vi "BIMS_Collector (BRZ).vi"() -> ()   [LabVIEW 2015]
doc: "This program is currently beta software. It is designed to address the data requirements defined primarily by the DHB Ballistic Test Report.\n\nThe general operation of this program is based on the Ballistics Version 2005 application developed internally by DuPont as a research tool for the Spruance Plant Ballistics Lab in Richmond, VA.\n\nPlease note that the original trigger control logic was modified and no longer depends on a safety interlock system to enable operation of a ballistic test.\n\nDuPont makes no warranties and assumes no liabilities in connection with any use of this program."
uses:
  <vilib>/addons/database/NI_Database_API.lvlib
  <vilib>/addons/database/Connection.llb/Conn Execute.vi
  <vilib>/addons/database/Recordset.llb/Rec Destroy - Connection.vi
  <vilib>/Utility/config.llb/NI_LVConfig.lvlib
  <vilib>/Utility/config.llb/Write Key (I32).vi
  Shot Record.ctl
  BIMS_Collector Globals.vi
  Collector State.ctl
  DataSource.ctl
  <vilib>/registry/registry.llb/Registry RtKey.ctl
  <vilib>/Utility/config.llb/Write Key (String).vi
  <vilib>/addons/database/Connection.llb/DB Tools Open Connec (Path).vi
panel:
  out "Loading":u16(ring)
  in  "runtimeMenusVisible":bool=TRUE
  in  "diagPageVisible":bool
  in  "RESET All":bool
  out "ConfigName":string
  out "TimeNow":string
  in  "EXIT":bool
  in  "mainTabCntrl":enum32{"Setup", "Measure", "History", "System"}(tab)=enum."System"
  in  "SampleEntryTabCntrl":enum32{"Environment", "Sample"}(tab)
  in  "ThreatDetails":u16(ring) caption="Detail" items=["2gr 223 cal.   FSP", "4gr 223 cal.   FSP", "16gr 223 cal."]
  in  "ThreatGroups":u16(ring) caption="Group" items=["", "RCC", "FSP", "44 Magnum", "0.22 Caliber", "0.380 Caliber", "0.38 Caliber", "9mm Luger", "40 S&W", "0.357 MAG", "0.44 Rem Mag"]
  in  "PowderTypes":u16(ring) caption="Type" items=["", "CBC 236", "CBC 210", "CBC 220", "CBC 216", "CBC 207", "CBC PCL 504"]
  in  "Ballisticians":u16(ring) caption="Laboratorists" items=["", "Gustavo M Rubio", "Manoel Machado", "Lucas Loureiro", "Outros (others)"]
  in  "Recorders":u16(ring) caption="Recorder"
  in  "Shooters":u16(ring) caption="Shooter" items=["", "Manoel C. Machado                                 ", "Gustavo M Rubio                                   ", "Assef Maluf                                       "]
  in  "Methods":u16(ring) caption="Method" items=["", "V50", "NIJ 0101.04", "NIJ 0101.06", "NIJ 0108.01", "Helmets", "Others"]
  in  "RoomT":sgl caption="Temperature (° C)" format="%.1f"
  in  "RoomHum":sgl caption="Humidity (%)" min=0 max=100 format="%.1f"
  in  "SampleBackings":u16(ring)=3 caption="Type" items=["", "Clay", "Roma Clay", "Corfix Clay", "Dim Clay"]
  in  "clayCalArray":i16[](array[numeric])=[0, 0, 0, 0, 0] caption="Calibration (mm)" min=0 max=99 format="%02.0f"
  out "clayAverage":sgl caption="Clay Average (mm)" format="%#.1f"
  in  "clayTemp":sgl caption="Clay Temp (° F)" format="%.1f"
  out "threatDetails":T1 caption="Description"
  in  "SampleClamping":u16(ring) caption="Clamping" items=["", "elástic with Velcro", "screws", "rubber tube", "anti spall ", "box against fragments"]
  in  "Sample SubTabCntrl":T2(tab)
  in  "SampleID":string caption="Sample ID"
  in  "SampleDimensions":u16(ring) caption="Dimensions" items=["", "40 x 40", "50 x 50", "P", "M", "G", "GG", "Car Part", "Indefinite"]
  in  "ModelMfrs":u16(ring) caption="Manufacturer" items=["DuPont Experimental"]
  in  "SampleTypes":u16(ring) caption="Sample Type" items=["", "Aramid", "Glass", "Steel", "Ceramic", "Panel", "Body Armor", "Car Parts", "Quality Control", "Helmets", "Shield", "Other"]
  in  "Submitters":u16(ring) caption="Submitter" items=["", "Ana P Viegas", "Julio Tabegna", "Priscila Akiti", "Ariana Bottura", "Carlos Magno", "Rodrigo Gomez", "Angela C Vargas", "Manoel Machado", "Others"]
  in  "ProjectID":string caption="Project ID"
  in  "BackLayers":i32 caption="# of Layers" min=0 max=99 step=5
  in  "FrontLayers":i32 caption="# of Layers" min=0 max=99 step=5
  in  "BackLayer":u16(ring) caption="Back Layer" items=["", "PC", "Steel", "PE Foam", "Ghost", "ceramic plate", "Others"]
  in  "FrontLayer":u16(ring) caption="Front Layer" items=["", "PC", "Steel", "PE Foam", "Ghost", "ceramic plate", "Others"]
  out "totalNumLayers":i32 caption="Total # of Layers" min=0 max=100 step=5
  out "totalBAW":sgl caption="Total BAW (psf)" format="%.2f"
  in  "LayerTabControl":enum32{"1", "2", "3", "4", "5", "6"}(tab) caption="Inner Layers"
  out "fab1_totalWt":sgl caption="Fab1 Wt" min=0 max=99 step=5 format="%.2f"
  out "SampleAttribs_1":T3 caption="fabricAttribs_1"
  in  "Layer_1":T4 caption="Fabric #1" {"plyNum" min=0 max=99 step=5}
  in  "SampleStyle_1":u16(ring) items=["", "S363 GR", "S363 WR", "S436 GR", "S436 WR", "S704 GR", "S704 WR", "S708 GR", "S708 WR", "S720", "S720 GR", "S720 WR", "S724 GR", "S729 GR", "S729 WR", "S731 GR", "S731 WR", "S745 GR", "S745 WR", "S745GR", "S745GR-1", "S778 GR", "S778 WR", "XF", "XP1000"]
  in  "Mfr_1":u16(ring) caption="vendor" items=["", "Assef Maluf", "DuPont", "DuPont Cooper River", "TEADIT", "TestBob1"]
  in  "layerStitch_1":u16(ring) caption="Stitch" items=["", "Diamante (diamond)", "Cantos vertices (corners vertices)", "Cantos centrais (corners centrals)", "Borda e Centro (all around and center)", "Borda (all around)", "Borda e diamante (all around and diamond)", "Dupla em X (double and X centered)", "Outras (others)"]
  out "fab2_totalWt":sgl caption="Fab2 Wt" min=0 max=99 step=5 format="%.2f"
  out "SampleAttribs_2":T3 caption="fabricAttribs_2"
  in  "Layer_2":T4 caption="Fabric #2" {"plyNum" min=0 max=99 step=5}
  in  "SampleStyle_2":u16(ring)
  in  "Mfr_2":u16(ring) caption="vendor" items=["", "Assef Maluf", "DuPont", "DuPont Cooper River", "TEADIT", "TestBob1"]
  in  "layerStitch_2":u16(ring) caption="Stitch" items=["", "Diamante (diamond)", "Cantos vertices (corners vertices)", "Cantos centrais (corners centrals)", "Borda e Centro (all around and center)", "Borda (all around)", "Borda e diamante (all around and diamond)", "Dupla em X (double and X centered)", "Outras (others)"]
  out "fab3_totalWt":sgl caption="Fab3 Wt" min=0 max=99 step=5 format="%.2f"
  out "SampleAttribs_3":T3 caption="fabricAttribs_3"
  in  "Layer_3":T4 caption="Fabric #3" {"plyNum" min=0 max=99 step=5}
  in  "SampleStyle_3":u16(ring)
  in  "Mfr_3":u16(ring) caption="vendor" items=["", "Assef Maluf", "DuPont", "DuPont Cooper River", "TEADIT", "TestBob1"]
  in  "layerStitch_3":u16(ring) caption="Stitch" items=["", "Diamante (diamond)", "Cantos vertices (corners vertices)", "Cantos centrais (corners centrals)", "Borda e Centro (all around and center)", "Borda (all around)", "Borda e diamante (all around and diamond)", "Dupla em X (double and X centered)", "Outras (others)"]
  out "fab4_totalWt":sgl caption="Fab4 Wt" min=0 max=99 step=5 format="%.2f"
  out "SampleAttribs_4":T3 caption="fabricAttribs_4"
  in  "Layer_4":T4 caption="Fabric #4" {"plyNum" min=0 max=99 step=5}
  in  "SampleStyle_4":u16(ring)
  in  "Mfr_4":u16(ring) caption="vendor" items=["", "Assef Maluf", "DuPont", "DuPont Cooper River", "TEADIT", "TestBob1"]
  in  "layerStitch_4":u16(ring) caption="Stitch" items=["", "Diamante (diamond)", "Cantos vertices (corners vertices)", "Cantos centrais (corners centrals)", "Borda e Centro (all around and center)", "Borda (all around)", "Borda e diamante (all around and diamond)", "Dupla em X (double and X centered)", "Outras (others)"]
  out "fab5_totalWt":sgl caption="Fab5 Wt" min=0 max=99 step=5 format="%.2f"
  out "SampleAttribs_5":T3 caption="fabricAttribs_5"
  in  "Layer_5":T4 caption="Fabric #5" {"plyNum" min=0 max=99 step=5}
  in  "SampleStyle_5":u16(ring)
  in  "Mfr_5":u16(ring) caption="vendor" items=["", "Assef Maluf", "DuPont", "DuPont Cooper River", "TEADIT", "TestBob1"]
  in  "layerStitch_5":u16(ring) caption="Stitch" items=["", "Diamante (diamond)", "Cantos vertices (corners vertices)", "Cantos centrais (corners centrals)", "Borda e Centro (all around and center)", "Borda (all around)", "Borda e diamante (all around and diamond)", "Dupla em X (double and X centered)", "Outras (others)"]
  out "fab6_totalWt":sgl caption="Fab6 Wt" min=0 max=99 step=5 format="%.2f"
  out "SampleAttribs_6":T3 caption="fabricAttribs_6"
  in  "Layer_6":T4 caption="Fabric #6" {"plyNum" min=0 max=99 step=5}
  in  "SampleStyle_6":u16(ring)
  in  "Mfr_6":u16(ring) caption="vendor" items=["", "Assef Maluf", "DuPont", "DuPont Cooper River", "TEADIT", "TestBob1"]
  in  "layerStitch_6":u16(ring) caption="Stitch" items=["", "Diamante (diamond)", "Cantos vertices (corners vertices)", "Cantos centrais (corners centrals)", "Borda e Centro (all around and center)", "Borda (all around)", "Borda e diamante (all around and diamond)", "Dupla em X (double and X centered)", "Outras (others)"]
  in  "SampleCoverings":u16(ring) caption="Sample Covering" items=["None", "RipStop", "Plastic bag", "Other"]
  in  "Assemblers":u16(ring) caption="Technician" items=["", "Gustavo M Rubio", "Lucas Loureiro", "Manoel Machado", "Assef Maluf", "Client", "Tecidos Especiales", "Others"]
  in  "Thickness":dbl caption="Thickness (in)" format="%.3f"
  in  "totalSampleWt":sgl caption="Total Weight (lbs)" format="%.3f"
  in  "Comments":string caption="Remarks (optional):"
  in  "TestConditions":u16(ring) caption="Sample Condition" items=["", "Dry", "Wet", "T & H Controlled", "After Tumbling", "Heated", "Cooled"]
  in  "shotsTabCntrl":T5(tab)
  in  "2ndScreen":bool=TRUE caption="Enabled"
  in  "Frag Rod":sgl format="%.1f"
  in  "MeasSrc":T6=enum."Screens" caption="Source"
  in  "Drag Corrected":bool=TRUE
  in  "ARM":bool
  in  "readyClock":bool caption="Clock"
  out "Impact/speed":sgl caption="Chronograph 1" min=0 max=10000 step=0.1 format="%.1f"
  out "SHOT STATUS":u16(ring) caption="Penetration" items=["Partial", "Complete"]
  out "residual/speed":sgl caption="Residual" min=0 max=10000 step=0.1 format="%.1f"
  out "SUBMIT DATE/TIME":string
  out "BACKFACE DEPTH":sgl caption="Backface\nDepth" min=0 max=200 step=5
  in  "MeasVelScrnSet1":sgl caption="Set #1" min=0 max=10000 step=0.1 format="%.1f"
  in  "Current/sthotstatus":u16(ring) caption="Penetration" items=["Partial", "Complete"]
  in  "Current/residual/speed":sgl caption="Residual Set" min=0 max=10000 step=0.1 format="%.1f"
  in  "currentDateTime":string caption="Date/Time"
  in  "MeasVelScrnSet2":sgl caption="Set #2" min=0 max=1000000 step=0.1 format="%.1f"
  out "%_Difference":sgl caption="% Vel Diff" format="%.3f"
  in  "backdepth":sgl caption="BF Depth"
  out "Redundant/speed":sgl caption="Chronograph 2" min=0 max=10000 step=0.1 format="%.1f"
  out "Current/avg/speed":sgl caption="Average" min=0 max=1000000 step=0.1 format="%.1f"
  out "Avg/speed":sgl caption="Average" min=0 max=10000 step=0.1 format="%.1f"
  out "SafetyInterlock":cluster{"ARMED":bool}
  out "DC_ factor":sgl=1.0 caption="DC Factor" format="%.4f"
  in  "Barrel Temp":sgl format="%.1f"
  in  "Shot Description":string caption="Description (optional)"
  in  "Powder Loading":sgl caption="Powder Load" min=0 max=100 step=0.1 format="%.3f"
  in  "Shot Angle":u16 max=90 step=1
  out "Projectile Mass":sgl caption="Projectile Mass (grains)" min=0 step=1
  in  "N.I.J":u16(ring) items=["n/a", "PASS", "FAIL"]
  out "Device S/N":string
  in  "addShot":bool caption="RANGE SETUP must be selected before shots can be added."
  in  "loadingUnits":enum32{"grams", "grains"}(radio)
  out "instruct_addShot":string="RANGE SETUP and THREAT must be selected before shots can be added."
  out "Set#1 Separation":sgl=1.0 caption="Outer" format="%.2f"
  out "Set#2 Separation":sgl=1.0 caption="Inner" format="%.2f"
  out "velSTDEV":sgl caption="Standard Deviation" min=0 max=10000 step=1 format="%.1f"
  out "saveReq":string="Number of layers in sample ply specification and number of shots in shots table must be greater than 0 to enable saving."
  in  "VsVr Report":bool caption="Report"
  out "Table of Shots":string[][](table) caption="Shot Table"
  in  "MC Listbox of Shots":i32(listbox)
  in  "saveShots":bool
  in  "clearShots":bool
  out "highPartial":i32 caption="High Partial" min=0 max=10000 step=1
  out "lowComplete":i32 caption="Low Complete" min=0 max=10000 step=1
  out "rangeOfResults":i32 caption="Range of Results" min=0 max=10000 step=1
  out "zmr 2":sgl caption="Low C minus High P" format="%.1f"
  out "computed_V50":sgl caption="V50  (m/s)" format="%.1f"
  out "Pairs":i16 min=0 max=100 step=1
  in  "reportV50":bool caption="Report"
  in  "maxDev":sgl=10.0 caption="Max Deviation (m/s)" min=0 max=100 format="%.1f"
  in  "undoLastShot":bool
  in  "deleteShot":bool
  in  "nextShot":bool
  in  "SHOTS":T7[](array[typedef]) {"Frag Rod" format="%.1f"; "UncorrectedAvgVel_PB" format="%.1f"; "UncorrectedRed_PB" format="%.1f"; "strikeVel_PB" format="%.1f"; "velLoss_PB" format="%.1f"; "avgVel_PB" format="%.1f"; "Redundant_Velocity" format="%.1f"; "Energy Loss (J)" format="%.3e"; "Projectile Mass" min=0 step=1 format="%.4f"; "Corrected residual" format="%.2f"; "Uncorrected Residual" format="%.1f"; "Corrected Impact" format="%.2f"; "Uncorrected Impact" format="%.1f"; "Shot Angle" max=90 step=1; "SHOT STATUS" items=["Partial", "Complete"]; "IMPACT VELOCITY" min=0 max=10000 step=0.1 format="%.1f"; "Barrel Temperature" format="%.1f"; "Powder Loading" format="%.4f"; "RESIDUAL  VELOCITY" min=0 max=10000 step=0.1 format="%.1f"}
  out "velProfile":cluster{dbl, dbl}[](graph) caption="Shot Velocity Measurement Profile"
  out "velCompProf":cluster{"vStrike":dbl, "vA":dbl} caption="Velocity in fps\n(computed)"
  out "velMeasProf":T8 caption="Velocity in fps\n(measured)"
  out "relativeTime":cluster{"ts2":dbl, "ts3":dbl, "ts1":dbl} caption="Relative time\n(microsec)"
  out "displacement":T9={"ds_v2"=6.75, "ds2"=5.0833, "ds_vB"=4.9167, "ds3"=4.75, "ds_vAvg"=6.9167, "ds_v1"=7.0833, "ds1"=8.75, "ds_vA"=8.9167, "ds0"=9.0833} caption="Distance from\ntarget (ft)" {"ds0" format="%_4g"; "ds_vA" format="%_4g"; "ds1" format="%_4g"; "ds_v1" format="%_4g"; "ds_vAvg" format="%_4g"; "ds3" format="%_4g"; "ds_vB" format="%#_4g"; "ds2" format="%#_4g"; "ds_v2" format="%_4g"}
  out "arrIDC":dbl[](array[numeric]) caption="Instantaneous Drag Coefficient"
  in  "rangeSetup":u16(ring)=1 caption="Range Dimensions" items=["Short (small frag)", "Standard (handgun)", "Long (rifle)"]
  out "mid_to_targ_dist":sgl=5.0 caption="Mid To Target (ft)"
  in  "historyTabCntrl":enum32{"Powder Loading", "Panel Search"}(tab)=enum."Panel Search"
  in  "Threat.freeTxt":string caption="Threat"
  in  "Powder.freeTxt":string caption="Powder"
  in  "QueryLoad":bool
  in  "lkupEndDate":timestamp caption="End Date" format="%<%x>T"
  in  "lkupStartDate":timestamp caption="Begin Date" format="%<%x>T"
  out "Vel.vs.Loading":cluster{dbl[], dbl[]}(graph)
  out "v50_table":string[][](table)
  in  "maxRecs":u16=1001 caption="Max # of SHOT Records" min=1 max=10000 step=100
  out "ActualNumRecs":i32=1001 caption="Actual # Returned"
  in  "ThreatSize_0":u16(ring) caption="Threat Size" items=["", "2", "4", "16", "17", "33", "40", "44", "85", "95", "124", "125", "158", "180", "240"]
  in  "panelSearch":bool
  in  "Mfr_0":u16(ring) caption="Manufacturer" items=["", "Assef Maluf", "DuPont", "DuPont Cooper River", "TEADIT", "TestBob1"]
  in  "SampleStyle_0":u16(ring) caption="Sample Style"
  in  "srchParams":T10={"maxPanels"=1001, "lkupPanelStartDate"=timestamp(0 s since 1904-01-01), "lkupPanelEndDate"=timestamp(3376658114.0909824 s since 1904-01-01)} {"lkupPanelEndDate" format="%<%x>T"; "lkupPanelStartDate" format="%<%x>T"; "maxPanels" min=1 max=10000 step=100}
  out "actualNumPanels":i32 caption="Actual # Returned"
  out "pastPanels":string[][](table)
  in  "Record #":i32=1 min=0 max=48
  in  "reportV50_History":bool
  out "SampleAttribs_0":T11 caption="fabricAttribs_1"
  in  "Requestors_0":u16(ring) caption="Submitter" items=["", "Ana P Viegas", "Angela C Vargas", "Ariana Bottura", "Carlos Magno", "Julio Tabegna", "Manoel Machado", "Others", "Priscila Akiti", "Rodrigo Gomez"]
  in  "aboutTabCntrl":T12(tab)
  in  "RefreshMetadata":bool
  out "LastShot":i32 caption="Shot"
  out "LastSample":i32 caption="Sample"
  in  "PublishNewRecords":bool
  in  "Folder":string="esvrs11" caption="Publish Folder"
  in  "clearErrors":bool
  in  "useBMC":bool caption="Use Message Center?"
  in  "Server":string="esvrs11"
  in  "Site":string="ICE1"
  in  "TestStandards":u16(ring)=2 caption="Standard" items=["n/a", "NIJ 0101.04", "MIL-STD-662F"]
  in  "WeaponTypes":u16(ring) caption="Weapon" items=["", "Universal Receiver", "Other"]
  in  "processShots":bool
  out "DIO":u32=21 format="%.0b"
  in  "line direction map":i32=1792 format="%.0b"
  out "Corrected Average":sgl=1527.9313 format="%.2f"
  out "CorrectedVelScrnSet2":sgl=1551.8816 caption="Corrected Redundant" format="%.2f"
  out "conversion factor":sgl=0.3048037 format="%.5f"
  out "#_completes":i32
  out "#_partials":i32
  in  "percent warning":sgl=1.0 format="%.2f"
  in  "SoftwareVersion":dbl caption="Version" format="%.2f"
  out "impact/ID":u32=83886081 format="%.0x"
  out "residual/ID":u32=83951617 format="%.0x"
  out "Red/ID":u32=84017153 format="%.0x"
  out "correction coefficient":sgl format="%.8f"
  out "Corrected Residual":sgl=751.9905 format="%.2f"
  out "CorrectedVelScrnSet1":sgl=1503.981 format="%.2f"
  out "Barrel to Screen":sgl=7.8333 format="%.2f"
  in  "Set#1_to_Target":sgl=7.083333 format="%.2f"
  out "Residual/Separation":sgl=4.0 format="%.2f"
  in  "Residual/Target Dist":sgl=7.083333 format="%.2f"
  out "Z.M.R.":sgl min=0 step=0.1 format="%.1f"
  in  "old threat":u16
  out "Complete":sgl[](array[numeric]) format="%.2f"
  out "factor array":sgl[](array[numeric]) format="%.4f"
  out "Partial":sgl[](array[numeric]) format="%.2f"
  in  "DAQ Card":i16=1
  in  "Impact Timer":i16 min=0 max=3 step=1
  in  "Redundant Timer":i16=1 min=0 max=3 step=1
  in  "Residual  Timer":i16=2 min=0 max=3 step=1
  out "Impact factor":sgl=1.0 caption="Impact" min=0 max=1 format="%.5f"
  out "Residual factor":sgl=1.0 caption="Residual" min=0 max=1 format="%.5f"
  in  "Areal Density":dbl format="%.2f"
  in  "Areal density text":string
  in  "Fabric Description":string caption="Fabric Desc"
  in  "clayCalib":string="##-##-##-##-##" caption="Calibration"
  in  "lookupRec":bool caption="lookup"
  out "STOP (Shots MC LB)":bool=TRUE
  out "configPath":path=path "P:/Private/My Projects/AFS/BIMS/2008/BIMS_Collector.ini" caption="Configuration Path (INI)"
  in  "minV50":i32=450 caption="Minimum V50"
  in  "Type of work":string="QC"
  in  "Threat":u16(ring) caption="Threat (long description)"
  out "massUnits":string="GRAMS" caption="Weight Units"
  out "lengthUnits":string="FOOT" caption="Distance Units"
  in  "SampleDescrip":u16(ring) caption="Misc. Sample Description (legacy)"
  in  "serialNum":string caption="Serial #"
  in  "Models":u16(ring) caption="Model #" items=["n/a"]
  in  "InterlockExists":bool=TRUE caption="Safety Interlock Hardware Exist?"
  in  "ScreenSetAvgg":bool caption="Average Screen Sets?"
  in  "Sort by AVG":bool=TRUE caption="Sort shots by average velocity"
  in  "useBallisitican":bool=TRUE caption="Use Ballistician field in Setup?"
  in  "useRecorder":bool caption="Use Recorder field in Setup?"
  in  "useShooter":bool caption="Use Shooter field in Setup?"
  out "SMErr":errorcluster
  out "U/I EvErr":errorcluster
  out "booleanDump":bool
  out "GrainSize":u16 caption="Grain"
  in  "LayerStitchTypes":u16(ring) caption="Stitch" items=["", "Corners"]
  # "Effectively restarts the application from scratch, as if the user pressed the EXIT button and then restarted the application."
  # "Configured for"
  # "Threat"
  # "*"
  # "*"
  # "Test"
  # "Powder"
  # "*"
  # "Personnel"
  # "Room"
  # "*"
  # "Backing"
  # "*"
  # "*"
  # "*"
  # "Body Side"
  # "Strike Face"
  # "Layer"
  # "Mfr"
  # "Style"
  # "# of Plies"
  # "Lot"
  # "Roll"
  # "Stitch"
  # "Internal ID"
  # "Fiber"
  # "Denier"
  # "Construction"
  # "Weave"
  # "Finish"
  # "Basis weight (oz/yd²)"
  # "Yarn Merge"
  # "Total Weight"
  # "*"
  # "*"
  # "*"
  # "1"
  # "2"
  # "3"
  # "4"
  # "5"
  # "6"
  # "Required"
  # "*"
  # "Timing System"
  # "Shot Parameters"
  # "cm"
  # "deg"
  # "° C"
  # "Velocity Measurements"
  # "Observations"
  # "Screens\nSeparation"
  # "meters"
  # "Table Functions"
  # "Summary"
  # "Reports"
  # "Test Record"
  # "Edit Shot Records"
  # "Corrected"
  # "Shot #"
  # "t0"
  # "0"
  # "S Strike"
  # "0"
  # "Internal ID#"
  # "Fiber"
  # "Denier"
  # "Pick"
  # "Weave"
  # "Finish"
  # "oz/yd²"
  # "Asset"
  # "DuPont Ballistics Information Management System\n\nBIMS\nEnterprise Edition\n\n\nSample Performance\nData Collector\n\nApril 2012"
  # "DuET Measurement System Technologies\nDUCOM 8 695-2330 for technical support\n\nDuPont Company"
  # "Last Assigned\nRecord Numbers"
  # "Deployment Configuration"
  # "Data items support Point Blank requirements:"
  # "Correction Factors"
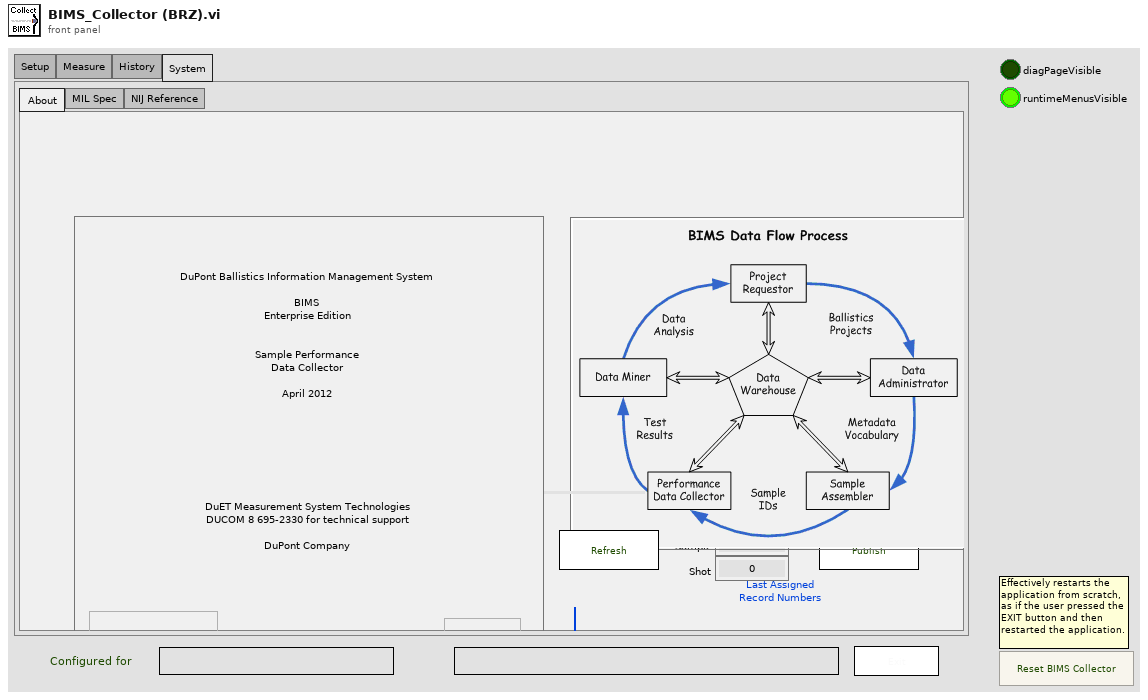
[diagram p1: front panel]
types:
  T1 = cluster{"barrelLength":string, "dragCorrection":string, "detailDescription":string, "barrelCaliber":string, "grainSize":string, "Make":string, "Model":string}
  T2 = enum32{"General Specification", "Ply Specification", "Preparation"}
  T3 = cluster{"Fabric.fiber":string, "Fabric.denier":string, "pick":string, "weave":string, "finish":string, "ozPerYd2":string, "fabricID_DHB":string, "yarnMerge":string}
  T4 = cluster{"plyNum":i32, "LotNum":string, "RollNum":string}
  T5 = enum32{"Ready-Aim-Fire", "Shots Table", "Edit", "Instantaneous DC"}
  T6 = typedef "DataSource.ctl" = enum16{"Simulated", "Radar", "Screens"}
  T7 = typedef "Shot Record.ctl" = cluster{"Uncorrected Impact":sgl, "Uncorrected Residual":sgl, "avgVel_PB":sgl, "IMPACT VELOCITY":sgl, "RESIDUAL  VELOCITY ":sgl, "Shot Description":string, "Powder Loading ":sgl, "Barrel Temperature":sgl, "TIME / DATE":string, "shot order":i32, "SHOT STATUS":u16, "Shot Angle":u16, "Corrected Impact":sgl, "Corrected residual":sgl, "Projectile Mass":sgl, "usedv50":bool, "Energy Loss (J)":sgl, "BackFace\nDepth":sgl, "BackFace\nDiameter":sgl, "Redundant_Velocity":sgl, "velLoss_PB":sgl, "strikeVel_PB":sgl, "UncorrectedRed_PB":sgl, "CorrectedRed_PB":sgl, "UncorrectedAvgVel_PB":sgl, "V50userExcl":bool, "Frag Rod":sgl}
  T8 = cluster{"v2":dbl, "vB":dbl, "vOuter":dbl, "v1":dbl, "vA":dbl, "vInner":dbl}
  T9 = cluster{"ds_v2":dbl, "ds2":dbl, "ds_vB":dbl, "ds3":dbl, "ds_vAvg":dbl, "ds_v1":dbl, "ds1":dbl, "ds_vA":dbl, "ds0":dbl}
  T10 = cluster{"maxPanels":u16, "lkupPanelStartDate":timestamp, "lkupPanelEndDate":timestamp}
  T11 = cluster{"Fabric.fiber":string, "Fabric.denier":string, "pick":string, "weave":string, "finish":string, "ozPerYd2":string, "fabricID_DHB":string, "asset":string}
  T12 = enum32{"About ", "MIL Spec", "NIJ Reference", "Internal Use"}
  T13 = typedef "Collector State.ctl" = enum16{"POLL", "INITIALIZE", "V50 Report or GET Record", "VsVr Report", "SAVE SHOTS", "ADD SHOT", "CLEAR SHOTS", "NEXT SHOT", "DELETE SHOT", "READY CLOCK", "PROC SHOTS", "CHECK DAQ"}
  T14 = typedef "Collector State.ctl" = enum16{"POLL", "INITIALIZE", "V50 Report or GET Record", "VsVr Report", "SAVE SHOTS", "ADD SHOT", "CLEAR SHOTS", "NEXT SHOT", "DELETE SHOT", "PROCESS SHOTS", "READY CLOCK", "CHECK DAQ"}
  T15 = enum8{"Enabled", "Disabled", "Disabled and Grayed Out"}
  T16 = enum32{"Page Enabled", "Page Disabled", "Page Disabled & Grayed"}
  T17 = typedef "Registry RtKey.ctl" = enum32{"HKEY_CLASSES_ROOT", "HKEY_CURRENT_USER", "HKEY_LOCAL_MACHINE", "HKEY_USERS", "HKEY_PERFORMANCE_DATA", "HKEY_CURRENT_CONFIG", "HKEY_DYN_DATA"}
  T18 = cluster{"[0]":string, "[1]":string, "[2]":string, "[3]":string, "[4]":string, "[5]":string, "[6]":string, "[7]":string, "[8]":string, "[9]":string}[]
  T19 = cluster{"[0]":string, "[1]":string, "[2]":string, "[3]":string, "[4]":string, "[5]":string, "[6]":string, "[7]":string, "[8]":string}[]
  T20 = cluster{"Fabric.fiber":string, "Fabric.denier":string, "pick":string, "weave":string, "finish":string, "ozPerYd2":string, "fabricID_DHB":string, "yarnMerge":string}[]
  T21 = cluster{"Uncorrected Impact":bool, "Uncorrected Residual":bool, "avgVel_PB":bool, "IMPACT VELOCITY":bool, "RESIDUAL  VELOCITY ":bool, "Shot Description":bool, "Powder Loading ":bool, "Barrel Temperature":bool, "TIME / DATE":bool, "shot order":bool, "SHOT STATUS":bool, "Shot Angle":bool, "Corrected Impact":bool, "Corrected residual":bool, "Projectile Mass":bool, "usedv50":bool, "Energy Loss (J)":bool, "BackFace\nDepth":bool, "BackFace\nDiameter":bool, "Redundant_Velocity":bool, "velLoss_PB":bool, "strikeVel_PB":bool, "UncorrectedRed_PB":bool, "CorrectedRed_PB":bool, "UncorrectedAvgVel_PB":bool, "V50userExcl":bool, "Frag Rod":bool}
  T22 = cluster{"SampleTypes":refnum<vi>, "SampleDescrip":refnum<vi>}
  T23 = cluster{"max dev":sgl, "residual separation":sgl, "Set#1 Separation":sgl, "Set#2 Separation ":sgl, "impact target dist":sgl, "resid target dist":sgl, "barrel screen dist":sgl, "midpt_to_target_dist":sgl}
  T24 = cluster{"fiber":string, "denier":string, "pick":string, "weave":string, "finish":string, "ozPerYd2":string, "internal_ID":string, "asset":string}[]
  T25 = cluster{"numOfPlies":i32, "LotNum":string, "RollNum":string}[]
  T26 = cluster{string, string, string, string, string, string, string, string, "clayCalib":string, string}
  T27 = cluster{string, string, string, string, string, string, string}
  T28 = cluster{"SampleID":string, "element":string, "Type of work":string, "serialNum":string, "element":string, string, string, string, "element":string, string}
  T29 = cluster{"SampleID":string, "element":string, string, string, string, "element":string}
  T30 = cluster{"[0]":string, "[1]":string, "[2]":string, "[3]":string, "[4]":string, "[5]":string, "[6]":string, "[7]":string, "[8]":string, "[9]":string}
  T31 = cluster{"[0]":string, "[1]":string, "[2]":string, "[3]":string, "[4]":string, "[5]":string, "[6]":string, "[7]":string, "[8]":string}
  T32 = cluster{"element":string, "element":string, "grainSize":string, "element":string, "barrelLength":string, string, "element":string, "element":string, "element":string}
  T33 = cluster{"element":string, "grainSize":string, "element":string, "barrelLength":string, string, "element":string}
  T34 = typedef "NI_Database_API.lvlib/Conn ObjectReference.ctl" = refnum<k1>
  T35 = typedef "NI_Database_API.lvlib/Rec ObjectReference.ctl" = refnum<k1>
  T36 = typedef "NI_LVConfig.lvlib/Config Data RefNum.ctl" = refnum<k1>
  T37 = cluster{"task ID out":u32, "task ID out":u32, "task ID out":u32}
  T38 = enum32{"invalid app kind", "Development System", "Run Time System", "Student Edition", "Embedded LabVIEW", "Evaluation", "Custom"}
  T39 = typedef "LVRowAndColumnTypeDef.ctl" = cluster{"Row":i32, "Column":i32}
  T40 = cluster{"barrelLength":string, "dragCoefficient":string, "detailDescription":string, "barrelCaliber":string, "grainSize":string, "Make":string, "Model":string}
  T41 = cluster{"fiber":string, "denier":string, "construction":string, "weave":string, "finish":string, "ozPerYd2":string, "fabricStyle_DHB":string, "yarnMerge":string}
  T42 = cluster{"plyNum":i32, "LotNum":string, "RollNum":string}[]
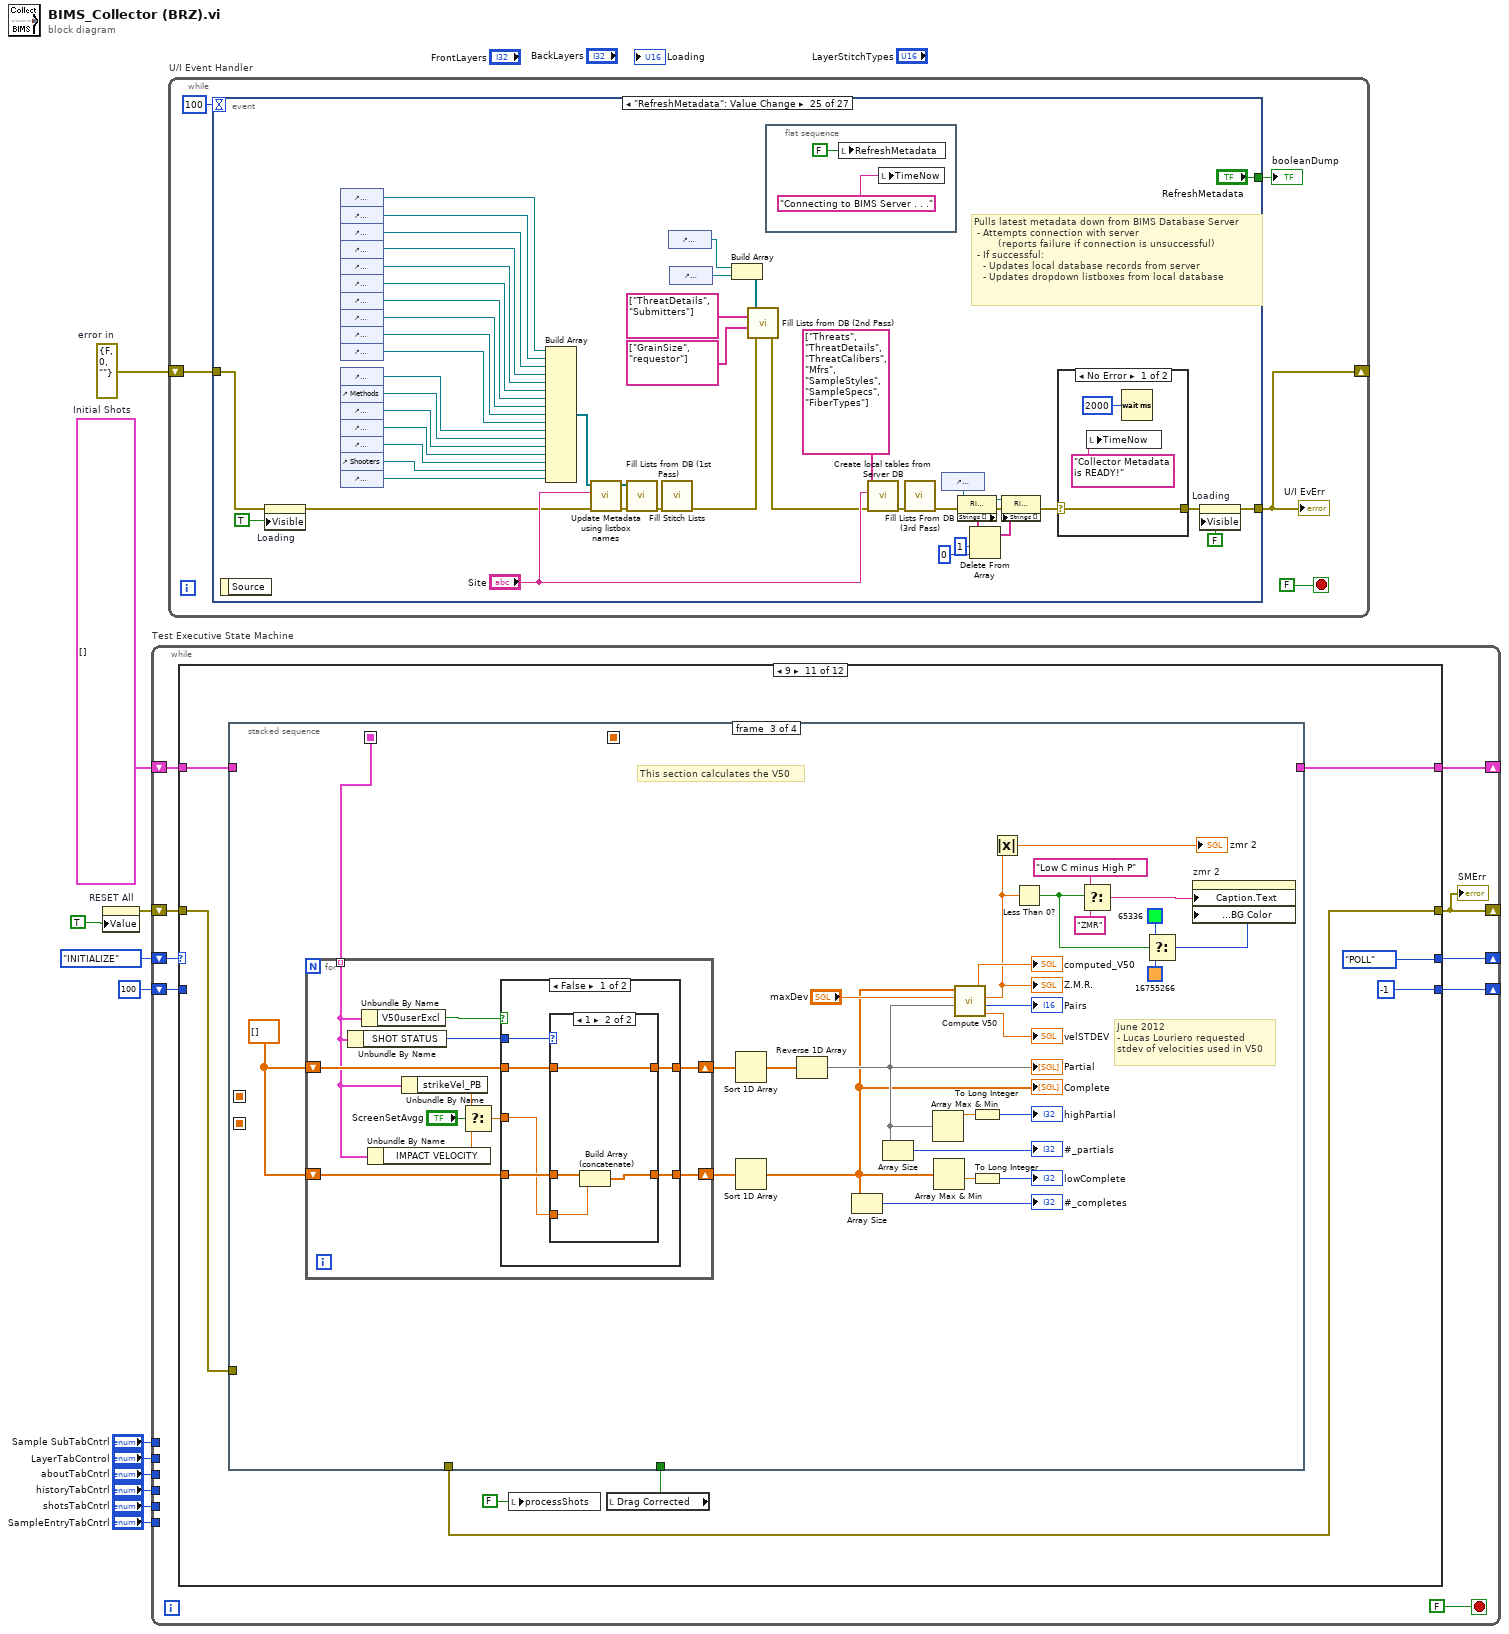
[diagram p0: block diagram]
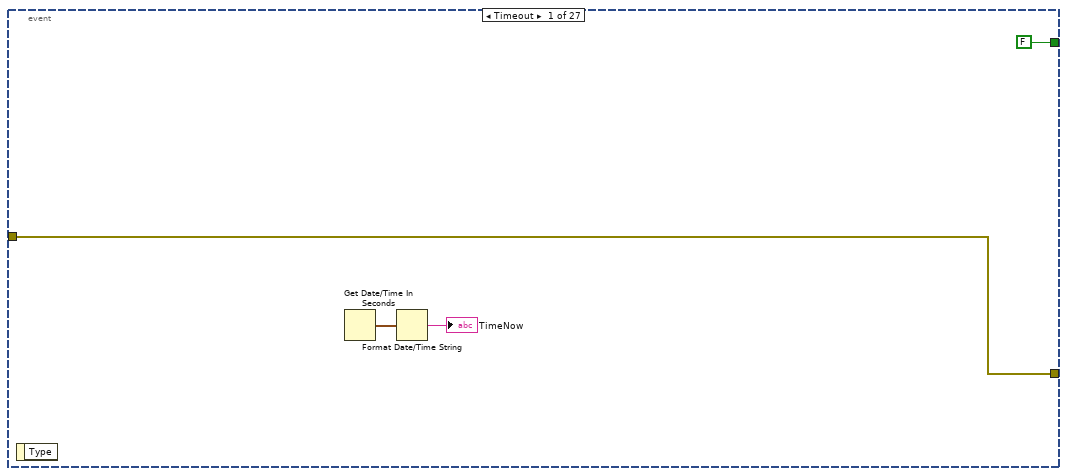
[diagram p2: hidden frame]
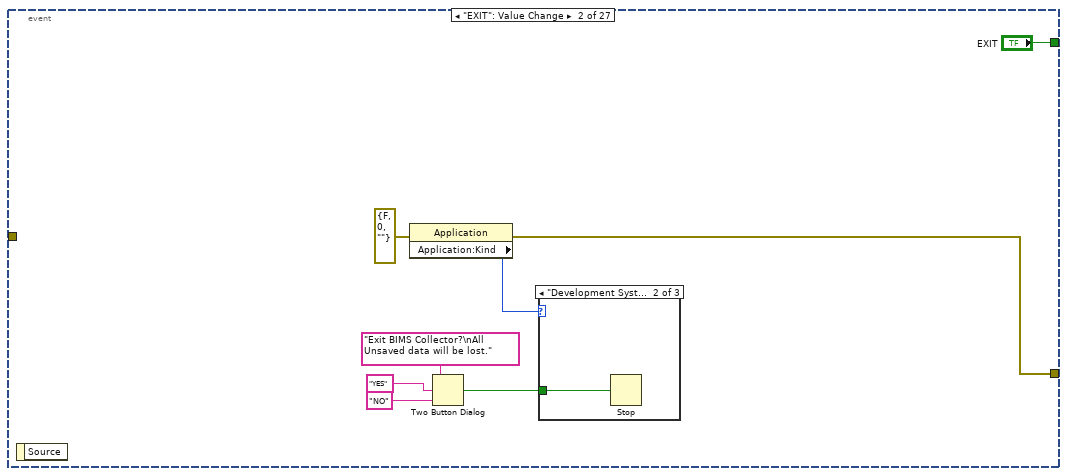
[diagram p3: hidden frame]
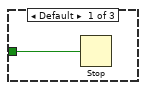
[diagram p4: hidden frame]
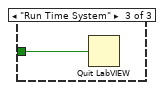
[diagram p5: hidden frame]
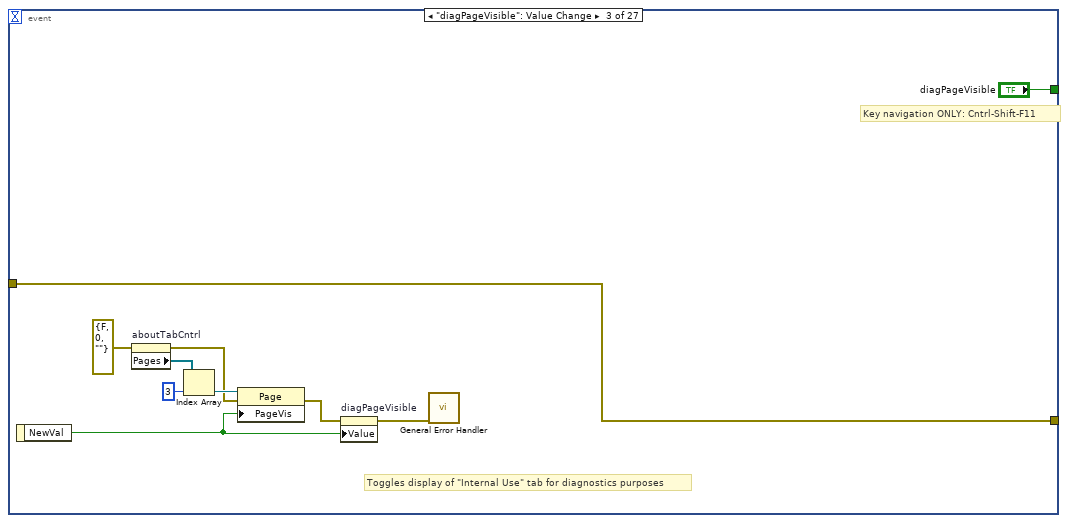
[diagram p6: hidden frame]
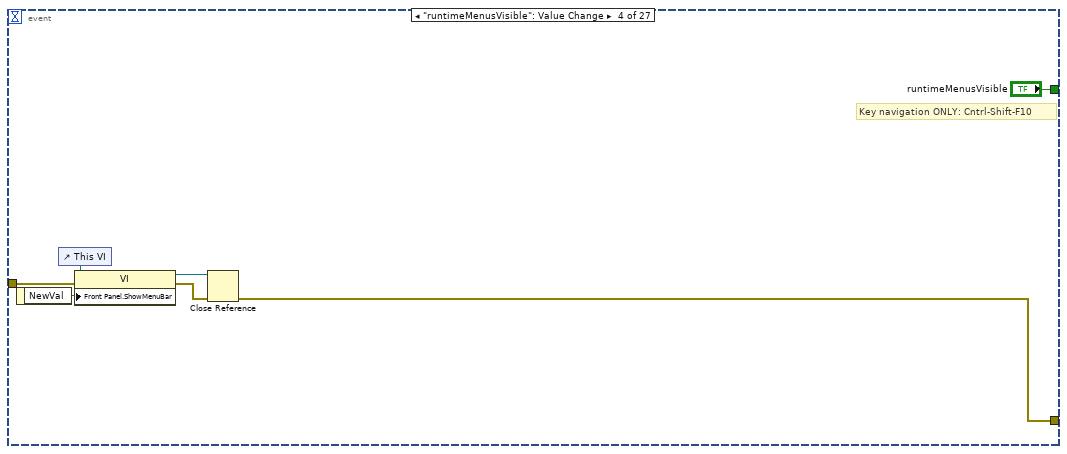
[diagram p7: hidden frame]
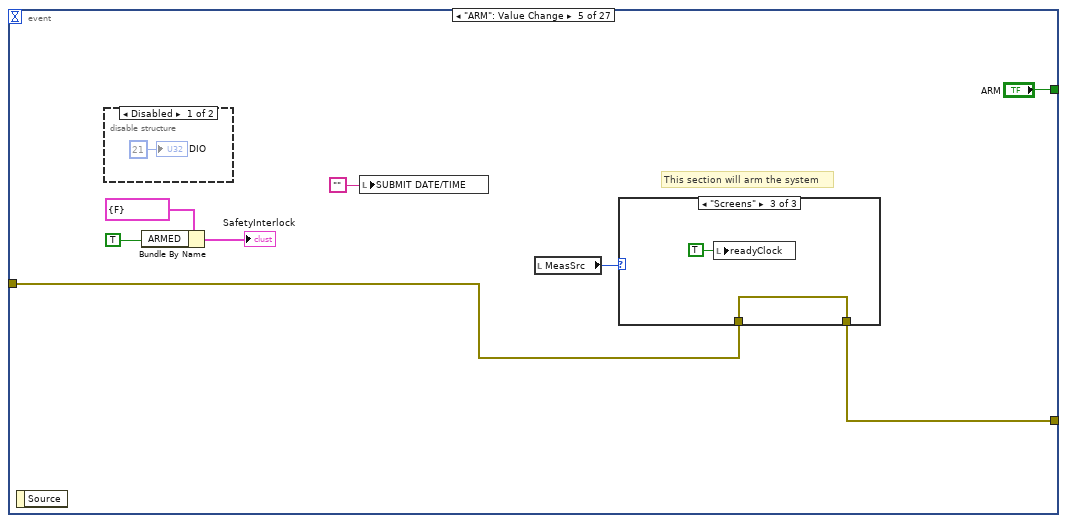
[diagram p8: hidden frame]
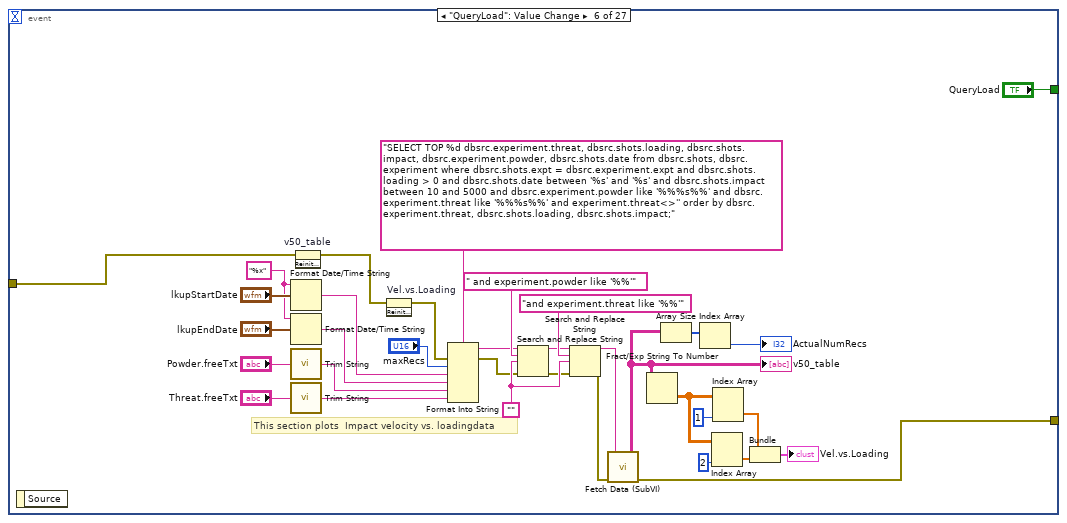
[diagram p12: hidden frame]
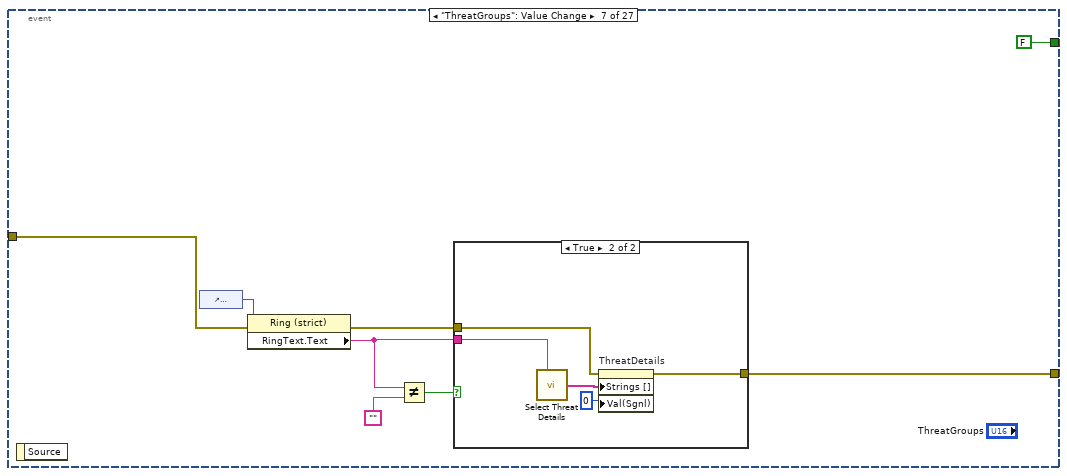
[diagram p13: hidden frame]
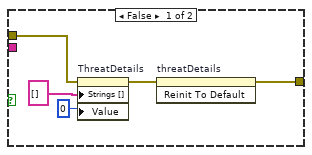
[diagram p14: hidden frame]
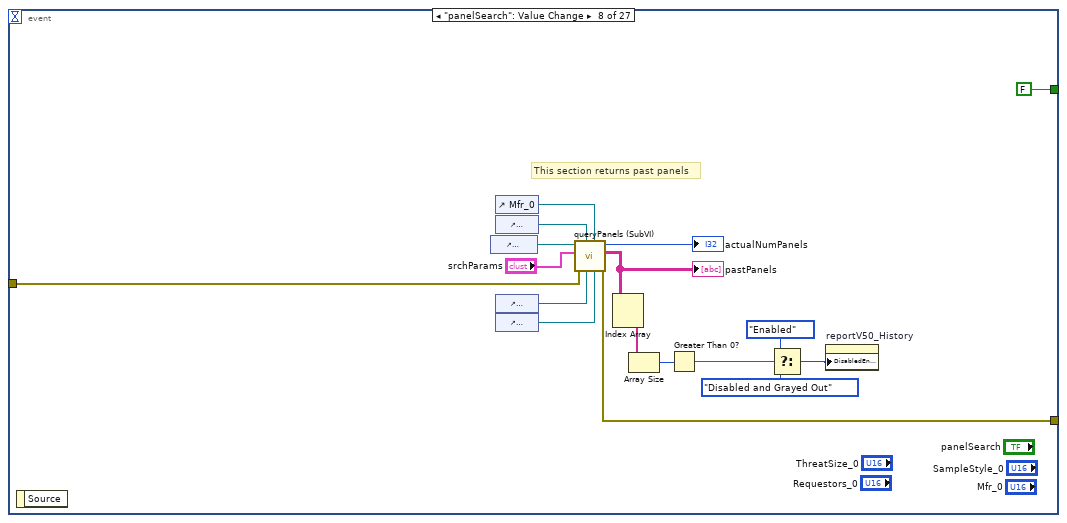
[diagram p15: hidden frame]
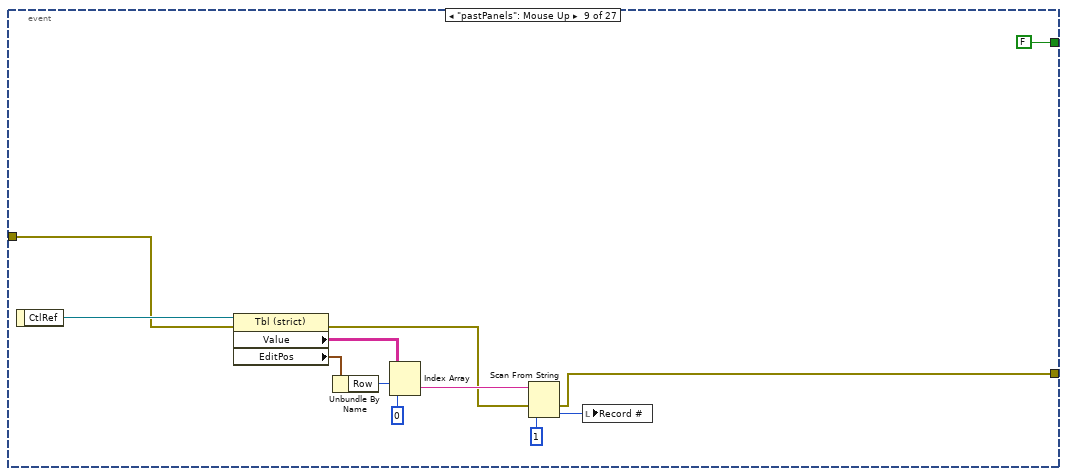
[diagram p16: hidden frame]
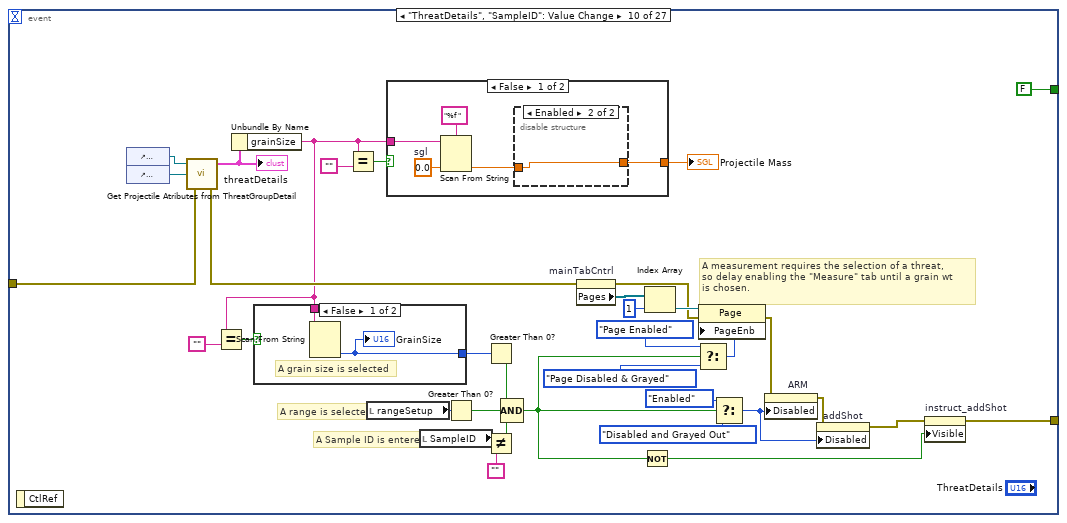
[diagram p17: hidden frame]
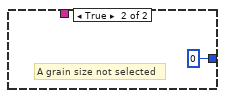
[diagram p18: hidden frame]
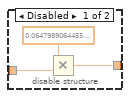
[diagram p19: hidden frame]
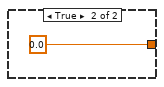
[diagram p20: hidden frame]
diagram:
  w7 = errorcluster {"status"=FALSE, "code"=0, "source"=""}  # error in
  w8 = T7[] []  # Initial Shots
  n1 = property on="RESET All" class="Bool (strict)"("Value"=TRUE ("RESET")) -> (error out=w10:errorcluster)  [unwired: 2 in, 1 out]
  n2 = while "Test Executive State Machine" {
    shift-left: 100 -> [w18]
    shift-right: [w19] -> _
    shift-left: Collector_State."INITIALIZE" ("progState") -> [w15]
    shift-right: [w20] -> _
    shift-right: [w16] -> _
    shift-left: w8 -> [w17]
    shift-right: [w13] -> _
    shift-left: w10 -> [w14]
    tunnel: "LayerTabControl" -> [_]
    tunnel: "aboutTabCntrl" -> [_]
    tunnel: "historyTabCntrl" -> [_]
    tunnel: "SampleEntryTabCntrl" -> [_]
    tunnel: "Sample SubTabCntrl" -> [_]
    tunnel: "shotsTabCntrl" -> [_]
    stop <- FALSE stop-if-true
    n3 = case shown="9" w15 {
      tunnel: [w24 w144 Collector_State."POLL" ("progState") Collector_State."POLL" ("progState") w1181 Collector_State."PROCESS SHOTS" ("progState") Collector_State."POLL" ("progState") Collector_State."PROCESS SHOTS" ("progState") Collector_State."PROCESS SHOTS" ("progState") Collector_State."POLL" ("progState") Collector_State."POLL" ("progState") w1849] -> w20
      tunnel: [-1 -1 ("index of element") -1 ("index of element") -1 ("index of element") w1180 -1 ("index of element") -1 -1 ("index of element") -1 ("index of element") -1 -1 ("index of element") w1848] -> w19
      tunnel: w18 -> [_ w145 _ _ _ _ _ _ _ _ _ _]
      tunnel: w17 -> [w28 w143 w300 w928 w1174 w1437 w1482 w1505 w1511 w1564 w1616 w1852]
      tunnel: [w27 w142 w300 w928 w1173 w1424 w1486 w1504 w1510 w1564 w1620 w1852] -> w16
      tunnel: w14 -> [_ w138 w297 w926 w1176 w1432 w1478 w1494 w1506 w1560 w1615 w1843]
      tunnel: [w36 w139 w296 w925 w1175 w1430 w1478 w1492 w1507 w1559 w1614 w1844] -> w13
      frame 0, Default {
        w29 = Collector_State."POLL"  # progStateType
        w49 = TRUE  # element
        w52 = 4  # SAVE
        # "This section checks for any buttons, maintains routine check of the paramters"
        n4 = case shown="\"Setup\", Default" "mainTabCntrl" {
          tunnel: w28 -> [_ w108 _ _]
          frame "Setup", Default {
            n5 = control-ref of="layerStitch_1"() -> (w76:refnum<vi>)
            n6 = control-ref of="layerStitch_2"() -> (w73:refnum<vi>)
            n7 = control-ref of="layerStitch_3"() -> (w72:refnum<vi>)
            n8 = control-ref of="layerStitch_4"() -> (w71:refnum<vi>)
            n9 = control-ref of="layerStitch_5"() -> (w70:refnum<vi>)
            n10 = control-ref of="layerStitch_6"() -> (w69:refnum<vi>)
            n11 = control-ref of="SampleStyle_0"() -> (w74:refnum<vi>)
            n12 = control-ref of="SampleStyle_1"() -> (w90:refnum<vi>)
            n13 = control-ref of="SampleStyle_2"() -> (w91:refnum<vi>)
            n14 = control-ref of="SampleStyle_3"() -> (w92:refnum<vi>)
            n15 = control-ref of="SampleStyle_4"() -> (w93:refnum<vi>)
            n16 = control-ref of="SampleStyle_5"() -> (w94:refnum<vi>)
            n17 = control-ref of="SampleStyle_6"() -> (w95:refnum<vi>)
            n18 = Build Array(w74, w90, w91, w92, w93, w94, w95) -> (w88:refnum<vi>[])
            n19 = global write "BIMS_Collector Globals.vi" "SampleStyles"(w88) -> ()
            n20 = Build Array(w76, w73, w72, w71, w70, w69) -> (w77:refnum<vi>[])
            n21 = global write "BIMS_Collector Globals.vi" "LayerStitchTypeRefs"(w77) -> ()
            n22 = local read "SampleAttribs_1"() -> (w82:T3)
            n23 = local read "SampleAttribs_2"() -> (w84:T3)
            n24 = local read "SampleAttribs_3"() -> (w85:T3)
            n25 = local read "SampleAttribs_4"() -> (w86:T3)
            n26 = local read "SampleAttribs_5"() -> (w87:T3)
            n27 = local read "SampleAttribs_6"() -> (w83:T3)
            n28 = Build Array(w82, w84, w85, w86, w87, w83) -> (w81:T20)
            n29 = global write "BIMS_Collector Globals.vi" "SampleAttribs"(w81) -> ()
            n30 = local read "Fabric Description"() -> (w80:string)
            n31 = control-ref of="Mfr_0"() -> (w75:refnum<vi>)
            n32 = control-ref of="Mfr_1"() -> (w101:refnum<vi>)
            n33 = control-ref of="Mfr_2"() -> (w100:refnum<vi>)
            n34 = control-ref of="Mfr_3"() -> (w99:refnum<vi>)
            n35 = control-ref of="Mfr_4"() -> (w98:refnum<vi>)
            n36 = control-ref of="Mfr_5"() -> (w97:refnum<vi>)
            n37 = control-ref of="Mfr_6"() -> (w96:refnum<vi>)
            n38 = String Subset(string=w80, length (rest)=75 ("length (rest)")) -> (substring=w79:string)  [unwired: 1 out]
            n39 = Build Array(w75, w101, w100, w99, w98, w97, w96) -> (w89:refnum<vi>[])
            n40 = local write "Fabric Description"(w79) -> ()
            n41 = global write "BIMS_Collector Globals.vi" "Mfrs"(w89) -> ()
          }
          frame "Measure" {
            # "Disable and gray out the \"Save\" button\nIF the shot table has no shots, \nOR if there are no plies; otherwise, enable it."
            # "Disable and gray out the \"Clear Shots\" button\nIF the shot table has no shots; otherwise, enable it."
            n42 = Array Size(array=w108) -> (size(s)=w115:i32)
            n43 = Equal To 0?(x=w115) -> (x = 0?=w102:bool)
            n44 = property on="saveReq" class="Str"("Visible"=w102) -> ()  [unwired: 2 in, 2 out]
            n45 = Select(t=T15."Disabled and Grayed Out" ("Disabled"), s=w102, f=T15."Enabled" ("Disabled")) -> (s? t:f=w114:T15)
            n46 = Select(t=T15."Disabled and Grayed Out" ("Disabled"), s=w102, f=T15."Enabled" ("Disabled")) -> (s? t:f=w103:T15)
            n47 = property on="reportV50" class="Bool"("Disabled"=w103) -> ()  [unwired: 2 in, 2 out]
            n48 = property on="saveShots" class="Bool"("Disabled"=w103) -> ()  [unwired: 2 in, 2 out]
            n49 = property on="clearShots" class="Bool"("Disabled"=w114) -> ()  [unwired: 2 in, 2 out]
            n50 = local read "Shot Description"() -> (w111:string)
            n51 = String Subset(string=w111, length (rest)=30 ("length (rest)")) -> (substring=w109:string)  [unwired: 1 out]
            n52 = local write "Shot Description"(w109) -> ()
            "SHOT STATUS" <- "Current/sthotstatus"
            "BACKFACE DEPTH" <- "backdepth"
          }
          frame "History" {
          }
          frame "System" {
          }
        }
        n53 = Get Date/Time String(want seconds? (F)=TRUE) -> (date string=w34:string, time string=w35:string)  [unwired: 2 in]
        n54 = call <vilib>:"Space Constant.vi"() -> ("String"=w32:string)
        n55 = Concatenate Strings(w34, w32, w35) -> (w33:string)
        n56 = local write "currentDateTime"(w33) -> ()
        n57 = Or(x="undoLastShot", y="deleteShot") -> (x .or. y?=w47:bool)
        n58 = Or(x="reportV50", y="reportV50_History") -> (x .or. y?=w55:bool)
        n59 = flat-sequence {
          tunnel: [w68] -> w30
          frame #0 {
            n60 = Wait (ms)(milliseconds to wait=u32 200 ("millisecond timer value")) -> ()  [unwired: 1 out]
          }
          frame #1 {
            n61 = local read "SMErr"() -> (w68:errorcluster)
          }
        }
        n62 = Build Array("RESET All", w55, "VsVr Report", "saveShots", "addShot", "clearShots", "nextShot", w47, "processShots", "readyClock") -> (w50:bool[])
        n63 = Search 1D Array(1D array=w50, element=w49) -> (index of element=w60:i32)  [unwired: 1 out]
        n64 = Increment(x=w60) -> (x+1=w61:i32)
        n65 = Equal?(x=w61, y=w52) -> (x = y?=w53:bool)
        n66 = case shown="False" w53 {
          tunnel: w61 -> [w117 w129]
          tunnel: [w118 w134] -> w59
          tunnel: w30 -> [w116 w125]
          tunnel: [w116 w123] -> w36
          frame False {
            w120 = 0  # Not Found
            n67 = Equal?(x=w117, y=w120) -> (x = y?=w119:bool)
            n68 = case shown="True" w119 {
              tunnel: w117 -> [w121 _]
              tunnel: [w121 w122] -> w118
              frame False {
              }
              frame True {
                w122 = 11  # CheckDAQ
                # "USUAL SCENARIO"
              }
            }
          }
          frame True {
            # "Before allowing data record to be saved,\nprompt user to validate."
            n69 = call "Get Last Record (SubVI).vi"("error in"=w125) -> ("error out"=w124:errorcluster, "experiment record"=w126:i32, "shot record"=w127:i32)  [unwired: 2 out]
            n70 = local write "LastShot"(w127) -> ()
            n71 = local write "LastSample"(w126) -> ()
            n72 = To Double Precision Float(number=w126) -> (double precision float=w128:dbl)
            n73 = Two Button Dialog(message="Are ALL Data Valid?", 1:"NO" ("F button name (\"Cancel\")"), 2:"YES" ("T button name (\"OK\")")) -> (T button?=w133:bool)
            n74 = property on="Record #" class="DigNum (strict)"(error in=w124, "Maximum"=w128) -> (error out=w123:errorcluster)  [unwired: 1 in, 1 out]
            n75 = case shown="False" w133 {
              tunnel: [0 ("index of element") w136] -> w134
              tunnel: w129 -> [_ w136]
              frame False {
                # "POLL"
              }
              frame True {
              }
            }
          }
        }
        n76 = local read "SHOTS"() -> (w27:T7[])
        n77 = To Variant(anything=w59) -> (Variant=w58:variant)
        n78 = for {
          tunnel: w28 -> [w65] mode=indexing
          tunnel: w27 -> [w66] mode=indexing
          tunnel: [w62] -> w26 mode=indexing
          n79 = Not Equal?(x=w66, y=w65) -> (x != y?=w64:T21)
          n80 = Cluster To Array(cluster=w64) -> (array=w63:bool[])
          n81 = Or Array Elements(Boolean array=w63) -> (logical OR=w62:bool)
        }
        n82 = Variant To Data(type=w29, Variant=w58) -> (data=w25:T13)  [unwired: 1 in, 1 out]
        n83 = Or Array Elements(Boolean array=w26) -> (logical OR=w22:bool)
        n84 = Select(t=Collector_State."PROCESS SHOTS" ("progStateType"), s=w22, f=w25) -> (s? t:f=w24:u16)
        "STOP (Shots MC LB)" <- TRUE ("STOP (Shots MC LB)")
      }
      frame 1 {
        # "This section reads the ini file"
        n85 = case shown="100" w145 {
          tunnel: [w151 w170] -> w146
          tunnel: [w149 w170] -> w141
          tunnel: w138 -> [w148 w162]
          tunnel: [w147 w162] -> w137
          frame 0, Default {
            n86 = local read "RESET All"() -> (w150:bool)
            n87 = case shown="True" w150 {
              tunnel: [TRUE w158] -> w151
              tunnel: [FALSE w158] -> w149
              tunnel: w148 -> [w152 w155]
              tunnel: [w152 w155] -> w147
              frame False {
                # "Refresh"
              }
              frame True {
                n88 = Two Button Dialog(message="Resetting will remove all unsaved data.\n\nDo you really  want to reset? ", 1:"NO" ("F button name (\"Cancel\")"), 2:"YES" ("T button name (\"OK\")")) -> (T button?=w158:bool)
              }
            }
          }
          frame 100 {
            w170 = TRUE  # Reset ALL
            n89 = property on="Loading" class="Ring (strict)"("Visible"=FALSE) -> ()  [unwired: 2 in, 2 out]
            n90 = control-ref of="Mfr_0"() -> (w160:refnum<vi>)
            n91 = control-ref of="Mfr_1"() -> (w169:refnum<vi>)
            n92 = control-ref of="Mfr_2"() -> (w168:refnum<vi>)
            n93 = control-ref of="Mfr_3"() -> (w167:refnum<vi>)
            n94 = control-ref of="Mfr_4"() -> (w166:refnum<vi>)
            n95 = control-ref of="Mfr_5"() -> (w165:refnum<vi>)
            n96 = control-ref of="Mfr_6"() -> (w164:refnum<vi>)
            n97 = Build Array(w160, w169, w168, w167, w166, w165, w164) -> (w163:refnum<vi>[])
            n98 = global write "BIMS_Collector Globals.vi" "Mfrs"(w163) -> ()
          }
        }
        n99 = case shown="True" w146 {
          tunnel: [Collector_State."POLL" ("progState") w208] -> w144
          tunnel: w143 -> [w173 _]
          tunnel: [w173 "SHOTS"] -> w142
          tunnel: w141 -> [_ w209]
          tunnel: [w171 w188] -> w139
          tunnel: w137 -> [w171 w207]
          frame False {
            n100 = local write "RESET All"(FALSE ("RESET")) -> ()
          }
          frame True {
            n101 = case shown="True" w209 {
              selector: w209 -> [_ w241]
              tunnel: [w223 w241] -> w189
              tunnel: [w222 w256] -> w190
              tunnel: w207 -> [w222 w243]
              tunnel: [w221 w240] -> w186
              frame False {
                w223 = FALSE  # Reset All
                # "Refresh"
                n102 = local read "configPath"() -> (w221:path)
              }
              frame True {
                # "This section resets\nentire program"
                # "Reset ALL"
                n103 = control-ref of="This VI"() -> (w233:refnum<vi>)
                n104 = invoke on="Invoke Node" class="VI" method="Default Vals.Reinit All"(reference=w233, error in=w243) -> (reference out=w232:refnum<vi>, error out=w231:errorcluster)  [unwired: 1 in, 1 out]
                n105 = property class="VI"(reference=w232, error in=w231, "Front Panel.ShowMenuBar"=FALSE ("Front Panel Window:Show Menu Bar")) -> (reference out=w229:refnum<vi>, error out=w227:errorcluster)
                n106 = property on="mainTabCntrl" class="TabCtl (strict)"() -> (error out=w235:errorcluster, "Pages"=w237:refnum<vi>[])  [unwired: 2 in, 1 out]
                n107 = control-ref of="ScreenSetAvgg"() -> (w251:refnum<vi>)
                n108 = control-ref of="InterlockExists"() -> (w252:refnum<vi>)
                n109 = control-ref of="useBallisitican"() -> (w253:refnum<vi>)
                n110 = control-ref of="useRecorder"() -> (w254:refnum<vi>)
                n111 = control-ref of="useShooter"() -> (w255:refnum<vi>)
                n112 = control-ref of="useBMC"() -> (w226:refnum<vi>)
                n113 = Close Reference(reference=w229, error in (no error)=w227) -> (error out=w228:errorcluster)
                n114 = Index Array(array=w237, index=1) -> (element=w239:refnum<vi>)
                n115 = call "RegReadParams.vi"("ScreenSetAveraging_Ref"=w251, "useBMC_Ref"=w226, "InterlockExist_Ref"=w252, "errorIN"=w228, "useShooter_Ref"=w255, "useRecorder_Ref"=w254, "useBallistician_Ref"=w253) -> ("error out"=w250:errorcluster)  [unwired: 4 out]
                n116 = control-ref of="Server"() -> (w242:refnum<vi>)
                n117 = control-ref of="ConfigName"() -> (w246:refnum<vi>)
                n118 = control-ref of="Site"() -> (w244:refnum<vi>)
                n119 = control-ref of="Folder"() -> (w225:refnum<vi>)
                n120 = property on="Property Node" class="Page"(reference=w239, error in=w235, "PageEnb"=T16."Page Disabled & Grayed" ("Page Enabled State")) -> (error out=w234:errorcluster)  [unwired: 1 out]
                n121 = Build Array(w246, w244, w242, w225) -> (w247:refnum<vi>[])
                n122 = call "InitStringValuesFromRegistry(SubVI).vi"("error in"=w250, "String References"=w247, "subkey"="SOFTWARE\\DuPont\\BIMS-08\\Collector", "root key (HKEY_LOCAL_MACHINE)"=Registry_RtKey."HKEY_LOCAL_MACHINE") -> ("error out"=w249:errorcluster)  [unwired: 3 out]
                n123 = property on="minV50" class="DigNum (strict)"(error in=w234, "Visible"=w241) -> ()  [unwired: 1 in, 2 out]
                n124 = Current VI's Path() -> (path=w224:path)
                n125 = call "Initialize (SubVI).vi"("path"=w224, "error IN"=w249) -> ("pathConfigOUT"=w240:path, "lengthUnits"=→"lengthUnits":string, "massUnits"=→"massUnits":string, "error out"=w256:errorcluster)  [unwired: 1 out]
                "configPath" <- w240
              }
            }
            n126 = control-ref of="Threat"() -> (w193:refnum<vi>)
            n127 = control-ref of="SampleTypes"() -> (w195:refnum<vi>)
            n128 = control-ref of="SampleDescrip"() -> (w202:refnum<vi>)
            n129 = call "Get Threats (SubVI).vi"("pathConfigIN"=w186, "refThreat"=w193, "error in"=w190) -> ("pathConfigOUT"=w197:path, "factorOut"=→"factor array":sgl[], "error out"=w200:errorcluster)  [unwired: 4 out]
            n130 = Bundle("SampleTypes"=w195, "SampleDescrip"=w202) -> (w201:T22)  [unwired: 1 out]
            n131 = call "Fill Lists from INI (SubVI).vi"("clusterListboxes"=w201, "error in"=w200, "pathConfigIN"=w197) -> ("error out"=w199:errorcluster, "pathConfigOUT"=w198:path)  [unwired: 4 out]
            n132 = call "Read Parameters.vi"("error in (no error)"=w199, "appended path"=w198) -> ("error out"=w192:errorcluster, "rangeParams"=w194:T23)  [unwired: 4 out]
            n133 = Unbundle(w194) -> ("max dev"=w175:sgl, "residual separation"=→"Residual/Separation":sgl, "Set#1 Separation"=→"Set#1 Separation":sgl, "Set#2 Separation"=→"Set#2 Separation":sgl, "impact target dist"=w179:sgl, "resid target dist"=w180:sgl, "barrel screen dist"=→"Barrel to Screen":sgl, "midpt_to_target_dist"=→"mid_to_targ_dist":sgl)
            n134 = property on="Ballisticians" class="Ring (strict)"("Visible"="useBallisitican") -> ()  [unwired: 2 in, 2 out]
            n135 = property on="Shooters" class="Ring (strict)"("Visible"="useShooter") -> ()  [unwired: 2 in, 2 out]
            n136 = property on="Recorders" class="Ring (strict)"("Visible"="useRecorder") -> ()  [unwired: 2 in, 2 out]
            n137 = property on="RefreshMetadata" class="Bool (strict)"(error in=w192, "Val(Sgnl)"=TRUE) -> (error out=w187:errorcluster)  [unwired: 1 in, 1 out]
            n138 = local write "Residual/Target Dist"(w180) -> ()
            n139 = local write "maxDev"(w175) -> ()
            n140 = local write "Set#1_to_Target"(w179) -> ()
            n141 = disable-structure shown="Disabled" {
              disable-tunnel: w187 -> [w212 w214]
              disable-tunnel: [w211 w214] -> w183
              frame Disabled {
                n142 = property on="rangeSetup" class="Ring (strict)"(error in=w212, "Val(Sgnl)"=u16 1 ("Value (Signaling)")) -> (error out=w211:errorcluster)  [unwired: 1 in, 1 out]
              }
              frame Enabled {
              }
            }
            n143 = case shown="True" w189 {
              tunnel: [Collector_State."POLL" ("progState") w284] -> w208
              tunnel: [w259 w269] -> w206
              tunnel: w183 -> [w259 w278]
              tunnel: w186 -> [_ w268]
              tunnel: "useBMC" -> [_ w267]
              frame False {
                # "Refresh"
              }
              frame True {
                w261 = T15."Disabled and Grayed Out" ("Disabled")
                # "Reset ALL"
                n144 = global read "BIMS_Collector Globals.vi" "SampleStyles"() -> (w271:refnum<vi>[])
                n145 = case shown="True" w267 {
                  tunnel: w268 -> [_ w286]
                  frame False {
                  }
                  frame True {
                    n146 = Path To String(path=w286) -> (string=w287:string)
                    n147 = call "Ballistics Message Center.vi"("INI File Name"=w287) -> ()
                  }
                }
                n148 = call "Get Last Record (SubVI).vi"("error in"=w278) -> ("error out"=w270:errorcluster, "experiment record"=w276:i32, "shot record"=→"LastShot":i32)  [unwired: 2 out]
                "LastSample" <- w276
                n149 = local read "MeasSrc"() -> (w285:T6)
                n150 = local read "InterlockExists"() -> (w283:bool)
                n151 = control-ref of="ThreatDetails"() -> (w266:refnum<vi>)
                n152 = control-ref of="SampleStyle_0"() -> (w273:refnum<vi>)
                n153 = control-ref of="ThreatGroups"() -> (w272:refnum<vi>)
                n154 = local read "SafetyInterlock"() -> (w281:cluster{"ARMED":bool})
                n155 = Bundle By Name(cluster=w281, "ARMED"=FALSE) -> (w280:cluster{"ARMED":bool})
                n156 = To Double Precision Float(number=w276) -> (double precision float=w275:dbl)
                n157 = property on="Record #" class="DigNum (strict)"(error in=w270, "Maximum"=w275) -> (error out=w269:errorcluster)  [unwired: 1 in, 1 out]
                n158 = case shown="\"Screens\"" w285 {
                  tunnel: [Collector_State."POLL" ("progState") Collector_State."POLL" ("progState") Collector_State."READY CLOCK" ("progState")] -> w284
                  frame "Simulated", Default {
                  }
                  frame "Radar" {
                  }
                  frame "Screens" {
                    # "check for PCI 6602"
                  }
                }
                n159 = Build Array (concatenate)(w266, w273, w272, w271) -> (w274:refnum<vi>[])
                n160 = local write "SafetyInterlock"(w280) -> ()
                n161 = Select(t=T15."Enabled" ("Disabled"), s=w283, f=T15."Disabled and Grayed Out" ("Disabled")) -> (s? t:f=w282:T15)
                n162 = for {
                  tunnel: w274 -> [w288] mode=indexing
                  n163 = property on="Property Node" class="Ring (strict)"(reference=w288, "Strings []"=string[] []) -> ()  [unwired: 1 in, 2 out]
                }
                n164 = property on="addShot" class="Bool"("Disabled"=T15."Enabled") -> ()  [unwired: 2 in, 2 out]
                n165 = property on="undoLastShot" class="Bool"("Disabled"=w261) -> ()  [unwired: 2 in, 2 out]
                n166 = property on="saveShots" class="Bool"("Disabled"=w261) -> ()  [unwired: 2 in, 2 out]
                n167 = property on="clearShots" class="Bool"("Disabled"=w261) -> ()  [unwired: 2 in, 2 out]
                n168 = property on="ARM" class="Bool"("Disabled"=w282) -> ()  [unwired: 2 in, 2 out]
                n169 = property on="SafetyInterlock" class="Clust (strict)"("Disabled"=w282) -> ()  [unwired: 2 in, 2 out]
                n170 = property on="saveReq" class="Str"("Visible"=TRUE) -> ()  [unwired: 2 in, 2 out]
              }
            }
            n171 = call <vilib>:"General Error Handler.vi"("error in (no error)"=w206) -> ("error out"=w188:errorcluster)  [unwired: 2 in, 12 out]
            n172 = flat-sequence {
              tunnel: w188 -> [w215]
              frame #0 {
                n173 = local read "ConfigName"() -> (w216:string)
                n174 = case shown="No Error" w215 {
                  tunnel: [w219 "NOT READY!" ("ConfigName")] -> w217
                  tunnel: w216 -> [w219 _]
                  frame No Error {
                    n175 = Wait (ms)(milliseconds to wait=u32 1000) -> ()  [unwired: 1 out]
                  }
                  frame Error {
                  }
                }
                "ConfigName" <- w217
              }
            }
            "saveReq" <- "Number of layers in sample ply specification and number of shots in shots table must be greater than 0 to enable saving." ("saveReq")
          }
        }
      }
      frame 2 {
        # "The custom Excel template file is \nexpected in the C:\\Ballistics folder."
        n176 = case shown="False" "lookupRec" {
          selector: "lookupRec" -> [_ w907]
          tunnel: [w343 w897] -> w324
          tunnel: [w342 w883] -> w323
          tunnel: [w341 w900] -> w322
          tunnel: [w340 w840] -> w321
          tunnel: [w339 w898] -> w320
          tunnel: [w338 w860] -> w319
          tunnel: [w337 w847] -> w306
          tunnel: [w336 w849] -> w305
          tunnel: [w335 w850] -> w304
          tunnel: [w334 "Record #"] -> w303
          tunnel: [w333 w899] -> w302
          tunnel: [w332 w849] -> w295
          tunnel: w300 -> [w331 _]
          tunnel: [w330 w872] -> w298
          tunnel: w297 -> [w330 w873]
          tunnel: [w329 w845] -> w293
          frame False {
            n177 = stacked-sequence {
              tunnel: [_ _ _ _ _ w740] -> w338
              tunnel: [_ w412 _ _ _ _] -> w342
              tunnel: [_ _ _ _ w532 _] -> w339
              tunnel: [_ _ _ w465 _ _] -> w340
              tunnel: [_ _ w434 _ _ _] -> w341
              tunnel: [w355 _ _ _ _ _] -> w343
              tunnel: [_ _ _ _ _ w746] -> w337
              tunnel: [_ _ _ _ _ w742] -> w336
              tunnel: [_ _ _ _ _ w741] -> w335
              tunnel: [_ _ _ _ _ w745] -> w334
              tunnel: [_ _ _ _ _ w744] -> w333
              tunnel: [_ _ _ _ _ w743] -> w332
              tunnel: w331 -> [_ _ w433 _ w531 _]
              frame #0 {
                # "Need to remove first element\nsince it's associated with the \nhistory page."
                # "FABRIC"
                n178 = local read "fab1_totalWt"() -> (w358:sgl)
                n179 = local read "fab3_totalWt"() -> (w360:sgl)
                n180 = local read "fab5_totalWt"() -> (w362:sgl)
                n181 = global read "BIMS_Collector Globals.vi" "SampleStyles"() -> (w346:refnum<vi>[])
                n182 = global read "BIMS_Collector Globals.vi" "Mfrs"() -> (w351:refnum<vi>[])
                n183 = local read "fab2_totalWt"() -> (w359:sgl)
                n184 = local read "fab4_totalWt"() -> (w361:sgl)
                n185 = local read "fab6_totalWt"() -> (w363:sgl)
                n186 = global read "BIMS_Collector Globals.vi" "LayerStitchTypeRefs"() -> (w353:refnum<vi>[])
                n187 = global read "BIMS_Collector Globals.vi" "SampleAttribs"() -> (w344:T24)
                n188 = global read "BIMS_Collector Globals.vi" "LayerSpecs"() -> (w354:T25)
                n189 = Delete From Array(array=w346, length=1, index=0) -> (array with subset deleted=w345:refnum<vi>[])  [unwired: 1 out]
                n190 = Delete From Array(array=w351, length=1, index=0) -> (array with subset deleted=w352:refnum<vi>[])  [unwired: 1 out]
                n191 = Build Array(w358, w359, w360, w361, w362, w363) -> (w357:sgl[])
                n192 = for {
                  tunnel: w357 -> [w367] mode=indexing
                  tunnel: [w375] -> w356 mode=indexing
                  tunnel: w344 -> [w374] mode=indexing
                  tunnel: w354 -> [w373] mode=indexing
                  tunnel: w352 -> [w372] mode=indexing
                  tunnel: w345 -> [w371] mode=indexing
                  tunnel: w353 -> [w370] mode=indexing
                  n193 = call "Dropdown Selection (SubVI).vi"("reference"=w372) -> ("element"=w365:string)
                  n194 = call "Dropdown Selection (SubVI).vi"("reference"=w371) -> ("element"=w369:string)
                  n195 = Equal?(x="", y=w365) -> (x = y?=w364:bool)
                  n196 = call "Dropdown Selection (SubVI).vi"("reference"=w370) -> ("element"=w368:string)
                  n197 = case shown="False" w364 {
                    tunnel: [w394 w396] -> w375
                    tunnel: w374 -> [w393 _]
                    tunnel: w373 -> [w392 _]
                    tunnel: w369 -> [w386 _]
                    tunnel: w368 -> [w381 _]
                    tunnel: w367 -> [w379 _]
                    tunnel: w365 -> [w378 _]
                    frame False {
                      n198 = Unbundle By Name(w392) -> ("numOfPlies"=w380:i32, "LotNum"=w389:string, "RollNum"=w390:string)
                      n199 = Unbundle By Name(w393) -> ("internal_ID"=w384:string, "fiber"=w385:string, "denier"=w388:string, "pick"=w387:string, "weave"=w382:string, "finish"=w383:string, "ozPerYd2"=w391:string)
                      n200 = Format Into String(w380) -> (resulting string=w377:string)  [unwired: 3 in, 1 out]
                      n201 = Format Into String(w379) -> (resulting string=w376:string)  [unwired: 3 in, 1 out]
                      n202 = Build Array(w377, w378, w386, w384, w385, w388, w387, w382, w383, w389, w390, w391, w376, w381) -> (w394:string[])
                    }
                    frame True {
                      n203 = Initialize Array("", 14 ("dimension size")) -> (w396:string[])
                    }
                  }
                }
                n204 = Transpose 2D Array(2D array=w356) -> (transposed array=w355:string[][])
              }
              frame #1 {
                w398 = "%.1f" ("format string")
                # "muzzel / midpoint"
                # "muzzle / scr#1"
                # "muzzle / target"
                # "scr#2 / target"
                # "RANGE"
                n205 = local read "Set#1 Separation"() -> (w405:sgl)
                n206 = local read "mid_to_targ_dist"() -> (w402:sgl)
                n207 = local read "Barrel to Screen"() -> (w399:sgl)
                n208 = local read "clayAverage"() -> (w420:sgl)
                n209 = Divide(x=w405, y=sgl 2.0) -> (x/y=w400:sgl)
                n210 = local read "RoomHum"() -> (w415:sgl)
                n211 = local read "clayTemp"() -> (w418:sgl)
                n212 = local read "clayCalib"() -> (w421:string)
                n213 = local read "RoomT"() -> (w416:sgl)
                n214 = Add(x=w399, y=w402) -> (x+y=w406:sgl)
                n215 = Subtract(x=w399, y=w400) -> (x-y=w401:sgl)
                n216 = Subtract(x=w402, y=w400) -> (x-y=w403:sgl)
                n217 = Format Into String(w406) -> (resulting string=w407:string)  [unwired: 3 in, 1 out]
                n218 = Format Into String(w401) -> (resulting string=w408:string)  [unwired: 3 in, 1 out]
                n219 = Format Into String(w405) -> (resulting string=w409:string)  [unwired: 3 in, 1 out]
                n220 = Format Into String(w403) -> (resulting string=w410:string)  [unwired: 3 in, 1 out]
                n221 = Format Into String(w402) -> (resulting string=w411:string)  [unwired: 3 in, 1 out]
                n222 = Format Into String(w415) -> (resulting string=w413:string)  [unwired: 3 in, 1 out]
                n223 = Format Into String(format string=w398, w416) -> (resulting string=w414:string)  [unwired: 2 in, 1 out]
                n224 = Format Into String(format string=w398, w418) -> (resulting string=w417:string)  [unwired: 2 in, 1 out]
                n225 = Format Into String(format string=w398, w420) -> (resulting string=w419:string)  [unwired: 2 in, 1 out]
                n226 = Bundle(w407, w408, w409, w410, w411, w413, w414, w417, "clayCalib"=w421, w419) -> (w422:T26)  [unwired: 1 out]
                n227 = Cluster To Array(cluster=w422) -> (array=w412:string[])
              }
              frame #2 {
                # "RESULTS"
                n228 = control-ref of="Methods"() -> (w423:refnum<vi>)
                n229 = call "Dropdown Selection (SubVI).vi"("reference"=w423) -> ("element"=w424:string)
                n230 = for {
                  tunnel: w433 -> [w463] mode=indexing
                  tunnel: [w462] -> w432 mode=indexing
                  tunnel: [w461] -> w431
                  i -> [w461]
                  n231 = Unbundle By Name(w463) -> ("BackFace\nDepth"=w462:sgl)
                }
                n232 = Increment(x=w431) -> (x+1=w429:i32)
                n233 = Add Array Elements(numeric array=w432) -> (sum=w430:sgl)
                n234 = To Single Precision Float(number=w429) -> (single precision float=w428:sgl)
                n235 = Divide(x=w430, y=w428) -> (x/y=w427:sgl)
                n236 = Format Into String(format string="%1.1f", w427) -> (resulting string=w426:string)  [unwired: 2 in, 1 out]
                n237 = case shown="\"V50\"" w424 {
                  tunnel: [w451 w460] -> w436
                  tunnel: w426 -> [w440 w459]
                  frame "V50" {
                    w445 = "%1d" ("format string")
                    w438 = "%1.1f" ("format string")
                    # "June 2012\n- Lucas Louriero requested \nstdev of velocities used in V50"
                    n238 = local read "Z.M.R."() -> (w443:sgl)
                    n239 = Less Than 0?(x=w443) -> (x < 0?=w444:bool)
                    n240 = local read "computed_V50"() -> (w450:sgl)
                    n241 = local read "rangeOfResults"() -> (w447:i32)
                    n242 = local read "lowComplete"() -> (w448:i32)
                    n243 = local read "highPartial"() -> (w449:i32)
                    n244 = local read "velSTDEV"() -> (w437:sgl)
                    n245 = case shown="True" w444 {
                      tunnel: w443 -> [w456 _]
                      tunnel: [w456 sgl 0.0 ("Z.M.R.")] -> w442
                      frame False {
                      }
                      frame True {
                      }
                    }
                    n246 = Format Into String(format string=w438, w437) -> (resulting string=w439:string)  [unwired: 2 in, 1 out]
                    n247 = Format Into String(format string="%1.1f", w450) -> (resulting string=w454:string)  [unwired: 2 in, 1 out]
                    n248 = Format Into String(format string=w445, w449) -> (resulting string=w453:string)  [unwired: 2 in, 1 out]
                    n249 = Format Into String(format string=w445, w448) -> (resulting string=w452:string)  [unwired: 2 in, 1 out]
                    n250 = Format Into String(format string=w445, w447) -> (resulting string=w455:string)  [unwired: 2 in, 1 out]
                    n251 = Format Into String(format string=w438, w442) -> (resulting string=w441:string)  [unwired: 2 in, 1 out]
                    n252 = Bundle(w454, w453, w452, w455, w441, w439, w440) -> (w451:T27)  [unwired: 1 out]
                  }
                  frame Default {
                    w458 = "" ("Empty String Constant")
                    n253 = Bundle(w458, w458, w458, w458, w458, w459, w459) -> (w460:T27)  [unwired: 1 out]
                  }
                }
                n254 = Cluster To Array(cluster=w436) -> (array=w435:string[])
                n255 = Build Array(w435) -> (w434:string[][])
              }
              frame #3 {
                # "SAMPLE"
                n256 = local read "Site"() -> (w464:string)
                n257 = case shown="\"BRZ\"" w464 {
                  tunnel: [w467 w491 w504 w517] -> w465
                  frame "ICE1", Default {
                    # "PB Req"
                    n258 = control-ref of="Methods"() -> (w468:refnum<vi>)
                    n259 = call "Dropdown Selection (SubVI).vi"("reference"=w468) -> ("element"=w470:string)
                    n260 = Equal?(x=w470, y="V50") -> (x = y?=w469:bool)
                    n261 = local read "totalSampleWt"() -> (w480:sgl)
                    n262 = case shown="True" w469 {
                      tunnel: ["n/a" w490] -> w474
                      frame False {
                      }
                      frame True {
                        n263 = local read "minV50"() -> (w489:i32)
                        n264 = Format Into String(w489) -> (resulting string=w490:string)  [unwired: 3 in, 1 out]
                      }
                    }
                    n265 = control-ref of="SampleDimensions"() -> (w486:refnum<vi>)
                    n266 = control-ref of="SampleCoverings"() -> (w487:refnum<vi>)
                    n267 = control-ref of="Models"() -> (w473:refnum<vi>)
                    n268 = local read "serialNum"() -> (w482:string)
                    n269 = local read "SampleID"() -> (w484:string)
                    n270 = local read "Thickness"() -> (w477:dbl)
                    n271 = local read "totalBAW"() -> (w476:sgl)
                    n272 = call "Dropdown Selection (SubVI).vi"("reference"=w486) -> ("element"=w483:string)
                    n273 = call "Dropdown Selection (SubVI).vi"("reference"=w473) -> ("element"=w472:string)
                    n274 = call "Dropdown Selection (SubVI).vi"("reference"=w487) -> ("element"=w481:string)
                    n275 = Format Into String(w480) -> (resulting string=w479:string)  [unwired: 3 in, 1 out]
                    n276 = Format Into String(w477) -> (resulting string=w478:string)  [unwired: 3 in, 1 out]
                    n277 = Format Into String(w476) -> (resulting string=w475:string)  [unwired: 3 in, 1 out]
                    n278 = Bundle("SampleID"=w484, "element"=w483, "Type of work"="Type of work", "serialNum"=w482, "element"=w472, w479, w478, w475, "element"=w481, w474) -> (w485:T28)  [unwired: 1 out]
                    n279 = Cluster To Array(cluster=w485) -> (array=w467:string[])
                  }
                  frame "SPR0" {
                    n280 = local read "totalSampleWt"() -> (w497:sgl)
                    n281 = control-ref of="SampleDimensions"() -> (w502:refnum<vi>)
                    n282 = control-ref of="SampleCoverings"() -> (w503:refnum<vi>)
                    n283 = local read "SampleID"() -> (w500:string)
                    n284 = local read "Thickness"() -> (w494:dbl)
                    n285 = local read "totalBAW"() -> (w493:sgl)
                    n286 = call "Dropdown Selection (SubVI).vi"("reference"=w502) -> ("element"=w499:string)
                    n287 = call "Dropdown Selection (SubVI).vi"("reference"=w503) -> ("element"=w498:string)
                    n288 = Format Into String(w497) -> (resulting string=w496:string)  [unwired: 3 in, 1 out]
                    n289 = Format Into String(w494) -> (resulting string=w495:string)  [unwired: 3 in, 1 out]
                    n290 = Format Into String(w493) -> (resulting string=w492:string)  [unwired: 3 in, 1 out]
                    n291 = Bundle("SampleID"=w500, "element"=w499, w496, w495, w492, "element"=w498) -> (w501:T29)  [unwired: 1 out]
                    n292 = Cluster To Array(cluster=w501) -> (array=w491:string[])
                  }
                  frame "SPR1" {
                    n293 = local read "totalSampleWt"() -> (w510:sgl)
                    n294 = control-ref of="SampleDimensions"() -> (w515:refnum<vi>)
                    n295 = control-ref of="SampleCoverings"() -> (w516:refnum<vi>)
                    n296 = local read "SampleID"() -> (w513:string)
                    n297 = local read "Thickness"() -> (w507:dbl)
                    n298 = local read "totalBAW"() -> (w506:sgl)
                    n299 = call "Dropdown Selection (SubVI).vi"("reference"=w515) -> ("element"=w512:string)
                    n300 = call "Dropdown Selection (SubVI).vi"("reference"=w516) -> ("element"=w511:string)
                    n301 = Format Into String(w510) -> (resulting string=w509:string)  [unwired: 3 in, 1 out]
                    n302 = Format Into String(w507) -> (resulting string=w508:string)  [unwired: 3 in, 1 out]
                    n303 = Format Into String(w506) -> (resulting string=w505:string)  [unwired: 3 in, 1 out]
                    n304 = Bundle("SampleID"=w513, "element"=w512, w509, w508, w505, "element"=w511) -> (w514:T29)  [unwired: 1 out]
                    n305 = Cluster To Array(cluster=w514) -> (array=w504:string[])
                  }
                  frame "BRZ" {
                    n306 = local read "totalSampleWt"() -> (w523:sgl)
                    n307 = control-ref of="SampleDimensions"() -> (w528:refnum<vi>)
                    n308 = control-ref of="SampleCoverings"() -> (w529:refnum<vi>)
                    n309 = local read "SampleID"() -> (w526:string)
                    n310 = local read "Thickness"() -> (w520:dbl)
                    n311 = local read "totalBAW"() -> (w519:sgl)
                    n312 = call "Dropdown Selection (SubVI).vi"("reference"=w528) -> ("element"=w525:string)
                    n313 = call "Dropdown Selection (SubVI).vi"("reference"=w529) -> ("element"=w524:string)
                    n314 = Format Into String(w523) -> (resulting string=w522:string)  [unwired: 3 in, 1 out]
                    n315 = Format Into String(w520) -> (resulting string=w521:string)  [unwired: 3 in, 1 out]
                    n316 = Format Into String(w519) -> (resulting string=w518:string)  [unwired: 3 in, 1 out]
                    n317 = Bundle("SampleID"=w526, "element"=w525, w522, w521, w518, "element"=w524) -> (w527:T29)  [unwired: 1 out]
                    n318 = Cluster To Array(cluster=w527) -> (array=w517:string[])
                  }
                }
              }
              frame #4 {
                n319 = local read "Site"() -> (w530:string)
                n320 = case shown="\"BRZ\"" w530 {
                  tunnel: [w542 w592 w644 w696] -> w532
                  tunnel: w531 -> [w535 w585 w637 w689]
                  frame "ICE1", Default {
                    # "SHOT TABLE"
                    n321 = control-ref of="Methods"() -> (w534:refnum<vi>)
                    n322 = call "Dropdown Selection (SubVI).vi"("reference"=w534) -> ("element"=w533:string)
                    n323 = for {
                      tunnel: w535 -> [w574] mode=indexing
                      shift-right: [w551] -> _
                      shift-left: T18 [] -> [w553]
                      tunnel: [w551] -> w538
                      tunnel: w533 -> [w547]
                      n324 = Unbundle By Name(w574) -> ("shot order"=w573:i32, "Powder Loading"=w572:sgl, "Uncorrected Impact"=w571:sgl, "UncorrectedRed_PB"=w570:sgl, "UncorrectedAvgVel_PB"=w569:sgl, "velLoss_PB"=w568:sgl, "strikeVel_PB"=w567:sgl, "SHOT STATUS"=w556:u16, "usedv50"=w566:bool, "Shot Angle"=w548:u16, "BackFace\nDepth"=w549:sgl)
                      n325 = case shown="\"V50\"" w547 {
                        tunnel: w566 -> [w576 _]
                        tunnel: [w575 w580] -> w565
                        tunnel: w548 -> [_ w579]
                        frame "V50" {
                          n326 = case shown="True" w576 {
                            tunnel: ["" ("Empty String Constant") "*"] -> w575
                            frame False {
                            }
                            frame True {
                            }
                          }
                        }
                        frame Default {
                          n327 = Format Into String(w579) -> (resulting string=w580:string)  [unwired: 3 in, 1 out]
                        }
                      }
                      n328 = case shown="1" w556 {
                        tunnel: ["P" "C"] -> w555
                        frame 0, Default {
                        }
                        frame 1 {
                        }
                      }
                      n329 = Format Into String(format string="%2d", w573) -> (resulting string=w558:string)  [unwired: 2 in, 1 out]
                      n330 = Format Into String(w572) -> (resulting string=w559:string)  [unwired: 3 in, 1 out]
                      n331 = Format Into String(w571) -> (resulting string=w560:string)  [unwired: 3 in, 1 out]
                      n332 = Format Into String(w570) -> (resulting string=w561:string)  [unwired: 3 in, 1 out]
                      n333 = Format Into String(w569) -> (resulting string=w562:string)  [unwired: 3 in, 1 out]
                      n334 = Format Into String(w568) -> (resulting string=w563:string)  [unwired: 3 in, 1 out]
                      n335 = Format Into String(w567) -> (resulting string=w564:string)  [unwired: 3 in, 1 out]
                      n336 = Format Into String(w549) -> (resulting string=w557:string)  [unwired: 3 in, 1 out]
                      n337 = Build Array(w558, w559, w560, w561, w562, w563, w564, w555, w565, w557) -> (w552:string[])
                      n338 = Array To Cluster(array=w552) -> (cluster=w554:T30)
                      n339 = Build Array (concatenate)(w553, w554) -> (w551:T18)
                    }
                    n340 = Array Size(array=w538) -> (size(s)=w540:i32)
                    n341 = Equal To 0?(x=w540) -> (x = 0?=w536:bool)
                    n342 = case shown="True" w536 {
                      tunnel: [w543 T18 [{"[0]"="", "[1]"="", "[2]"="", "[3]"="", "[4]"="", "[5]"="", "[6]"="", "[7]"="", "[8]"="", "[9]"=""}]] -> w537
                      tunnel: w538 -> [w543 _]
                      frame False {
                      }
                      frame True {
                      }
                    }
                    n343 = Sort 1D Array(array=w537) -> (sorted array=w539:T18)
                    n344 = for {
                      tunnel: w539 -> [w546] mode=indexing
                      tunnel: [w545] -> w542 mode=indexing
                      n345 = Cluster To Array(cluster=w546) -> (array=w545:string[])
                    }
                  }
                  frame "SPR0" {
                    # "SHOT TABLE"
                    n346 = control-ref of="Methods"() -> (w584:refnum<vi>)
                    n347 = call "Dropdown Selection (SubVI).vi"("reference"=w584) -> ("element"=w583:string)
                    n348 = for {
                      tunnel: w585 -> [w622] mode=indexing
                      shift-right: [w603] -> _
                      shift-left: T19 [] -> [w605]
                      tunnel: [w603] -> w588
                      tunnel: w583 -> [w599]
                      n349 = Unbundle By Name(w622) -> ("shot order"=w621:i32, "Powder Loading"=w620:sgl, "Uncorrected Impact"=w619:sgl, "UncorrectedRed_PB"=w618:sgl, "strikeVel_PB"=w617:sgl, "SHOT STATUS"=w608:u16, "usedv50"=w616:bool, "Shot Angle"=w600:u16, "BackFace\nDepth"=w601:sgl, "V50userExcl"=w598:bool, "Shot Description"=w597:string)
                      n350 = case shown="\"V50\"" w599 {
                        tunnel: w616 -> [w625 _]
                        tunnel: [w624 w632] -> w615
                        tunnel: w600 -> [_ w631]
                        tunnel: w598 -> [w623 _]
                        frame "V50" {
                          n351 = case shown="True" w623 {
                            tunnel: w625 -> [w627 _]
                            tunnel: [w626 "!"] -> w624
                            frame False {
                              n352 = case shown="False" w627 {
                                tunnel: ["" ("Empty String Constant") "*"] -> w626
                                frame False {
                                }
                                frame True {
                                }
                              }
                            }
                            frame True {
                            }
                          }
                        }
                        frame Default {
                          n353 = Format Into String(w631) -> (resulting string=w632:string)  [unwired: 3 in, 1 out]
                        }
                      }
                      n354 = case shown="1" w608 {
                        tunnel: ["P" "C"] -> w607
                        frame 0, Default {
                        }
                        frame 1 {
                        }
                      }
                      n355 = Format Into String(format string="%2d", w621) -> (resulting string=w610:string)  [unwired: 2 in, 1 out]
                      n356 = Format Into String(w620) -> (resulting string=w611:string)  [unwired: 3 in, 1 out]
                      n357 = Format Into String(w619) -> (resulting string=w612:string)  [unwired: 3 in, 1 out]
                      n358 = Format Into String(w618) -> (resulting string=w613:string)  [unwired: 3 in, 1 out]
                      n359 = Format Into String(w617) -> (resulting string=w614:string)  [unwired: 3 in, 1 out]
                      n360 = Format Into String(w601) -> (resulting string=w609:string)  [unwired: 3 in, 1 out]
                      n361 = Build Array(w610, w611, w612, w613, w614, w607, w615, w609, w597) -> (w604:string[])
                      n362 = Array To Cluster(array=w604) -> (cluster=w606:T31)
                      n363 = Build Array (concatenate)(w605, w606) -> (w603:T19)
                    }
                    n364 = Array Size(array=w588) -> (size(s)=w590:i32)
                    n365 = Equal To 0?(x=w590) -> (x = 0?=w586:bool)
                    n366 = case shown="True" w586 {
                      tunnel: [w593 T19 [{"[0]"="", "[1]"="", "[2]"="", "[3]"="", "[4]"="", "[5]"="", "[6]"="", "[7]"="", "[8]"=""}]] -> w587
                      tunnel: w588 -> [w593 _]
                      frame False {
                      }
                      frame True {
                      }
                    }
                    n367 = Sort 1D Array(array=w587) -> (sorted array=w589:T19)
                    n368 = for {
                      tunnel: w589 -> [w596] mode=indexing
                      tunnel: [w595] -> w592 mode=indexing
                      n369 = Cluster To Array(cluster=w596) -> (array=w595:string[])
                    }
                  }
                  frame "SPR1" {
                    # "SHOT TABLE"
                    n370 = control-ref of="Methods"() -> (w636:refnum<vi>)
                    n371 = call "Dropdown Selection (SubVI).vi"("reference"=w636) -> ("element"=w635:string)
                    n372 = for {
                      tunnel: w637 -> [w674] mode=indexing
                      shift-right: [w655] -> _
                      shift-left: T19 [] -> [w657]
                      tunnel: [w655] -> w640
                      tunnel: w635 -> [w651]
                      n373 = Unbundle By Name(w674) -> ("shot order"=w673:i32, "Powder Loading"=w672:sgl, "Uncorrected Impact"=w671:sgl, "UncorrectedRed_PB"=w670:sgl, "strikeVel_PB"=w669:sgl, "SHOT STATUS"=w660:u16, "usedv50"=w668:bool, "Shot Angle"=w652:u16, "BackFace\nDepth"=w653:sgl, "V50userExcl"=w650:bool, "Shot Description"=w649:string)
                      n374 = case shown="\"V50\"" w651 {
                        tunnel: w668 -> [w677 _]
                        tunnel: [w676 w684] -> w667
                        tunnel: w652 -> [_ w683]
                        tunnel: w650 -> [w675 _]
                        frame "V50" {
                          n375 = case shown="True" w675 {
                            tunnel: w677 -> [w679 _]
                            tunnel: [w678 "!"] -> w676
                            frame False {
                              n376 = case shown="False" w679 {
                                tunnel: ["" ("Empty String Constant") "*"] -> w678
                                frame False {
                                }
                                frame True {
                                }
                              }
                            }
                            frame True {
                            }
                          }
                        }
                        frame Default {
                          n377 = Format Into String(w683) -> (resulting string=w684:string)  [unwired: 3 in, 1 out]
                        }
                      }
                      n378 = case shown="1" w660 {
                        tunnel: ["P" "C"] -> w659
                        frame 0, Default {
                        }
                        frame 1 {
                        }
                      }
                      n379 = Format Into String(format string="%2d", w673) -> (resulting string=w662:string)  [unwired: 2 in, 1 out]
                      n380 = Format Into String(w672) -> (resulting string=w663:string)  [unwired: 3 in, 1 out]
                      n381 = Format Into String(w671) -> (resulting string=w664:string)  [unwired: 3 in, 1 out]
                      n382 = Format Into String(w670) -> (resulting string=w665:string)  [unwired: 3 in, 1 out]
                      n383 = Format Into String(w669) -> (resulting string=w666:string)  [unwired: 3 in, 1 out]
                      n384 = Format Into String(w653) -> (resulting string=w661:string)  [unwired: 3 in, 1 out]
                      n385 = Build Array(w662, w663, w664, w665, w666, w659, w667, w661, w649) -> (w656:string[])
                      n386 = Array To Cluster(array=w656) -> (cluster=w658:T31)
                      n387 = Build Array (concatenate)(w657, w658) -> (w655:T19)
                    }
                    n388 = Array Size(array=w640) -> (size(s)=w642:i32)
                    n389 = Equal To 0?(x=w642) -> (x = 0?=w638:bool)
                    n390 = case shown="True" w638 {
                      tunnel: [w645 T19 [{"[0]"="", "[1]"="", "[2]"="", "[3]"="", "[4]"="", "[5]"="", "[6]"="", "[7]"="", "[8]"=""}]] -> w639
                      tunnel: w640 -> [w645 _]
                      frame False {
                      }
                      frame True {
                      }
                    }
                    n391 = Sort 1D Array(array=w639) -> (sorted array=w641:T19)
                    n392 = for {
                      tunnel: w641 -> [w648] mode=indexing
                      tunnel: [w647] -> w644 mode=indexing
                      n393 = Cluster To Array(cluster=w648) -> (array=w647:string[])
                    }
                  }
                  frame "BRZ" {
                    # "SHOT TABLE"
                    n394 = control-ref of="Methods"() -> (w688:refnum<vi>)
                    n395 = call "Dropdown Selection (SubVI).vi"("reference"=w688) -> ("element"=w687:string)
                    n396 = for {
                      tunnel: w689 -> [w726] mode=indexing
                      shift-right: [w707] -> _
                      shift-left: T19 [] -> [w709]
                      tunnel: [w707] -> w692
                      tunnel: w687 -> [w703]
                      n397 = Unbundle By Name(w726) -> ("shot order"=w725:i32, "Powder Loading"=w724:sgl, "Uncorrected Impact"=w723:sgl, "UncorrectedRed_PB"=w722:sgl, "strikeVel_PB"=w721:sgl, "SHOT STATUS"=w712:u16, "usedv50"=w720:bool, "Shot Angle"=w704:u16, "BackFace\nDepth"=w705:sgl, "V50userExcl"=w702:bool, "Shot Description"=w701:string)
                      n398 = case shown="\"V50\"" w703 {
                        tunnel: w720 -> [w729 _]
                        tunnel: [w728 w736] -> w719
                        tunnel: w704 -> [_ w735]
                        tunnel: w702 -> [w727 _]
                        frame "V50" {
                          n399 = case shown="True" w727 {
                            tunnel: w729 -> [w731 _]
                            tunnel: [w730 "!"] -> w728
                            frame False {
                              n400 = case shown="False" w731 {
                                tunnel: ["" ("Empty String Constant") "*"] -> w730
                                frame False {
                                }
                                frame True {
                                }
                              }
                            }
                            frame True {
                            }
                          }
                        }
                        frame Default {
                          n401 = Format Into String(w735) -> (resulting string=w736:string)  [unwired: 3 in, 1 out]
                        }
                      }
                      n402 = case shown="1" w712 {
                        tunnel: ["P" "C"] -> w711
                        frame 0, Default {
                        }
                        frame 1 {
                        }
                      }
                      n403 = Format Into String(format string="%2d", w725) -> (resulting string=w714:string)  [unwired: 2 in, 1 out]
                      n404 = Format Into String(w724) -> (resulting string=w715:string)  [unwired: 3 in, 1 out]
                      n405 = Format Into String(w723) -> (resulting string=w716:string)  [unwired: 3 in, 1 out]
                      n406 = Format Into String(w722) -> (resulting string=w717:string)  [unwired: 3 in, 1 out]
                      n407 = Format Into String(w721) -> (resulting string=w718:string)  [unwired: 3 in, 1 out]
                      n408 = Format Into String(w705) -> (resulting string=w713:string)  [unwired: 3 in, 1 out]
                      n409 = Build Array(w714, w715, w716, w717, w718, w711, w719, w713, w701) -> (w708:string[])
                      n410 = Array To Cluster(array=w708) -> (cluster=w710:T31)
                      n411 = Build Array (concatenate)(w709, w710) -> (w707:T19)
                    }
                    n412 = Array Size(array=w692) -> (size(s)=w694:i32)
                    n413 = Equal To 0?(x=w694) -> (x = 0?=w690:bool)
                    n414 = case shown="True" w690 {
                      tunnel: [w697 T19 [{"[0]"="", "[1]"="", "[2]"="", "[3]"="", "[4]"="", "[5]"="", "[6]"="", "[7]"="", "[8]"=""}]] -> w691
                      tunnel: w692 -> [w697 _]
                      frame False {
                      }
                      frame True {
                      }
                    }
                    n415 = Sort 1D Array(array=w691) -> (sorted array=w693:T19)
                    n416 = for {
                      tunnel: w693 -> [w700] mode=indexing
                      tunnel: [w699] -> w696 mode=indexing
                      n417 = Cluster To Array(cluster=w700) -> (array=w699:string[])
                    }
                  }
                }
              }
              frame #5 {
                n418 = local read "Site"() -> (w739:string)
                n419 = case shown="\"BRZ\"" w739 {
                  tunnel: [w770 w791 w811 w831] -> w746
                  tunnel: [w769 w790 w810 w830] -> w745
                  tunnel: [w768 w789 w809 w829] -> w744
                  tunnel: [w767 w774 w794 w814] -> w743
                  tunnel: ["" ("projNum") w774 w794 w814] -> w742
                  tunnel: [w765 w788 w808 w828] -> w741
                  tunnel: [w749 w777 w797 w817] -> w740
                  frame "ICE1", Default {
                    # "THREAT"
                    # "Range # (supports a PB reporting requirement)"
                    # "Project Name goes here.\nSupports a PB reporting requirement."
                    # "GENERAL"
                    n420 = local read "threatDetails"() -> (w748:T1)
                    n421 = Unbundle By Name(w748) -> ("barrelLength"=w752:string)
                    n422 = Unbundle By Name(w748) -> ("grainSize"=w747:string)
                    n423 = local read "Shot Angle"() -> (w753:u16)
                    n424 = control-ref of="WeaponTypes"() -> (w762:refnum<vi>)
                    n425 = control-ref of="ThreatGroups"() -> (w761:refnum<vi>)
                    n426 = control-ref of="PowderTypes"() -> (w760:refnum<vi>)
                    n427 = control-ref of="Recorders"() -> (w763:refnum<vi>)
                    n428 = control-ref of="Shooters"() -> (w764:refnum<vi>)
                    n429 = Format Into String(w753) -> (resulting string=w754:string)  [unwired: 3 in, 1 out]
                    n430 = call "Dropdown Selection (SubVI).vi"("reference"=w762) -> ("element"=w758:string)
                    n431 = call "Dropdown Selection (SubVI).vi"("reference"=w761) -> ("element"=w757:string)
                    n432 = call "Dropdown Selection (SubVI).vi"("reference"=w760) -> ("element"=w756:string)
                    n433 = call "Dropdown Selection (SubVI).vi"("reference"=w763) -> ("element"=w755:string)
                    n434 = call "Dropdown Selection (SubVI).vi"("reference"=w764) -> ("element"=w751:string)
                    n435 = Bundle("element"=w758, "element"=w757, "grainSize"=w747, "element"=w756, "barrelLength"=w752, w754, "element"="1", "element"=w751, "element"=w755) -> (w759:T32)  [unwired: 1 out]
                    n436 = local read "LastSample"() -> (w773:i32)
                    n437 = local read "Comments"() -> (w768:string)
                    n438 = local read "ProjectID"() -> (w765:string)
                    n439 = Cluster To Array(cluster=w759) -> (array=w749:string[])
                    n440 = control-ref of="Methods"() -> (w771:refnum<vi>)
                    n441 = control-ref of="TestStandards"() -> (w772:refnum<vi>)
                    n442 = call "Dropdown Selection (SubVI).vi"("reference"=w771) -> ("element"=w770:string)
                    n443 = call "Dropdown Selection (SubVI).vi"("reference"=w772) -> ("element"=w767:string)
                    n444 = Increment(x=w773) -> (x+1=w769:i32)
                  }
                  frame "SPR0" {
                    w774 = "" ("projNum")
                    # "THREAT"
                    # "Project Name goes here.\nSupports a PB reporting requirement."
                    # "GENERAL"
                    n445 = local read "threatDetails"() -> (w776:T1)
                    n446 = Unbundle By Name(w776) -> ("barrelLength"=w779:string)
                    n447 = Unbundle By Name(w776) -> ("grainSize"=w775:string)
                    n448 = local read "Shot Angle"() -> (w780:u16)
                    n449 = control-ref of="ThreatGroups"() -> (w786:refnum<vi>)
                    n450 = control-ref of="PowderTypes"() -> (w785:refnum<vi>)
                    n451 = control-ref of="Ballisticians"() -> (w787:refnum<vi>)
                    n452 = Format Into String(w780) -> (resulting string=w781:string)  [unwired: 3 in, 1 out]
                    n453 = call "Dropdown Selection (SubVI).vi"("reference"=w786) -> ("element"=w783:string)
                    n454 = call "Dropdown Selection (SubVI).vi"("reference"=w785) -> ("element"=w782:string)
                    n455 = call "Dropdown Selection (SubVI).vi"("reference"=w787) -> ("element"=w778:string)
                    n456 = Bundle("element"=w783, "grainSize"=w775, "element"=w782, "barrelLength"=w779, w781, "element"=w778) -> (w784:T33)  [unwired: 1 out]
                    n457 = local read "LastSample"() -> (w793:i32)
                    n458 = local read "Comments"() -> (w789:string)
                    n459 = local read "ProjectID"() -> (w788:string)
                    n460 = control-ref of="Methods"() -> (w792:refnum<vi>)
                    n461 = Cluster To Array(cluster=w784) -> (array=w777:string[])
                    n462 = call "Dropdown Selection (SubVI).vi"("reference"=w792) -> ("element"=w791:string)
                    n463 = Increment(x=w793) -> (x+1=w790:i32)
                  }
                  frame "SPR1" {
                    w794 = "" ("projNum")
                    # "THREAT"
                    # "Project Name goes here.\nSupports a PB reporting requirement."
                    # "GENERAL"
                    n464 = local read "threatDetails"() -> (w796:T1)
                    n465 = Unbundle By Name(w796) -> ("barrelLength"=w799:string)
                    n466 = Unbundle By Name(w796) -> ("grainSize"=w795:string)
                    n467 = local read "Shot Angle"() -> (w800:u16)
                    n468 = control-ref of="Ballisticians"() -> (w807:refnum<vi>)
                    n469 = control-ref of="ThreatGroups"() -> (w806:refnum<vi>)
                    n470 = control-ref of="PowderTypes"() -> (w805:refnum<vi>)
                    n471 = call "Dropdown Selection (SubVI).vi"("reference"=w807) -> ("element"=w798:string)
                    n472 = call "Dropdown Selection (SubVI).vi"("reference"=w806) -> ("element"=w803:string)
                    n473 = call "Dropdown Selection (SubVI).vi"("reference"=w805) -> ("element"=w802:string)
                    n474 = Format Into String(w800) -> (resulting string=w801:string)  [unwired: 3 in, 1 out]
                    n475 = Bundle("element"=w803, "grainSize"=w795, "element"=w802, "barrelLength"=w799, w801, "element"=w798) -> (w804:T33)  [unwired: 1 out]
                    n476 = local read "LastSample"() -> (w813:i32)
                    n477 = local read "Comments"() -> (w809:string)
                    n478 = local read "ProjectID"() -> (w808:string)
                    n479 = control-ref of="Methods"() -> (w812:refnum<vi>)
                    n480 = Cluster To Array(cluster=w804) -> (array=w797:string[])
                    n481 = call "Dropdown Selection (SubVI).vi"("reference"=w812) -> ("element"=w811:string)
                    n482 = Increment(x=w813) -> (x+1=w810:i32)
                  }
                  frame "BRZ" {
                    w814 = "" ("projNum")
                    # "THREAT"
                    # "Project Name goes here.\nSupports a PB reporting requirement."
                    # "GENERAL"
                    n483 = local read "threatDetails"() -> (w816:T1)
                    n484 = Unbundle By Name(w816) -> ("barrelLength"=w819:string)
                    n485 = Unbundle By Name(w816) -> ("grainSize"=w815:string)
                    n486 = local read "Shot Angle"() -> (w820:u16)
                    n487 = control-ref of="Ballisticians"() -> (w827:refnum<vi>)
                    n488 = control-ref of="ThreatGroups"() -> (w826:refnum<vi>)
                    n489 = control-ref of="PowderTypes"() -> (w825:refnum<vi>)
                    n490 = call "Dropdown Selection (SubVI).vi"("reference"=w827) -> ("element"=w818:string)
                    n491 = call "Dropdown Selection (SubVI).vi"("reference"=w826) -> ("element"=w823:string)
                    n492 = call "Dropdown Selection (SubVI).vi"("reference"=w825) -> ("element"=w822:string)
                    n493 = Format Into String(w820) -> (resulting string=w821:string)  [unwired: 3 in, 1 out]
                    n494 = Bundle("element"=w823, "grainSize"=w815, "element"=w822, "barrelLength"=w819, w821, "element"=w818) -> (w824:T33)  [unwired: 1 out]
                    n495 = local read "LastSample"() -> (w833:i32)
                    n496 = local read "Comments"() -> (w829:string)
                    n497 = local read "ProjectID"() -> (w828:string)
                    n498 = control-ref of="Methods"() -> (w832:refnum<vi>)
                    n499 = Cluster To Array(cluster=w824) -> (array=w817:string[])
                    n500 = call "Dropdown Selection (SubVI).vi"("reference"=w832) -> ("element"=w831:string)
                    n501 = Increment(x=w833) -> (x+1=w830:i32)
                  }
                }
              }
            }
            n502 = Get Date/Time String() -> (date string=w329:string)  [unwired: 3 in, 1 out]
          }
          frame True {
            w849 = ""
            w841 = 16  # dimensions
            w844 = 5  # SampleID
            # "date"
            # "method"
            # "general"
            # "remark"
            # "threat"
            # "shots"
            # "sample"
            # "results"
            # "range"
            # "fabric"
            # "query db with the entered record number and use result to populate the xlt"
            n503 = Not(x=w907) -> (.not. x?=w906:bool)
            n504 = local write "lookupRec"(w906) -> ()
            n505 = Format Into String(format string="SELECT * FROM Experiments\nWHERE expt=%d;" ("query string"), error in=w873, "Record #") -> (resulting string=w903:string, error out=w874:errorcluster)  [unwired: 1 in]
            n506 = call "Fetch Data (SubVI).vi"("error IN"=w874, "query string"=w903) -> ("error OUT"=w872:errorcluster, "recordset data"=w905:string[][])  [unwired: 4 out]
            n507 = Index Array(array=w905) -> (element=w843:string[])  [unwired: 2 in]
            n508 = Index Array(array=w843, index=111) -> (element=w876:string)
            n509 = local read "Set#1 Separation"() -> (w890:sgl)
            n510 = call "Load Shots (SubVI).vi"("Record #"="Record #", "Method"=w876) -> ("Shot Array"=w898:string[][], "AvgDef"=w881:dbl)  [unwired: 1 in]
            n511 = local read "mid_to_targ_dist"() -> (w893:sgl)
            n512 = local read "Barrel to Screen"() -> (w896:sgl)
            n513 = Format Into String(w881) -> (resulting string=w879:string)  [unwired: 3 in, 1 out]
            n514 = Match Pattern(string=w876, regular expression="N.I.J.") -> (offset past match=w878:i32)  [unwired: 4 out]
            n515 = Greater Or Equal To 0?(x=w878) -> (x >= 0?=w875:bool)
            n516 = case shown="False" w875 {
              tunnel: [w918 w919] -> w880
              tunnel: w879 -> [w915 w921]
              tunnel: w843 -> [w917 _]
              frame False {
                n517 = Index Array(array=w917, index #1=124 ("index"), index #2=149 ("index"), index #5=145 ("index")) -> (element #1=w916:string, element #2=w914:string, element #3=w913:string, element #4=w909:string, element #5=w910:string)  [unwired: 2 in]
                n518 = Build Array(w916, w914, w913, w909, w910, w915) -> (w918:string[])
              }
              frame True {
                w920 = "" ("Empty String Constant")
                n519 = Build Array(w920, w920, w920, w920, w920, w921, w921) -> (w919:string[])
              }
            }
            n520 = Divide(x=w890, y=sgl 2.0) -> (x/y=w895:sgl)
            n521 = Add(x=w896, y=w893) -> (x+y=w889:sgl)
            n522 = Subtract(x=w896, y=w895) -> (x-y=w894:sgl)
            n523 = Subtract(x=w893, y=w895) -> (x-y=w892:sgl)
            n524 = Index Array(array=w843, index #1=120 ("index"), index #2=119 ("index"), index #3=127 ("index"), index #4=12 ("index"), index #5=7 ("index")) -> (element #1=w861:string, element #2=w859:string, element #3=w858:string, element #4=w855:string, element #5=w854:string)
            n525 = Index Array(array=w843, index #1=113 ("index"), index #2=112 ("index"), index #3=103 ("index")) -> (element #1=w870:string, element #2=w869:string, element #3=w868:string, element #4=w867:string, element #5=w863:string)  [unwired: 2 in]
            n526 = Format Into String(w889) -> (resulting string=w888:string)  [unwired: 3 in, 1 out]
            n527 = Format Into String(w894) -> (resulting string=w887:string)  [unwired: 3 in, 1 out]
            n528 = Format Into String(w890) -> (resulting string=w886:string)  [unwired: 3 in, 1 out]
            n529 = Format Into String(w892) -> (resulting string=w885:string)  [unwired: 3 in, 1 out]
            n530 = Format Into String(w893) -> (resulting string=w884:string)  [unwired: 3 in, 1 out]
            n531 = Index Array(array=w843, index #1=w844, index #2=w841, index #3=147 ("index"), index #5=148 ("index")) -> (element #1=w842:string, element #2=w839:string, element #3=w838:string, element #5=w835:string)  [unwired: 1 in, 1 out]
            n532 = Build Array(w861, w859, w858, "", w855, w854) -> (w860:string[])
            n533 = Build Array(w888, w887, w886, w885, w884, w870, w869, w868, w867, w863) -> (w883:string[])
            n534 = Index Array(array=w843, index #1=4 ("index"), index #2=111 ("index")) -> (element #1=w850:string, element #2=w847:string)
            n535 = Index Array(array=w843, index=107) -> (element=w899:string)
            n536 = Build Array(w842, w839, w838, "", w835) -> (w840:string[])
            n537 = Index Array(array=w843, index=2) -> (element=w845:string)
            n538 = call "Get Model Construction.vi"("panel record"=w843) -> ("Fabric Array"=w897:string[][])
            n539 = Build Array(w880) -> (w900:string[][])
          }
        }
        n540 = To Variant(anything=w324) -> (Variant=w318:variant)
        n541 = To Variant(anything=w323) -> (Variant=w317:variant)
        n542 = To Variant(anything=w322) -> (Variant=w316:variant)
        n543 = To Variant(anything=w321) -> (Variant=w315:variant)
        n544 = To Variant(anything=w320) -> (Variant=w314:variant)
        n545 = To Variant(anything=w319) -> (Variant=w313:variant)
        n546 = To Variant(anything=w306) -> (Variant=w312:variant)
        n547 = To Variant(anything=w305) -> (Variant=w311:variant)
        n548 = To Variant(anything=w304) -> (Variant=w310:variant)
        n549 = To Variant(anything=w303) -> (Variant=w307:variant)
        n550 = To Variant(anything=w302) -> (Variant=w308:variant)
        n551 = To Variant(anything=w295) -> (Variant=w309:variant)
        n552 = To Variant(anything=w293) -> (Variant=w294:variant)
        n553 = call "TestReport_XL.vi"("Enable"=TRUE, "blockFabric"=w318, "blockRange"=w317, "blockResults"=w316, "blockSample"=w315, "blockShotTbl"=w314, "error in (no error)"=w298, "blockThreat"=w313, "testDate"=w294, "method"=w312, "projName"=w311, "projNum"=w310, "recNum"=w307, "remark"=w308, "standard"=w309) -> ("error out"=w325:errorcluster)  [unwired: 4 in, 8 out]
        n554 = call <vilib>:"Simple Error Handler.vi"("error in (no error)"=w325) -> ("error out"=w327:errorcluster)  [unwired: 1 in, 7 out]
        n555 = case shown="No Error" w327 {
          selector: w327 -> [w922 w924]
          tunnel: [w922 w924] -> w296
          frame No Error {
            n556 = One Button Dialog(message=" V50 Ballistic Test Report is ready") -> ()  [unwired: 2 out]
          }
          frame Error {
          }
        }
      }
      frame 3 {
        w954 = TRUE  # Enable
        # "The custom Excel template file is \nexpected in the C:\\Ballistics folder."
        n557 = stacked-sequence {
          tunnel: [_ _ _ _ _ w1145] -> w947
          tunnel: [_ w1018 _ _ _ _] -> w951
          tunnel: [_ _ _ _ w1102 _] -> w948
          tunnel: [_ _ _ w1069 _ _] -> w949
          tunnel: [_ _ w1040 _ _ _] -> w950
          tunnel: [w962 _ _ _ _ _] -> w952
          tunnel: [_ _ _ _ _ w1166] -> w934
          tunnel: [_ _ _ _ _ "" ("projNum")] -> w933
          tunnel: [_ _ _ _ _ w1161] -> w932
          tunnel: [_ _ _ _ _ w1165] -> w931
          tunnel: [_ _ _ _ _ w1164] -> w930
          tunnel: [_ _ _ _ _ w1163] -> w929
          tunnel: w928 -> [_ _ w1039 _ w1095 _]
          frame #0 {
            # "FABRIC"
            n558 = local read "fab1_totalWt"() -> (w965:sgl)
            n559 = local read "fab3_totalWt"() -> (w967:sgl)
            n560 = local read "fab5_totalWt"() -> (w969:sgl)
            n561 = global read "BIMS_Collector Globals.vi" "LayerStitchTypeRefs"() -> (w957:refnum<vi>[])
            n562 = global read "BIMS_Collector Globals.vi" "SampleAttribs"() -> (w958:T24)
            n563 = global read "BIMS_Collector Globals.vi" "SampleStyles"() -> (w960:refnum<vi>[])
            n564 = local read "fab2_totalWt"() -> (w966:sgl)
            n565 = local read "fab4_totalWt"() -> (w968:sgl)
            n566 = local read "fab6_totalWt"() -> (w970:sgl)
            n567 = global read "BIMS_Collector Globals.vi" "LayerSpecs"() -> (w959:T25)
            n568 = global read "BIMS_Collector Globals.vi" "Mfrs"() -> (w961:refnum<vi>[])
            n569 = Build Array(w965, w966, w967, w968, w969, w970) -> (w964:sgl[])
            n570 = for {
              tunnel: w964 -> [w972] mode=indexing
              tunnel: [w978] -> w963 mode=indexing
              tunnel: w958 -> [w976] mode=indexing
              tunnel: w959 -> [w975] mode=indexing
              tunnel: w961 -> [w974] mode=indexing
              tunnel: w960 -> [w973] mode=indexing
              tunnel: w957 -> [w971] mode=indexing
              n571 = Less Or Equal To 0?(x=w972) -> (x <= 0?=w977:bool)
              n572 = case shown="False" w977 {
                tunnel: [w1000 w1002] -> w978
                tunnel: w976 -> [w999 _]
                tunnel: w975 -> [w984 _]
                tunnel: w974 -> [w993 _]
                tunnel: w973 -> [w990 _]
                tunnel: w972 -> [w983 _]
                tunnel: w971 -> [w979 _]
                frame False {
                  n573 = Unbundle By Name(w984) -> ("numOfPlies"=w982:i32, "LotNum"=w996:string, "RollNum"=w997:string)
                  n574 = Unbundle By Name(w999) -> ("internal_ID"=w987:string, "fiber"=w988:string, "denier"=w995:string, "pick"=w994:string, "weave"=w985:string, "finish"=w986:string, "ozPerYd2"=w998:string)
                  n575 = Format Into String(w982) -> (resulting string=w992:string)  [unwired: 3 in, 1 out]
                  n576 = call "Dropdown Selection (SubVI).vi"("reference"=w993) -> ("element"=w991:string)
                  n577 = call "Dropdown Selection (SubVI).vi"("reference"=w990) -> ("element"=w989:string)
                  n578 = call "Dropdown Selection (SubVI).vi"("reference"=w979) -> ("element"=w980:string)
                  n579 = Format Into String(w983) -> (resulting string=w981:string)  [unwired: 3 in, 1 out]
                  n580 = Build Array(w992, w991, w989, w987, w988, w995, w994, w985, w986, w996, w997, w998, w981, w980) -> (w1000:string[])
                }
                frame True {
                  n581 = call <vilib>:"Space Constant.vi"() -> ("String"=w1003:string)
                  n582 = Initialize Array(w1003, 12 ("dimension size")) -> (w1002:string[])
                }
              }
            }
            n583 = Transpose 2D Array(2D array=w963) -> (transposed array=w962:string[][])
          }
          frame #1 {
            w1004 = "%.1f" ("format string")
            # "muzzel / midpoint"
            # "muzzle / scr#1"
            # "muzzle / target"
            # "scr#2 / target"
            # "RANGE"
            n584 = local read "Set#1 Separation"() -> (w1011:sgl)
            n585 = local read "mid_to_targ_dist"() -> (w1008:sgl)
            n586 = local read "Barrel to Screen"() -> (w1005:sgl)
            n587 = local read "clayAverage"() -> (w1026:sgl)
            n588 = Divide(x=w1011, y=sgl 2.0) -> (x/y=w1006:sgl)
            n589 = local read "RoomHum"() -> (w1021:sgl)
            n590 = local read "clayTemp"() -> (w1024:sgl)
            n591 = local read "clayCalib"() -> (w1027:string)
            n592 = local read "RoomT"() -> (w1022:sgl)
            n593 = Add(x=w1005, y=w1008) -> (x+y=w1012:sgl)
            n594 = Subtract(x=w1005, y=w1006) -> (x-y=w1007:sgl)
            n595 = Subtract(x=w1008, y=w1006) -> (x-y=w1009:sgl)
            n596 = Format Into String(w1012) -> (resulting string=w1013:string)  [unwired: 3 in, 1 out]
            n597 = Format Into String(w1007) -> (resulting string=w1014:string)  [unwired: 3 in, 1 out]
            n598 = Format Into String(w1011) -> (resulting string=w1015:string)  [unwired: 3 in, 1 out]
            n599 = Format Into String(w1009) -> (resulting string=w1016:string)  [unwired: 3 in, 1 out]
            n600 = Format Into String(w1008) -> (resulting string=w1017:string)  [unwired: 3 in, 1 out]
            n601 = Format Into String(w1021) -> (resulting string=w1019:string)  [unwired: 3 in, 1 out]
            n602 = Format Into String(format string=w1004, w1022) -> (resulting string=w1020:string)  [unwired: 2 in, 1 out]
            n603 = Format Into String(format string=w1004, w1024) -> (resulting string=w1023:string)  [unwired: 2 in, 1 out]
            n604 = Format Into String(format string=w1004, w1026) -> (resulting string=w1025:string)  [unwired: 2 in, 1 out]
            n605 = Bundle(w1013, w1014, w1015, w1016, w1017, w1019, w1020, w1023, "clayCalib"=w1027, w1025) -> (w1028:T26)  [unwired: 1 out]
            n606 = Cluster To Array(cluster=w1028) -> (array=w1018:string[])
          }
          frame #2 {
            # "RESULTS"
            n607 = control-ref of="Methods"() -> (w1029:refnum<vi>)
            n608 = call "Dropdown Selection (SubVI).vi"("reference"=w1029) -> ("element"=w1030:string)
            n609 = for {
              tunnel: w1039 -> [w1067] mode=indexing
              tunnel: [w1066] -> w1038 mode=indexing
              tunnel: [w1065] -> w1037
              i -> [w1065]
              n610 = Unbundle By Name(w1067) -> ("BackFace\nDepth"=w1066:sgl)
            }
            n611 = Increment(x=w1037) -> (x+1=w1035:i32)
            n612 = Add Array Elements(numeric array=w1038) -> (sum=w1036:sgl)
            n613 = To Single Precision Float(number=w1035) -> (single precision float=w1034:sgl)
            n614 = Divide(x=w1036, y=w1034) -> (x/y=w1033:sgl)
            n615 = Format Into String(format string="%1.1f", w1033) -> (resulting string=w1032:string)  [unwired: 2 in, 1 out]
            n616 = case shown="\"V50\"" w1030 {
              tunnel: [w1055 w1064] -> w1042
              tunnel: w1032 -> [w1043 w1063]
              frame "V50" {
                w1049 = "%1d" ("format string")
                n617 = local read "Z.M.R."() -> (w1047:sgl)
                n618 = Less Than 0?(x=w1047) -> (x < 0?=w1048:bool)
                n619 = local read "rangeOfResults"() -> (w1051:i32)
                n620 = local read "computed_V50"() -> (w1054:sgl)
                n621 = local read "lowComplete"() -> (w1052:i32)
                n622 = local read "highPartial"() -> (w1053:i32)
                n623 = case shown="True" w1048 {
                  tunnel: w1047 -> [w1060 _]
                  tunnel: [w1060 sgl 0.0 ("Z.M.R.")] -> w1046
                  frame False {
                  }
                  frame True {
                  }
                }
                n624 = Format Into String(format string="%1.1f", w1054) -> (resulting string=w1058:string)  [unwired: 2 in, 1 out]
                n625 = Format Into String(format string=w1049, w1053) -> (resulting string=w1057:string)  [unwired: 2 in, 1 out]
                n626 = Format Into String(format string=w1049, w1052) -> (resulting string=w1056:string)  [unwired: 2 in, 1 out]
                n627 = Format Into String(format string=w1049, w1051) -> (resulting string=w1059:string)  [unwired: 2 in, 1 out]
                n628 = Format Into String(format string="%1.1f", w1046) -> (resulting string=w1045:string)  [unwired: 2 in, 1 out]
                n629 = Bundle(w1058, w1057, w1056, w1059, w1045, w1043, w1043) -> (w1055:T27)  [unwired: 1 out]
              }
              frame Default {
                w1062 = "" ("Empty String Constant")
                n630 = Bundle(w1062, w1062, w1062, w1062, w1062, w1063, w1063) -> (w1064:T27)  [unwired: 1 out]
              }
            }
            n631 = Cluster To Array(cluster=w1042) -> (array=w1041:string[])
            n632 = Build Array(w1041) -> (w1040:string[][])
          }
          frame #3 {
            # "PB Req"
            # "SAMPLE"
            n633 = control-ref of="Methods"() -> (w1070:refnum<vi>)
            n634 = call "Dropdown Selection (SubVI).vi"("reference"=w1070) -> ("element"=w1072:string)
            n635 = Equal?(x=w1072, y="V50") -> (x = y?=w1071:bool)
            n636 = local read "totalSampleWt"() -> (w1082:sgl)
            n637 = case shown="True" w1071 {
              tunnel: ["n/a" w1092] -> w1076
              frame False {
              }
              frame True {
                n638 = local read "minV50"() -> (w1091:i32)
                n639 = Format Into String(w1091) -> (resulting string=w1092:string)  [unwired: 3 in, 1 out]
              }
            }
            n640 = local read "Type of work"() -> (w1068:string)
            n641 = control-ref of="SampleDimensions"() -> (w1088:refnum<vi>)
            n642 = control-ref of="SampleCoverings"() -> (w1089:refnum<vi>)
            n643 = control-ref of="Models"() -> (w1075:refnum<vi>)
            n644 = local read "serialNum"() -> (w1084:string)
            n645 = local read "SampleID"() -> (w1086:string)
            n646 = local read "Thickness"() -> (w1079:dbl)
            n647 = local read "totalBAW"() -> (w1078:sgl)
            n648 = call "Dropdown Selection (SubVI).vi"("reference"=w1088) -> ("element"=w1085:string)
            n649 = call "Dropdown Selection (SubVI).vi"("reference"=w1075) -> ("element"=w1074:string)
            n650 = call "Dropdown Selection (SubVI).vi"("reference"=w1089) -> ("element"=w1083:string)
            n651 = Format Into String(w1082) -> (resulting string=w1081:string)  [unwired: 3 in, 1 out]
            n652 = Format Into String(w1079) -> (resulting string=w1080:string)  [unwired: 3 in, 1 out]
            n653 = Format Into String(w1078) -> (resulting string=w1077:string)  [unwired: 3 in, 1 out]
            n654 = Bundle("SampleID"=w1086, "element"=w1085, "Type of work"=w1068, "serialNum"=w1084, "element"=w1074, w1081, w1080, w1077, "element"=w1083, w1076) -> (w1087:T28)  [unwired: 1 out]
            n655 = Cluster To Array(cluster=w1087) -> (array=w1069:string[])
          }
          frame #4 {
            # "SHOT TABLE"
            n656 = control-ref of="Methods"() -> (w1094:refnum<vi>)
            n657 = call "Dropdown Selection (SubVI).vi"("reference"=w1094) -> ("element"=w1093:string)
            n658 = for {
              tunnel: w1095 -> [w1134] mode=indexing
              shift-right: [w1111] -> _
              shift-left: T18 [] -> [w1113]
              tunnel: [w1111] -> w1098
              tunnel: w1093 -> [w1107]
              n659 = Unbundle By Name(w1134) -> ("shot order"=w1133:i32, "Powder Loading"=w1132:sgl, "Uncorrected Impact"=w1131:sgl, "UncorrectedRed_PB"=w1130:sgl, "UncorrectedAvgVel_PB"=w1129:sgl, "velLoss_PB"=w1128:sgl, "strikeVel_PB"=w1127:sgl, "SHOT STATUS"=w1116:u16, "usedv50"=w1126:bool, "Shot Angle"=w1108:u16, "BackFace\nDepth"=w1109:sgl)
              n660 = case shown="\"V50\"" w1107 {
                tunnel: w1126 -> [w1136 _]
                tunnel: [w1135 w1140] -> w1125
                tunnel: w1108 -> [_ w1139]
                frame "V50" {
                  n661 = case shown="True" w1136 {
                    tunnel: ["" ("Empty String Constant") "*"] -> w1135
                    frame False {
                    }
                    frame True {
                    }
                  }
                }
                frame Default {
                  n662 = Format Into String(w1139) -> (resulting string=w1140:string)  [unwired: 3 in, 1 out]
                }
              }
              n663 = case shown="1" w1116 {
                tunnel: ["P" "C"] -> w1115
                frame 0, Default {
                }
                frame 1 {
                }
              }
              n664 = Format Into String(format string="%2d", w1133) -> (resulting string=w1118:string)  [unwired: 2 in, 1 out]
              n665 = Format Into String(w1132) -> (resulting string=w1119:string)  [unwired: 3 in, 1 out]
              n666 = Format Into String(w1131) -> (resulting string=w1120:string)  [unwired: 3 in, 1 out]
              n667 = Format Into String(w1130) -> (resulting string=w1121:string)  [unwired: 3 in, 1 out]
              n668 = Format Into String(w1129) -> (resulting string=w1122:string)  [unwired: 3 in, 1 out]
              n669 = Format Into String(w1128) -> (resulting string=w1123:string)  [unwired: 3 in, 1 out]
              n670 = Format Into String(w1127) -> (resulting string=w1124:string)  [unwired: 3 in, 1 out]
              n671 = Format Into String(w1109) -> (resulting string=w1117:string)  [unwired: 3 in, 1 out]
              n672 = Build Array(w1118, w1119, w1120, w1121, w1122, w1123, w1124, w1115, w1125, w1117) -> (w1112:string[])
              n673 = Array To Cluster(array=w1112) -> (cluster=w1114:T30)
              n674 = Build Array (concatenate)(w1113, w1114) -> (w1111:T18)
            }
            n675 = Array Size(array=w1098) -> (size(s)=w1100:i32)
            n676 = Equal To 0?(x=w1100) -> (x = 0?=w1096:bool)
            n677 = case shown="True" w1096 {
              tunnel: [w1103 T18 [{"[0]"="", "[1]"="", "[2]"="", "[3]"="", "[4]"="", "[5]"="", "[6]"="", "[7]"="", "[8]"="", "[9]"=""}]] -> w1097
              tunnel: w1098 -> [w1103 _]
              frame False {
              }
              frame True {
              }
            }
            n678 = Sort 1D Array(array=w1097) -> (sorted array=w1099:T18)
            n679 = for {
              tunnel: w1099 -> [w1106] mode=indexing
              tunnel: [w1105] -> w1102 mode=indexing
              n680 = Cluster To Array(cluster=w1106) -> (array=w1105:string[])
            }
          }
          frame #5 {
            # "THREAT"
            # "Range # (supports a PB reporting requirement)"
            # "Project Name goes here.\nSupports a PB reporting requirement."
            # "GENERAL"
            n681 = local read "threatDetails"() -> (w1144:T1)
            n682 = Unbundle By Name(w1144) -> ("barrelLength"=w1148:string)
            n683 = Unbundle By Name(w1144) -> ("grainSize"=w1143:string)
            n684 = local read "Shot Angle"() -> (w1149:u16)
            n685 = control-ref of="WeaponTypes"() -> (w1158:refnum<vi>)
            n686 = control-ref of="ThreatGroups"() -> (w1157:refnum<vi>)
            n687 = control-ref of="PowderTypes"() -> (w1156:refnum<vi>)
            n688 = control-ref of="Recorders"() -> (w1159:refnum<vi>)
            n689 = control-ref of="Shooters"() -> (w1160:refnum<vi>)
            n690 = Format Into String(w1149) -> (resulting string=w1150:string)  [unwired: 3 in, 1 out]
            n691 = call "Dropdown Selection (SubVI).vi"("reference"=w1158) -> ("element"=w1154:string)
            n692 = call "Dropdown Selection (SubVI).vi"("reference"=w1157) -> ("element"=w1153:string)
            n693 = call "Dropdown Selection (SubVI).vi"("reference"=w1156) -> ("element"=w1152:string)
            n694 = call "Dropdown Selection (SubVI).vi"("reference"=w1159) -> ("element"=w1151:string)
            n695 = call "Dropdown Selection (SubVI).vi"("reference"=w1160) -> ("element"=w1147:string)
            n696 = Bundle("element"=w1154, "element"=w1153, "grainSize"=w1143, "element"=w1152, "barrelLength"=w1148, w1150, "element"="1", "element"=w1147, "element"=w1151) -> (w1155:T32)  [unwired: 1 out]
            n697 = Cluster To Array(cluster=w1155) -> (array=w1145:string[])
            n698 = local read "Comments"() -> (w1164:string)
            n699 = local read "ProjectID"() -> (w1161:string)
            n700 = local read "LastSample"() -> (w1169:i32)
            n701 = control-ref of="TestStandards"() -> (w1168:refnum<vi>)
            n702 = control-ref of="Methods"() -> (w1167:refnum<vi>)
            n703 = call "Dropdown Selection (SubVI).vi"("reference"=w1168) -> ("element"=w1163:string)
            n704 = call "Dropdown Selection (SubVI).vi"("reference"=w1167) -> ("element"=w1166:string)
            n705 = Increment(x=w1169) -> (x+1=w1165:i32)
          }
        }
        n706 = To Variant(anything=w952) -> (Variant=w946:variant)
        n707 = To Variant(anything=w951) -> (Variant=w945:variant)
        n708 = To Variant(anything=w950) -> (Variant=w944:variant)
        n709 = To Variant(anything=w949) -> (Variant=w943:variant)
        n710 = To Variant(anything=w948) -> (Variant=w942:variant)
        n711 = To Variant(anything=w947) -> (Variant=w941:variant)
        n712 = To Variant(anything=w934) -> (Variant=w940:variant)
        n713 = To Variant(anything=w933) -> (Variant=w939:variant)
        n714 = To Variant(anything=w932) -> (Variant=w938:variant)
        n715 = To Variant(anything=w931) -> (Variant=w935:variant)
        n716 = To Variant(anything=w930) -> (Variant=w936:variant)
        n717 = To Variant(anything=w929) -> (Variant=w937:variant)
        n718 = call "TestReport_XL.vi"("Enable"=w954, "blockFabric"=w946, "blockRange"=w945, "blockResults"=w944, "blockSample"=w943, "blockShotTbl"=w942, "error in (no error)"=w926, "blockThreat"=w941, "method"=w940, "projName"=w939, "projNum"=w938, "recNum"=w935, "remark"=w936, "standard"=w937) -> ("error out"=w953:errorcluster)  [unwired: 5 in, 8 out]
        n719 = call <vilib>:"Simple Error Handler.vi"("error in (no error)"=w953) -> ("error out"=w955:errorcluster)  [unwired: 1 in, 7 out]
        n720 = case shown="No Error" w955 {
          selector: w955 -> [w1170 w1172]
          tunnel: [w1170 w1172] -> w925
          frame No Error {
            n721 = One Button Dialog(message=" VsVr Ballistic Test Report is ready") -> ()  [unwired: 2 out]
          }
          frame Error {
          }
        }
      }
      frame 4 {
        # "This section saves the shots to the data base"
        n722 = stacked-sequence {
          seq-local: [w1238 _ _] -> [_ w1324 _]
          seq-local: [w1240 _ _] -> [_ w1321 _]
          seq-local: [_ w1309 _] -> [_ _ w1338]
          seq-local: [_ w1311 _] -> [_ _ w1337]
          seq-local: [w1236 _ _] -> [_ _ w1330]
          seq-local: [w1210 _ _] -> [_ w1267 _]
          tunnel: [_ _ w1332] -> w1178
          tunnel: [_ _ w1335] -> w1179
          tunnel: w1174 -> [_ w1276 w1329]
          tunnel: w1176 -> [w1212 _ _]
          tunnel: ["SampleDescrip" _ _] -> _
          tunnel: ["Areal Density" _ _] -> _
          tunnel: ["Areal density text" _ _] -> _
          tunnel: ["SoftwareVersion" _ _] -> _
          tunnel: ["Fabric Description" _ _] -> _
          tunnel: ["Threat" _ _] -> _
          tunnel: ["old threat" _ _] -> _
          tunnel: ["line direction map" _ _] -> _
          tunnel: ["Methods" _ _] -> _
          tunnel: ["SampleCoverings" _ _] -> _
          tunnel: ["Ballisticians" _ _] -> _
          tunnel: ["Submitters" _ _] -> _
          tunnel: ["SampleDimensions" _ _] -> _
          tunnel: ["PowderTypes" _ _] -> _
          tunnel: ["SampleTypes" _ _] -> _
          tunnel: ["TestConditions" _ _] -> _
          tunnel: ["ModelMfrs" _ _] -> _
          tunnel: ["Assemblers" _ _] -> _
          tunnel: ["N.I.J" _ _] -> _
          tunnel: ["SampleClamping" _ _] -> _
          tunnel: ["FrontLayer" _ _] -> _
          tunnel: ["BackLayer" _ _] -> _
          frame #0 {
            # "Legacy requirements:"
            # "Shared requirements:"
            n723 = local read "fab1_totalWt"() -> (w1248:sgl)
            n724 = local read "fab2_totalWt"() -> (w1247:sgl)
            n725 = local read "fab3_totalWt"() -> (w1246:sgl)
            n726 = local read "fab4_totalWt"() -> (w1245:sgl)
            n727 = local read "fab5_totalWt"() -> (w1244:sgl)
            n728 = local read "fab6_totalWt"() -> (w1243:sgl)
            n729 = flat-sequence {
              tunnel: ["TestStandards"] -> _
              tunnel: ["Shooters"] -> _
              tunnel: ["Recorders"] -> _
              tunnel: ["WeaponTypes"] -> _
              tunnel: ["Models"] -> _
              tunnel: ["serialNum"] -> _
              tunnel: ["layerStitch_1"] -> _
              tunnel: ["minV50"] -> _
              tunnel: ["layerStitch_2"] -> _
              tunnel: ["layerStitch_3"] -> _
              tunnel: ["layerStitch_4"] -> _
              tunnel: ["layerStitch_5"] -> _
              tunnel: ["layerStitch_6"] -> _
              frame #0 {
                # "PB-only requirements:"
              }
            }
            n730 = Build Array(w1248, w1247, w1246, w1245, w1244, w1243) -> (w1242:sgl[])
            n731 = call "SQL Statement for Sample Descritpion.vi"("error IN"=w1212, "Layer Weight Array"=w1242, "VALUES clause IN"=" VALUES (%d " ("SQL statement IN"), "INSERT clause IN"="INSERT INTO Experiments " ("SQL statement IN")) -> ("error OUT"=w1211:errorcluster, "VALUES clause OUT"=w1241:string, "INSERT clause OUT"=w1239:string)  [unwired: 1 out]
            n732 = local read "LastSample"() -> (w1237:i32)
            n733 = Increment(x=w1237) -> (x+1=w1236:i32)
            n734 = local read "rangeOfResults"() -> (w1214:i32)
            n735 = local read "lowComplete"() -> (w1215:i32)
            n736 = local read "clayAverage"() -> (w1217:sgl)
            n737 = local read "highPartial"() -> (w1216:i32)
            n738 = control-ref of="SampleClamping"() -> (w1209:refnum<vi>)
            n739 = control-ref of="BackLayer"() -> (w1185:refnum<vi>)
            n740 = control-ref of="FrontLayer"() -> (w1184:refnum<vi>)
            n741 = control-ref of="Ballisticians"() -> (w1231:refnum<vi>)
            n742 = control-ref of="Shooters"() -> (w1227:refnum<vi>)
            n743 = control-ref of="Recorders"() -> (w1226:refnum<vi>)
            n744 = control-ref of="Submitters"() -> (w1230:refnum<vi>)
            n745 = control-ref of="SampleCoverings"() -> (w1223:refnum<vi>)
            n746 = control-ref of="ThreatGroups"() -> (w1222:refnum<vi>)
            n747 = call "Dropdown Selection (SubVI).vi"("reference"=w1231) -> ("element"=w1229:string)
            n748 = call "Dropdown Selection (SubVI).vi"("reference"=w1227) -> ("element"=w1225:string)
            n749 = call "Dropdown Selection (SubVI).vi"("reference"=w1226) -> ("element"=w1224:string)
            n750 = call "Dropdown Selection (SubVI).vi"("reference"=w1230) -> ("element"=w1228:string)
            n751 = call "Dropdown Selection (SubVI).vi"("reference"=w1223) -> ("element"=w1221:string)
            n752 = call "Dropdown Selection (SubVI).vi"("reference"=w1222) -> ("element"=w1220:string)
            n753 = call "Dropdown Selection (SubVI).vi"("reference"=w1209) -> ("element"=w1208:string)
            n754 = call "Dropdown Selection (SubVI).vi"("reference"=w1185) -> ("element"=w1183:string)
            n755 = call "Dropdown Selection (SubVI).vi"("reference"=w1184) -> ("element"=w1182:string)
            n756 = Concatenate Strings(w1239, ", expt, [date], Ballistician1, Ballistician2, Ballistician3, Submitter1, SampleCovering, ProjectileType, ClayTemp, ClayCalibration, ClayAvgThickness, highPartial, lowComplete, rangeOfResults, clamping, FrontPly, BackPly," ("Substring")) -> (w1238:string)
            n757 = Format Into String(format string=", %d, #%s#, '%s', '%s', '%s', '%s', '%s', '%s', %.1f, '%s', %.1f, %d, %d, %d, '%s', '%s', '%s'" ("Format String"), initial string=w1241, error in=w1211, w1236, "currentDateTime", w1229, w1225, w1224, w1228, w1221, w1220, "clayTemp", "clayCalib", w1217, w1216, w1215, w1214, w1208, w1183, w1182) -> (resulting string=w1240:string, error out=w1210:errorcluster)
          }
          frame #1 {
            w1323 = " Angle, Conditions, SampleType, ThreatGrain, ThreatDetail, V50dc, V50, maker, thickness, powder, numshots, backing, totalnumberplys, testcomments, NIJ1, method, temperature, humidity, Dimensions, zmr, ProjectID, SampleID, panelmaker, panelWeight, totalBAW)"  # INSERT clause continued
            # "Although shot angle is defined for the overall\nexperiment, it is also recorded for each shot."
            n758 = local read "computed_V50"() -> (w1319:sgl)
            n759 = local read "Drag Corrected"() -> (w1314:bool)
            n760 = local read "Impact factor"() -> (w1316:sgl)
            n761 = Array Size(array=w1276) -> (size(s)=w1307:i32)
            n762 = Select(t=w1316, s=w1314, f=sgl 1.0) -> (s? t:f=w1315:sgl)
            n763 = Divide(x=w1319, y=w1315) -> (x/y=w1318:sgl)
            n764 = control-ref of="ModelMfrs"() -> (w1302:refnum<vi>)
            n765 = control-ref of="PowderTypes"() -> (w1300:refnum<vi>)
            n766 = call "Dropdown Selection (SubVI).vi"("reference"=w1302) -> ("element"=w1301:string)
            n767 = call "Dropdown Selection (SubVI).vi"("reference"=w1300) -> ("element"=w1284:string)
            n768 = local read "GrainSize"() -> (w1265:u16)
            n769 = local read "Z.M.R."() -> (w1290:sgl)
            n770 = local read "Shot Angle"() -> (w1278:u16)
            n771 = Less Than 0?(x=w1290) -> (x < 0?=w1289:bool)
            n772 = local read "totalNumLayers"() -> (w1306:i32)
            n773 = control-ref of="ThreatDetails"() -> (w1262:refnum<vi>)
            n774 = control-ref of="SampleTypes"() -> (w1272:refnum<vi>)
            n775 = control-ref of="TestConditions"() -> (w1291:refnum<vi>)
            n776 = control-ref of="SampleBackings"() -> (w1299:refnum<vi>)
            n777 = Format Into String(w1265) -> (resulting string=w1264:string)  [unwired: 3 in, 1 out]
            n778 = local read "totalBAW"() -> (w1292:sgl)
            n779 = case shown="True" w1289 {
              tunnel: w1290 -> [w1327 _]
              tunnel: [w1327 sgl 0.0 ("Z.M.R.")] -> w1288
              frame False {
              }
              frame True {
              }
            }
            n780 = control-ref of="SampleDimensions"() -> (w1295:refnum<vi>)
            n781 = control-ref of="N.I.J"() -> (w1297:refnum<vi>)
            n782 = control-ref of="Methods"() -> (w1282:refnum<vi>)
            n783 = control-ref of="Assemblers"() -> (w1293:refnum<vi>)
            n784 = call "Dropdown Selection (SubVI).vi"("reference"=w1262) -> ("element"=w1263:string)
            n785 = call "Dropdown Selection (SubVI).vi"("reference"=w1272) -> ("element"=w1271:string)
            n786 = call "Dropdown Selection (SubVI).vi"("reference"=w1291) -> ("element"=w1277:string)
            n787 = call "Dropdown Selection (SubVI).vi"("reference"=w1299) -> ("element"=w1298:string)
            n788 = Equal?(x=w1264, y="") -> (x = y?=w1286:bool)
            n789 = call "Dropdown Selection (SubVI).vi"("reference"=w1297) -> ("element"=w1296:string)
            n790 = call "Dropdown Selection (SubVI).vi"("reference"=w1282) -> ("element"=w1281:string)
            n791 = call "Dropdown Selection (SubVI).vi"("reference"=w1295) -> ("element"=w1294:string)
            n792 = call "Dropdown Selection (SubVI).vi"("reference"=w1293) -> ("element"=w1283:string)
            n793 = case shown="False" w1286 {
              tunnel: [w1325 "0" ("element")] -> w1285
              tunnel: w1264 -> [w1325 _]
              frame False {
              }
              frame True {
              }
            }
            n794 = call "Prepare DB Connect Path (SubVI).vi"("connectString"=path "BIMS_Collector.udl", "error in"=w1267) -> ("appended path"=w1266:path, "error out"=w1268:errorcluster)  [unwired: 1 out]
            n795 = Format Into String(format string=", %d, '%s', '%s', '%s', '%s', %.4f, %.1f, '%s', %.4f, '%s', %d, '%s', %d, '%s', '%s', '%s', %.1f, %.1f, '%s', %.1f, '%s', '%s', '%s', %.1f, %.1f);" ("Format String"), initial string=w1321, error in=w1268, w1278, w1277, w1271, w1285, w1263, w1319, w1318, w1301, "Thickness", w1284, w1307, w1298, w1306, "Comments", w1296, w1281, "RoomT", "RoomHum", w1294, w1288, "ProjectID", "SampleID", w1283, "totalSampleWt", w1292) -> (resulting string=w1320:string, error out=w1270:errorcluster)
            n796 = call-poly <vilib>:"DB Tools Open Connection.vi"("error in (no error)"=w1270, "connection information"=w1266) -> ("error out"=w1279:errorcluster, "connection reference"=w1280:T34)  [unwired: 3 in, 3 out]
            n797 = Concatenate Strings(w1324, w1323, w1320) -> (w1313:string)
            n798 = call-poly <vilib>:"DB Tools Execute Query.vi"("error in (no error)"=w1279, "SQL query"=w1313, "connection reference"=w1280) -> ("error out"=w1312:errorcluster, "recordset reference"=w1310:T35)  [unwired: 1 in, 4 out]
            n799 = call-poly <vilib>:"DB Tools Free Object.vi"("error in (no error)"=w1312, "recordset reference"=w1310) -> ("error out"=w1311:errorcluster, "connection reference"=w1309:T34)  [unwired: 8 out]
          }
          frame #2 {
            # "Experiment.expt"
            n800 = local read "LastShot"() -> (w1336:i32)
            n801 = Increment(x=w1336) -> (x+1=w1334:i32)
            n802 = for {
              tunnel: w1329 -> [w1382] mode=indexing
              tunnel: w1338 -> [w1357]
              tunnel: w1337 -> [w1341]
              tunnel: [w1355] -> w1331
              tunnel: [w1356] -> w1333
              tunnel: w1334 -> [w1362]
              tunnel: [w1354] -> w1335
              tunnel: w1330 -> [w1350]
              i -> [w1354]
              w1342 = sgl 1.0 ("f")
              # "Shot.id"
              n803 = Add(x=w1362, y=w1354) -> (x+y=w1361:i32)
              n804 = Unbundle By Name(w1382) -> ("IMPACT VELOCITY"=w1368:sgl, "Redundant_Velocity"=w1347:sgl, "RESIDUAL  VELOCITY"=w1346:sgl, "Shot Description"=w1348:string, "Powder Loading"=w1372:sgl, "Barrel Temperature"=w1373:sgl, "TIME / DATE"=w1374:string, "shot order"=w1375:i32, "Shot Angle"=w1376:u16, "BackFace\nDepth"=w1377:sgl, "BackFace\nDiameter"=w1378:sgl, "SHOT STATUS"=w1380:u16, "Projectile Mass"=w1371:sgl, "usedv50"=w1370:bool, "Energy Loss (J)"=w1369:sgl, "avgVel_PB"=w1353:sgl, "velLoss_PB"=w1352:sgl, "strikeVel_PB"=w1351:sgl, "Frag Rod"=w1339:sgl)
              n805 = local read "Drag Corrected"() -> (w1344:bool)
              n806 = local read "Residual factor"() -> (w1366:sgl)
              n807 = local read "Impact factor"() -> (w1343:sgl)
              n808 = Greater Than 0?(x=w1380) -> (x > 0?=w1379:bool)
              n809 = Select(t=w1343, s=w1344, f=w1342) -> (s? t:f=w1364:sgl)
              n810 = Select(t=w1343, s=w1344, f=w1342) -> (s? t:f=w1349:sgl)
              n811 = Select(t=w1366, s=w1344, f=w1342) -> (s? t:f=w1365:sgl)
              n812 = Divide(x=w1368, y=w1364) -> (x/y=w1363:sgl)
              n813 = Divide(x=w1347, y=w1349) -> (x/y=w1345:sgl)
              n814 = Divide(x=w1346, y=w1365) -> (x/y=w1367:sgl)
              n815 = Format Into String(format string="INSERT INTO shots (impactdc, redundantdc, residualdc,  comment, loading, barreltemp, [date], [order], shotangle, bfdepth, bfdiameter, [complete], expt, id, weight,usedv50, loss, residual, impact, redundant, avgVel_PB, velLoss_PB, strikeVel_PB, fragRod)  VALUES (%.1f, %.1f, %.1f, '%s', %.4f, %.1f, #%s#, %d, %d, %.3f, %.3f, %d, %d, %d, %.4f, %d, %.4f, %.1f, %.1f, %.1f, %.1f, %.1f, %.1f, %.1f)" ("Substring"), error in=w1341, w1368, w1347, w1346, w1348, w1372, w1373, w1374, w1375, w1376, w1377, w1378, w1379, w1350, w1361, w1371, w1370, w1369, w1367, w1363, w1345, w1353, w1352, w1351, w1339) -> (resulting string=w1358:string, error out=w1340:errorcluster)  [unwired: 1 in]
              n816 = call-poly <vilib>:"DB Tools Execute Query.vi"("error in (no error)"=w1340, "SQL query"=w1358, "connection reference"=w1357) -> ("error out"=w1360:errorcluster, "recordset reference"=w1359:T35)  [unwired: 1 in, 4 out]
              n817 = call-poly <vilib>:"DB Tools Free Object.vi"("error in (no error)"=w1360, "recordset reference"=w1359) -> ("error out"=w1355:errorcluster, "connection reference"=w1356:T34)  [unwired: 8 out]
            }
            n818 = call <vilib>:"DB Tools Close Connection.vi"("error in (no error)"=w1331, "connection reference"=w1333) -> ("error out"=w1332:errorcluster)  [unwired: 5 out]
          }
        }
        n819 = local read "configPath"() -> (w1177:path)
        n820 = case shown="No Error" w1178 {
          selector: w1178 -> [w1394 w1421]
          tunnel: [-1 -1] -> w1180
          tunnel: [Collector_State."POLL" ("progState") Collector_State."POLL" ("progState")] -> w1181
          tunnel: w1179 -> [w1405 _]
          tunnel: w1177 -> [w1389 _]
          tunnel: [w1388 w1419] -> w1175
          tunnel: w1174 -> [w1386 w1418]
          tunnel: [w1384 w1418] -> w1173
          frame No Error {
            w1395 = "Data Base Parameters" ("section")
            n821 = local read "LastShot"() -> (w1406:i32)
            n822 = Array Size(array=w1386) -> (size(s)=w1385:i32)
            n823 = flat-sequence {
              tunnel: w1388 -> [_]
              tunnel: w1383 -> [w1416]
              tunnel: [w1416] -> w1384
              frame #0 {
                w1409 = T15."Disabled and Grayed Out" ("Disabled")
                n824 = property on="saveReq" class="Str"("Visible"=TRUE) -> ()  [unwired: 2 in, 2 out]
                n825 = local write "SampleID"("") -> ()
                n826 = property on="clearShots" class="Bool"("Disabled"=T15."Enabled") -> ()  [unwired: 2 in, 2 out]
                n827 = property on="addShot" class="Bool"("Disabled"=w1409) -> ()  [unwired: 2 in, 2 out]
                n828 = property on="undoLastShot" class="Bool"("Disabled"=w1409) -> ()  [unwired: 2 in, 2 out]
                n829 = property on="saveShots" class="Bool"("Disabled"=w1409) -> ()  [unwired: 2 in, 2 out]
                n830 = One Button Dialog(message="Data Saved. Enter new Sample ID.") -> ()  [unwired: 1 in, 1 out]
                n831 = property on="mainTabCntrl" class="TabCtl (strict)"("Value"=enum32{"Setup", "Measure", "History", "System"}."Setup" ("mainTabCntrl")) -> ()  [unwired: 2 in, 2 out]
                n832 = property on="SampleEntryTabCntrl" class="TabCtl (strict)"("Value"=enum32{"Environment", "Sample"}."Sample" ("SampleEntryTabCntrl")) -> ()  [unwired: 2 in, 2 out]
                n833 = property on="Sample SubTabCntrl" class="TabCtl (strict)"("Value"=T2."General Specification" ("Sample SubTabCntrl")) -> ()  [unwired: 2 in, 2 out]
              }
            }
            n834 = Increment(x=w1406) -> (x+1=w1400:i32)
            n835 = call <vilib>:"Open Config Data (compatibility).vi"("error in (no error)"=w1394, "configuration file path"=w1389) -> ("error out"=w1399:errorcluster, "refnum"=w1398:T36)  [unwired: 7 in, 1 out]
            n836 = Add(x=w1400, y=w1405) -> (x+y=w1401:i32)
            n837 = local read "LastSample"() -> (w1402:i32)
            n838 = for {
              N: w1385 -> [_]
              shift-right: [w1407] -> w1383
              shift-left: w1386 -> [w1408]
              n839 = Delete From Array(array=w1408) -> (array with subset deleted=w1407:T7[])  [unwired: 2 in, 1 out]
            }
            n840 = local write "LastShot"(w1401) -> ()
            n841 = call-poly <vilib>:"Write Key.vi"("section"=w1395, "error in (no error)"=w1399, "value"=w1401, "key"="Last Shot Saved ", "refnum"=w1398) -> ("error out"=w1397:errorcluster, "refnum out"=w1396:T36)  [unwired: 5 out]
            n842 = Increment(x=w1402) -> (x+1=w1390:i32)
            n843 = local write "LastSample"(w1390) -> ()
            n844 = call-poly <vilib>:"Write Key.vi"("section"=w1395, "error in (no error)"=w1397, "value"=w1390, "key"="Last Panel Saved ", "refnum"=w1396) -> ("error out"=w1387:errorcluster)  [unwired: 6 out]
            n845 = To Double Precision Float(number=w1390) -> (double precision float=w1393:dbl)
            n846 = call <vilib>:"Close Config Data.vi"("error in (no error)"=w1387, "refnum"=w1396) -> ("error out"=w1388:errorcluster)  [unwired: 1 in, 8 out]
            n847 = property on="Record #" class="DigNum (strict)"("Maximum"=w1393) -> ()  [unwired: 2 in, 2 out]
            n848 = property on="SHOTS" class="Arr (strict)"("Val(Sgnl)"=w1383) -> ()  [unwired: 2 in, 2 out]
          }
          frame Error {
            n849 = One Button Dialog(message="Error saving Data. ") -> ()  [unwired: 2 out]
            n850 = call <vilib>:"General Error Handler.vi"("error in (no error)"=w1421) -> ("error out"=w1419:errorcluster)  [unwired: 2 in, 12 out]
          }
        }
      }
      frame 5 {
        # "Shot Order"
        # "This section accepts new data to the shot table."
        n851 = property on="undoLastShot" class="Bool"(error in=w1432, "Disabled"=u8 0) -> (error out=w1431:errorcluster)  [unwired: 1 in, 1 out]
        n852 = local read "residual/speed"() -> (w1457:sgl)
        n853 = local read "Impact/speed"() -> (w1461:sgl)
        n854 = Array Size(array=w1437) -> (size(s)=w1442:i32)
        n855 = Increment(x=w1442) -> (x+1=w1462:i32)
        n856 = case shown="\"grains\"" "loadingUnits" {
          tunnel: [w1469 w1470] -> w1427
          tunnel: "Powder Loading" -> [w1469 w1471]
          frame "grams", Default {
            # "Always save in grams."
          }
          frame "grains" {
            # "Always save in grams."
            n857 = Multiply(x=w1471, y=sgl 0.06479891) -> (x*y=w1470:sgl)
          }
        }
        n858 = local read "Current/residual/speed"() -> (w1445:sgl)
        n859 = local read "CorrectedVelScrnSet2"() -> (w1466:sgl)
        n860 = local read "MeasVelScrnSet2"() -> (w1463:sgl)
        n861 = local read "CorrectedVelScrnSet1"() -> (w1446:sgl)
        n862 = local read "MeasVelScrnSet1"() -> (w1464:sgl)
        n863 = local read "Current/avg/speed"() -> (w1468:sgl)
        n864 = local read "Corrected Residual"() -> (w1444:sgl)
        n865 = local read "BACKFACE DEPTH"() -> (w1448:sgl)
        n866 = local read "Redundant/speed"() -> (w1465:sgl)
        n867 = local read "conversion factor"() -> (w1455:sgl)
        n868 = local read "Projectile Mass"() -> (w1434:sgl)
        n869 = local read "SHOT STATUS"() -> (w1441:u16)
        n870 = local read "Avg/speed"() -> (w1467:sgl)
        n871 = Multiply(x=w1461, y=w1455) -> (x*y=w1453:sgl)
        n872 = Multiply(x=w1455, y=w1457) -> (x*y=w1454:sgl)
        n873 = Multiply(x=w1453, y=w1453) -> (x*y=w1449:sgl)
        n874 = Multiply(x=w1454, y=w1454) -> (x*y=w1450:sgl)
        n875 = Subtract(x=w1449, y=w1450) -> (x-y=w1451:sgl)
        n876 = Format Date/Time String(time format string (%c)="%x   %H:%M:%S") -> (date/time string=w1458:string)  [unwired: 2 out]
        "SUBMIT DATE/TIME" <- w1458
        n877 = Compound Arithmetic op=MULTIPLY(w1434, w1451, sgl 0.0005 ("Input")) -> (w1456:sgl)
        n878 = Index Array(array=w1437) -> (element=w1440:T7)  [unwired: 1 in]
        n879 = Bundle By Name(cluster=w1440, "TIME / DATE"=w1458, "shot order"=w1462, "IMPACT VELOCITY"=w1461, "RESIDUAL  VELOCITY"=w1457, "Shot Description"="Shot Description", "Powder Loading"=w1427, "Barrel Temperature"="Barrel Temp", "SHOT STATUS"=w1441, "BackFace\nDepth"=w1448, "Shot Angle"="Shot Angle", "Uncorrected Impact"=w1464, "Corrected Impact"=w1446, "Uncorrected Residual"=w1445, "Corrected residual"=w1444, "Projectile Mass"=w1434, "Energy Loss (J)"=w1456, "UncorrectedRed_PB"=w1463, "Redundant_Velocity"=w1465, "CorrectedRed_PB"=w1466, "UncorrectedAvgVel_PB"=w1468, "avgVel_PB"=w1467, "Frag Rod"="Frag Rod", "V50userExcl"=FALSE) -> (w1443:T7)
        n880 = Build Array (concatenate)(w1437, w1443) -> (w1433:T7[])
        n881 = stacked-sequence {
          tunnel: w1433 -> [w1476]
          tunnel: [w1476] -> w1424
          tunnel: w1431 -> [w1475]
          tunnel: [w1474] -> w1430
          frame #0 {
            n882 = property on="shotsTabCntrl" class="TabCtl (strict)"(error in=w1475, "Value"=T5."Shots Table" ("shotsTabCntrl")) -> (error out=w1474:errorcluster)  [unwired: 1 in, 1 out]
            n883 = local write "backdepth"(sgl 0.0 ("BACKFACE DEPTH")) -> ()
          }
        }
      }
      frame 6 {
        # "This section will clear the shot table and re-enable the \"ADD SHOT\" button to get ready for a new test panel."
        n884 = Two Button Dialog(message="Shot table cleared even if not saved. Are you sure?", 1:"NO" ("F button name (\"Cancel\")"), 2:"YES" ("T button name (\"OK\")")) -> (T button?=w1481:bool)
        n885 = case shown="True" w1481 {
          tunnel: [w1487 T7[] [] ("SHOTS")] -> w1486
          tunnel: w1482 -> [w1487 _]
          frame False {
          }
          frame True {
            w1488 = T15."Disabled and Grayed Out" ("Disabled")
            n886 = invoke on="Table of Shots" class="Tbl (strict)" method="Reinit To Default"() -> ()  [unwired: 3 in, 3 out]
            n887 = property on="addShot" class="Bool"("Disabled"=T15."Enabled") -> ()  [unwired: 2 in, 2 out]
            n888 = invoke on="SHOTS" class="Arr (strict)" method="Reinit To Default"() -> ()  [unwired: 3 in, 3 out]
            n889 = property on="saveReq" class="Str"("Visible"=TRUE) -> ()  [unwired: 2 in, 2 out]
            n890 = property on="clearShots" class="Bool"("Disabled"=w1488) -> ()  [unwired: 2 in, 2 out]
            n891 = property on="undoLastShot" class="Bool"("Disabled"=w1488) -> ()  [unwired: 2 in, 2 out]
            n892 = property on="saveShots" class="Bool"("Disabled"=w1488) -> ()  [unwired: 2 in, 2 out]
          }
        }
      }
      frame 7 {
        n893 = property on="SHOTS" class="Arr (strict)"(error in=w1494) -> (error out=w1493:errorcluster, "Index Values"=w1498:u32[])  [unwired: 1 in, 1 out]
        n894 = Array Size(array=w1505) -> (size(s)=w1501:i32)
        n895 = Index Array "Index Array"(array=w1498) -> (element=w1503:u32)  [unwired: 1 in]
        n896 = To Unsigned Long Integer(number=w1501) -> (unsigned 32bit integer=w1497:u32)
        n897 = Increment(x=w1503) -> (x+1=w1502:u32)
        n898 = Quotient & Remainder(x=w1502, y=w1497) -> (x-y*floor(x/y)=w1500:u32)  [unwired: 1 out]
        n899 = Replace Array Subset "Replace Array Subset"(array=w1498, new element=w1500) -> (w1499:u32[])  [unwired: 1 in]
        n900 = property on="SHOTS" class="Arr (strict)"(error in=w1493, "Index Values"=w1499) -> (error out=w1492:errorcluster, "Value"=w1504:T7[])  [unwired: 1 in, 1 out]
      }
      frame 8 {
        # "This section undoes new shot data OR deletes the currently accessed previous shot"
        n901 = local read "deleteShot"() -> (w1512:bool)
        n902 = case shown="True" w1512 {
          tunnel: w1511 -> [w1515 w1528]
          tunnel: [w1516 w1529] -> w1510
          frame False {
            n903 = Array Size(array=w1515) -> (size(s)=w1513:i32)
            n904 = while {
              tunnel: [w1519] -> w1514
              tunnel: w1513 -> [w1521]
              tunnel: w1515 -> [w1523] mode=indexing
              i -> [w1519]
              stop <- w1522 stop-if-true
              n905 = Unbundle By Name(w1523) -> ("shot order"=w1520:i32)
              n906 = Equal?(x=w1520, y=w1521) -> (x = y?=w1522:bool)
            }
            n907 = Delete From Array "Delete From Array"(array=w1515, index=w1514) -> (array with subset deleted=w1516:T7[])  [unwired: 1 in, 1 out]
            n908 = local write "SUBMIT DATE/TIME"("" ("Empty String Constant")) -> ()
            n909 = property on="undoLastShot" class="Bool"("Disabled"=u8 2) -> ()  [unwired: 2 in, 2 out]
          }
          frame True {
            n910 = property on="SHOTS" class="Arr (strict)"() -> ("Index Values"=w1537:u32[])  [unwired: 2 in, 2 out]
            n911 = local write "deleteShot"(FALSE) -> ()
            n912 = Index Array(array=w1537, index=0 ("Index")) -> (element=w1527:u32)
            n913 = To Long Integer(number=w1527) -> (32bit integer=w1524:i32)
            n914 = Index Array(array=w1528, index=w1524) -> (element=w1526:T7)
            n915 = Unbundle By Name(w1526) -> ("shot order"=w1525:i32)
            n916 = Format Into String(format string="The currently displayed Shot, #%d", w1525) -> (resulting string=w1534:string)  [unwired: 2 in, 1 out]
            n917 = Concatenate Strings(w1534, ", will be deleted.  IT CANNOT RECOVERED!  Do you want to DELETE the shot?" ("message")) -> (w1533:string)
            n918 = Two Button Dialog(message=w1533, 1:"NO I do NOT want to delete.  Cancel Request" ("F button name (\"Cancel\")"), 2:"YES I want to delete the shot" ("T button name (\"OK\")")) -> (T button?=w1540:bool)
            n919 = case shown="True" w1540 {
              tunnel: w1528 -> [w1553 w1556]
              tunnel: [w1553 w1558] -> w1531
              tunnel: w1524 -> [_ w1555]
              tunnel: [10000 ("shot order") w1557] -> w1530
              frame False {
              }
              frame True {
                n920 = Index Array(array=w1556, index=w1555) -> (element=w1554:T7)
                n921 = Unbundle By Name(w1554) -> ("shot order"=w1557:i32)
                n922 = Delete From Array(array=w1556, index=w1555) -> (array with subset deleted=w1558:T7[])  [unwired: 1 in, 1 out]
              }
            }
            n923 = for {
              tunnel: [w1547] -> w1529 mode=indexing
              tunnel: w1531 -> [w1542] mode=indexing
              tunnel: w1530 -> [w1546]
              n924 = Unbundle By Name(w1542) -> ("shot order"=w1544:i32)
              n925 = Decrement(x=w1544) -> (x-1=w1543:i32)
              n926 = Greater?(x=w1544, y=w1546) -> (0:w1545:bool)
              n927 = case shown="True" w1545 {
                tunnel: w1543 -> [_ w1550]
                tunnel: w1542 -> [w1548 w1551]
                tunnel: [w1548 w1549] -> w1547
                frame False {
                }
                frame True {
                  n928 = Bundle By Name(cluster=w1551, "shot order"=w1550) -> (w1549:T7)
                }
              }
            }
          }
        }
        n929 = property on="SHOTS" class="Arr (strict)"(error in=w1506, "Val(Sgnl)"=w1510) -> (error out=w1507:errorcluster)  [unwired: 1 in, 1 out]
      }
      frame 9 {
        n930 = local write "SUBMIT DATE/TIME"("" ("Empty String Constant")) -> ()
        n931 = Concatenate Strings("L|", "6|") -> (w1565:string)
        n932 = case shown="\"Simulated\", Default" "MeasSrc" {
          tunnel: w1565 -> [_ _ w1581]
          tunnel: w1560 -> [w1571 w1576 w1580]
          tunnel: [w1569 w1576 w1577] -> w1559
          frame "Simulated", Default {
            n933 = flat-sequence {
              tunnel: w1571 -> [w1572]
              tunnel: [w1572] -> w1570
              tunnel: [w1574] -> w1569
              tunnel: w1570 -> [w1574]
              frame #0 {
                n934 = local write "readyClock"(FALSE ("RANGE RESET")) -> ()
              }
              frame #1 {
                n935 = Wait (ms)(milliseconds to wait=u32 100) -> ()  [unwired: 1 out]
              }
            }
          }
          frame "Radar" {
          }
          frame "Screens" {
            w1587 = u32 22 items=["NI-DAQ version", "device name", "base address", "data transfer mode for analog input", "data transfer mode for analog output group 1", "data transfer mode for analog output group 2", "data transfer mode for GPCTR 0", "data transfer mode for GPCTR 1", "data transfer mode for digital I/O group 1", "data transfer mode for digital I/O group 2", "device type code", "DMA A level", "DMA B level", "DMA C level", "interrupt A level", "interrupt B level", "reserved", "lpt device mode", "DAQCard-700 counter 1 source", "interrupt generation mode", "device state during suspend mode", "computer name", "serial number", "counter type", "Scarab A Memory Size", "Scarab B Memory Size"] ("information type")
            w1586 = u32 1  # device
            n936 = Concatenate Strings(w1581, "2|") -> (w1582:string)
            n937 = call <vilib>:"Get DAQ Device Information.vi"("error in (no error)"=w1580, "information type"=w1587, "task ID or device"=w1586) -> ("error out"=w1579:errorcluster, "information string"=w1585:string)  [unwired: 7 out]
            n938 = disable-structure "Diagram Disable Structure" shown="Enabled" {
              disable-tunnel: w1582 -> [w1592 _]
              disable-tunnel: w1579 -> [w1589 w1594]
              disable-tunnel: [w1588 w1594] -> w1578
              frame Disabled {
                n939 = Current VI's Path() -> (path=w1593:path)
                n940 = call "Where Am I (SubVI).vi"("TL Calling Location"=w1592, "Call VI path"=w1593) -> ("I'm here"=w1591:string)
                n941 = call "Error Check (SubVI).vi"("calling VI"=w1591, "tag #"=0, "error IN"=w1589) -> ("error OUT"=w1588:errorcluster)  [unwired: 2 in]
              }
              frame Enabled {
                # "Debug code is disabled"
              }
            }
            n942 = case shown="Error" w1578 {
              selector: w1578 -> [w1595 _]
              tunnel: w1585 -> [w1605 _]
              tunnel: [w1605 "DEVICE NOT READY!" ("information string")] -> w1584
              tunnel: [w1596 errorcluster {"status"=FALSE, "code"=0, "source"=""} ("error out")] -> w1577
              frame No Error {
                # "assign task IDs to counters"
                n943 = call "Config Counter to Measure Two Edge Separation.vi"("error IN"=w1595, "Counter"="Impact Timer", "device"="DAQ Card") -> ("error out"=w1607:errorcluster, "task ID out"=w1601:u32)  [unwired: 1 in]
                "impact/ID" <- w1601
                n944 = local write "readyClock"(FALSE ("RANGE RESET")) -> ()
                n945 = call "Config Counter to Measure Two Edge Separation.vi"("error IN"=w1607, "Counter"="Residual  Timer", "device"="DAQ Card") -> ("error out"=w1609:errorcluster, "task ID out"=w1599:u32)  [unwired: 1 in]
                "residual/ID" <- w1599
                n946 = call "Config Counter to Measure Two Edge Separation.vi"("error IN"=w1609, "Counter"="Redundant Timer", "device"="DAQ Card") -> ("error out"=w1608:errorcluster, "task ID out"=w1600:u32)  [unwired: 1 in]
                "Red/ID" <- w1600
                n947 = Bundle("task ID out"=w1601, "task ID out"=w1600, "task ID out"=w1599) -> (w1597:T37)  [unwired: 1 out]
                n948 = call <vilib>:"Simple Error Handler.vi"("error in (no error)"=w1608) -> ("error out"=w1596:errorcluster)  [unwired: 1 in, 7 out]
                n949 = global write "BIMS_Collector Globals.vi" "Screens"(w1597) -> ()
              }
              frame Error {
                n950 = One Button Dialog(message="Error initializing Timer board.  Switching to simulation") -> ()  [unwired: 2 out]
                n951 = local write "MeasSrc"(DataSource."Simulated" ("MeasSrc")) -> ()
              }
            }
            "Device S/N" <- w1584
          }
        }
      }
      frame 9 {
        n952 = local write "processShots"(FALSE ("ProcessShots")) -> ()
        n953 = local read "Drag Corrected"() -> (w1619:bool)
        n954 = stacked-sequence {
          seq-local: [_ w1677 _ _] -> [_ _ w1709 w1757]
          seq-local: [w1641 _ _ _] -> [_ w1673 _ _]
          seq-local: [w1639 _ _ _] -> [_ w1674 _ _]
          seq-local: [w1640 _ _ _] -> [_ w1675 _ _]
          tunnel: [_ _ _ w1750] -> w1620
          tunnel: w1619 -> [w1643 w1676 _ _]
          tunnel: w1616 -> [_ w1672 _ _]
          tunnel: w1615 -> [w1638 _ _ _]
          tunnel: [w1638 _ _ _] -> w1614
          frame #0 {
            n955 = disable-structure "Diagram Disable Structure" shown="Enabled" {
              disable-tunnel: [w1660 w1667] -> w1648
              frame Disabled {
                n956 = local read "factor array"() -> (w1662:sgl[])
                n957 = local read "Threat"() -> (w1659:u16)
                n958 = To Long Integer(number=w1659) -> (32bit integer=w1661:i32)
                n959 = Index Array(array=w1662, index=w1661) -> (element=w1660:sgl)
              }
              frame Enabled {
                n960 = local read "threatDetails"() -> (w1666:T1)
                n961 = Unbundle By Name(w1666) -> ("dragCorrection"=w1664:string)
                n962 = Not Equal?(x=w1664, y="") -> (x != y?=w1665:bool)
                n963 = case shown="True" w1665 {
                  tunnel: [sgl 1.0 ("default value 1") w1670] -> w1667
                  tunnel: w1664 -> [_ w1669]
                  frame False {
                  }
                  frame True {
                    n964 = Scan From String(input string=w1669, default 1=sgl 0.0 ("default value 1")) -> (output 1=w1670:sgl)  [unwired: 3 in, 3 out]
                  }
                }
              }
            }
            "correction coefficient" <- w1648
            n965 = local read "Current/avg/speed"() -> (w1644:sgl)
            n966 = local read "mid_to_targ_dist"() -> (w1645:sgl)
            n967 = local read "lengthUnits"() -> (w1642:string)
            n968 = call "Compute Strike Velocity.vi"("drag coefficient"=w1648, "decay distance"=w1645, "raw velocity"=w1644, "distance units"=w1642) -> ("correction factor"=w1641:sgl, "strike velocity"=w1646:sgl)  [unwired: 1 out]
            "DC_ factor" <- w1641
            "Corrected Average" <- w1646
            n969 = call "Velocity Correction.vi"("raw impact"="MeasVelScrnSet1", "distance units"=w1642, "raw redundant"="MeasVelScrnSet2", "raw residual"="Current/residual/speed", "screen set midpt to target"="Set#1_to_Target", "residual screen to target"="Residual/Target Dist", "correction coefficient"=w1648) -> ("corrected impact"=w1653:sgl, "corrected redundant"=w1649:sgl, "corrected residual"=w1651:sgl, "impact factor"=w1639:sgl, "conversion factor"=→"conversion factor":sgl, "residual factor"=w1640:sgl)  [unwired: 3 out]
            "Residual factor" <- w1640
            "Impact factor" <- w1639
            "CorrectedVelScrnSet1" <- w1653
            "Corrected Residual" <- w1651
            "CorrectedVelScrnSet2" <- w1649
            n970 = Select(t=w1649, s=w1643, f="MeasVelScrnSet2") -> (s? t:f=→"Redundant/speed":sgl)
            n971 = Select(t=w1646, s=w1643, f=w1644) -> (s? t:f=→"Avg/speed":sgl)
            n972 = Select(t=w1653, s=w1643, f="MeasVelScrnSet1") -> (s? t:f=→"Impact/speed":sgl)
            n973 = Select(t=w1651, s=w1643, f="Current/residual/speed") -> (s? t:f=→"residual/speed":sgl)
            n974 = Add(x="MeasVelScrnSet2", y="MeasVelScrnSet1") -> (x+y=w1625:sgl)
            n975 = Subtract(x="MeasVelScrnSet2", y="MeasVelScrnSet1") -> (x-y=w1624:sgl)
            n976 = Divide(x=w1625, y=sgl 200.0) -> (x/y=w1626:sgl)
            n977 = Divide(x=w1624, y=w1626) -> (x/y=w1630:sgl)
            "%_Difference" <- w1630
            n978 = Absolute Value(x=w1630) -> (abs(x)=w1632:sgl)
            n979 = Less?(x=w1632, y="percent warning") -> (x < y?=w1637:bool)
            n980 = Select(t=u32 65343, s=w1637, f=u32 15668992) -> (s? t:f=w1633:u32)
            n981 = Select(t=u32 0, s=w1637, f=u32 16777226) -> (s? t:f=w1636:u32)
            n982 = property on="%_Difference" class="DigNum (strict)"("Numeric Text.Text Colors:BG Color"=w1633, "NumText.TextColor"=w1636) -> ()  [unwired: 2 in, 2 out]
          }
          frame #1 {
            # "<-- DC_factor (for Average of impact and redundant)"
            # "IF drag corrected THEN apply factors"
            # "Residual factor"
            # "Impact factor\n(also applies to\nredundant velocity)"
            n983 = for {
              tunnel: w1672 -> [w1685] mode=indexing
              tunnel: w1675 -> [w1694]
              tunnel: w1674 -> [w1689]
              tunnel: w1676 -> [w1683]
              tunnel: [w1696] -> w1677 mode=indexing
              tunnel: w1673 -> [w1678]
              n984 = Unbundle By Name(w1685) -> ("UncorrectedAvgVel_PB"=w1684:sgl)
              n985 = Unbundle By Name(w1685) -> ("Uncorrected Impact"=w1688:sgl)
              n986 = Unbundle By Name(w1685) -> ("Uncorrected Residual"=w1693:sgl)
              n987 = Unbundle By Name(w1685) -> ("UncorrectedRed_PB"=w1691:sgl)
              n988 = Multiply(x=w1678, y=w1684) -> (x*y=w1681:sgl)
              n989 = Multiply(x=w1689, y=w1691) -> (x*y=w1690:sgl)
              n990 = Multiply(x=w1689, y=w1688) -> (x*y=w1679:sgl)
              n991 = Multiply(x=w1694, y=w1693) -> (x*y=w1686:sgl)
              n992 = Select(t=w1681, s=w1683, f=w1684) -> (s? t:f=w1682:sgl)
              n993 = Select(t=w1690, s=w1683, f=w1691) -> (s? t:f=w1692:sgl)
              n994 = Select(t=w1686, s=w1683, f=w1693) -> (s? t:f=w1695:sgl)
              n995 = Select(t=w1679, s=w1683, f=w1688) -> (s? t:f=w1687:sgl)
              n996 = Subtract(x=w1682, y=w1681) -> (x-y=w1680:sgl)
              n997 = Bundle By Name(cluster=w1685, "velLoss_PB"=w1680, "strikeVel_PB"=w1681, "avgVel_PB"=w1682, "CorrectedRed_PB"=w1690, "Redundant_Velocity"=w1692, "Corrected Impact"=w1679, "IMPACT VELOCITY"=w1687, "Corrected residual"=w1686, "RESIDUAL  VELOCITY"=w1695) -> (w1696:T7)
            }
          }
          frame #2 {
            w1710 = sgl[] [] ("Partial")
            # "June 2012\n- Lucas Louriero requested \nstdev of velocities used in V50"
            # "This section calculates the V50"
            n998 = for {
              shift-right: [w1732] -> w1712
              shift-left: w1710 -> [w1733]
              shift-right: [w1730] -> w1711
              shift-left: w1710 -> [w1731]
              tunnel: w1709 -> [w1724] mode=indexing
              n999 = Unbundle By Name(w1724) -> ("SHOT STATUS"=w1729:u16)
              n1000 = Unbundle By Name(w1724) -> ("V50userExcl"=w1723:bool)
              n1001 = Unbundle By Name(w1724) -> ("IMPACT VELOCITY"=w1728:sgl)
              n1002 = Unbundle By Name(w1724) -> ("strikeVel_PB"=w1727:sgl)
              n1003 = Select(t=w1727, s="ScreenSetAvgg", f=w1728) -> (s? t:f=w1726:sgl)
              n1004 = case shown="False" w1723 {
                tunnel: w1733 -> [w1739 w1749]
                tunnel: [w1738 w1749] -> w1732
                tunnel: w1731 -> [w1737 w1748]
                tunnel: [w1736 w1748] -> w1730
                tunnel: w1729 -> [w1735 _]
                tunnel: w1726 -> [w1734 _]
                frame False {
                  n1005 = case shown="1" w1735 {
                    tunnel: w1734 -> [w1740 w1744]
                    tunnel: [w1743 w1745] -> w1738
                    tunnel: w1739 -> [w1742 w1745]
                    tunnel: w1737 -> [w1741 w1747]
                    tunnel: [w1741 w1746] -> w1736
                    frame 0, Default {
                      n1006 = Build Array (concatenate)(w1742, w1740) -> (w1743:sgl[])
                    }
                    frame 1 {
                      n1007 = Build Array (concatenate)(w1747, w1744) -> (w1746:sgl[])
                    }
                  }
                }
                frame True {
                }
              }
            }
            n1008 = Sort 1D Array(array=w1712) -> (sorted array=w1722:sgl[])
            n1009 = Sort 1D Array(array=w1711) -> (sorted array=w1698:sgl[])
            "Complete" <- w1698
            n1010 = Reverse 1D Array(array=w1722) -> (reversed array=w1699:sgl[])
            "Partial" <- w1699
            n1011 = Array Size(array=w1698) -> (size(s)=→"#_completes":i32)
            n1012 = Array Size(array=w1699) -> (size(s)=→"#_partials":i32)
            n1013 = Array Max & Min(array=w1699) -> (max value=w1719:sgl)  [unwired: 3 out]
            n1014 = Array Max & Min(array=w1698) -> (min value=w1717:sgl)  [unwired: 3 out]
            n1015 = call "Compute V50.vi"("Partial"=w1699, "Maximum Deviation"="maxDev", "Complete"=w1698) -> ("velSTDEV"=→"velSTDEV":sgl, "Pairs"=→"Pairs":i16, "zmr"=w1700:sgl, "V50"=→"computed_V50":sgl)  [unwired: 1 out]
            "Z.M.R." <- w1700
            n1016 = To Long Integer(number=w1719) -> (32bit integer=→"highPartial":i32)
            n1017 = To Long Integer(number=w1717) -> (32bit integer=→"lowComplete":i32)
            n1018 = Absolute Value(x=w1700) -> (abs(x)=→"zmr 2":sgl)
            n1019 = Less Than 0?(x=w1700) -> (x < 0?=w1703:bool)
            n1020 = Select(t="Low C minus High P", s=w1703, f="ZMR") -> (s? t:f=w1706:string)
            n1021 = Select(t=u32 65336, s=w1703, f=u32 16755266) -> (s? t:f=w1707:u32)
            n1022 = property on="zmr 2" class="DigNum (strict)"("Caption.Text"=w1706, "Numeric Text.Text Colors:BG Color"=w1707) -> ()  [unwired: 2 in, 2 out]
          }
          frame #3 {
            n1023 = local read "Pairs"() -> (w1762:i16)
            n1024 = Sort 1D Array(array=w1757) -> (sorted array=w1760:T7[])
            n1025 = for {
              tunnel: w1760 -> [w1806] mode=indexing
              tunnel: w1762 -> [w1816]
              shift-right: [w1815] -> _
              shift-left: i16 0 -> [w1814]
              tunnel: [w1808] -> w1758 mode=indexing
              # "this section marks the lowest completes that are used in V50"
              n1026 = Unbundle By Name(w1806) -> ("SHOT STATUS"=w1812:u16, "Projectile Mass"=w1810:sgl, "avgVel_PB"=w1809:sgl, "RESIDUAL  VELOCITY"=w1811:sgl)
              n1027 = Unbundle By Name(w1806) -> ("V50userExcl"=w1807:bool)
              n1028 = local read "conversion factor"() -> (w1818:sgl)
              n1029 = case shown="True" w1807 {
                tunnel: w1816 -> [w1829 _]
                tunnel: [w1828 w1838] -> w1815
                tunnel: w1814 -> [w1827 w1838]
                tunnel: [w1826 FALSE] -> w1813
                tunnel: w1812 -> [w1825 _]
                frame False {
                  n1030 = case shown="1" w1825 {
                    tunnel: w1829 -> [_ w1836]
                    tunnel: [FALSE w1835] -> w1826
                    tunnel: [w1831 w1834] -> w1828
                    tunnel: w1827 -> [w1831 w1832]
                    frame 0, Default {
                    }
                    frame 1 {
                      n1031 = Less?(x=w1832, y=w1836) -> (x < y?=w1835:bool)
                      n1032 = Add(x=w1832, y=i16 1 ("t")) -> (x+y=w1834:i16)
                    }
                  }
                }
                frame True {
                }
              }
              n1033 = Multiply(x=w1818, y=w1811) -> (x*y=w1819:sgl)
              n1034 = Multiply(x=w1809, y=w1818) -> (x*y=w1820:sgl)
              n1035 = Multiply(x=w1820, y=w1820) -> (x*y=w1824:sgl)
              n1036 = Multiply(x=w1819, y=w1819) -> (x*y=w1823:sgl)
              n1037 = Subtract(x=w1824, y=w1823) -> (x-y=w1822:sgl)
              n1038 = Compound Arithmetic op=MULTIPLY(w1810, w1822, sgl 0.0005 ("Input")) -> (w1817:sgl)
              n1039 = Bundle By Name(cluster=w1806, "usedv50"=w1813, "Energy Loss (J)"=w1817) -> (w1808:T7)
            }
            n1040 = Reverse 1D Array(array=w1758) -> (reversed array=w1759:T7[])
            n1041 = for {
              tunnel: w1759 -> [w1782] mode=indexing
              tunnel: w1762 -> [w1789]
              shift-right: [w1787] -> _
              shift-left: i16 0 -> [w1788]
              tunnel: [w1785] -> w1750 mode=indexing
              # "chooses highest partials used in v50"
              n1042 = Unbundle By Name(w1782) -> ("SHOT STATUS"=w1790:u16, "usedv50"=w1784:bool)
              n1043 = Unbundle By Name(w1782) -> ("V50userExcl"=w1783:bool)
              n1044 = case shown="True" w1783 {
                tunnel: w1790 -> [w1796 _]
                tunnel: w1789 -> [w1795 _]
                tunnel: w1788 -> [w1794 w1805]
                tunnel: [w1793 w1805] -> w1787
                tunnel: [w1792 FALSE ("usedv50")] -> w1786
                tunnel: w1784 -> [w1791 _]
                frame False {
                  n1045 = case shown="1" w1796 {
                    tunnel: w1795 -> [w1800 _]
                    tunnel: [w1799 w1803] -> w1792
                    tunnel: w1794 -> [w1797 w1802]
                    tunnel: [w1798 w1802] -> w1793
                    tunnel: w1791 -> [_ w1803]
                    frame 0, Default {
                      n1046 = Less?(x=w1797, y=w1800) -> (x < y?=w1799:bool)
                      n1047 = Add(x=w1797, y=i16 1) -> (x+y=w1798:i16)
                    }
                    frame 1 {
                    }
                  }
                }
                frame True {
                }
              }
              n1048 = Bundle By Name(cluster=w1782, "usedv50"=w1786) -> (w1785:T7)
            }
            n1049 = for {
              shift-right: [w1768] -> w1751
              shift-left: sgl[] [] ("Partial") -> [w1765]
              tunnel: w1750 -> [w1767] mode=indexing
              n1050 = local read "ScreenSetAvgg"() -> (w1772:bool)
              n1051 = Unbundle By Name(w1767) -> ("V50userExcl"=w1766:bool, "usedv50"=w1764:bool)
              n1052 = Unbundle By Name(w1767) -> ("IMPACT VELOCITY"=w1770:sgl)
              n1053 = Unbundle By Name(w1767) -> ("strikeVel_PB"=w1771:sgl)
              n1054 = Select(t=w1771, s=w1772, f=w1770) -> (s? t:f=w1769:sgl)
              n1055 = case shown="False" w1766 {
                tunnel: w1769 -> [w1773 _]
                tunnel: [w1774 w1781] -> w1768
                tunnel: w1765 -> [w1775 w1781]
                tunnel: w1764 -> [w1776 _]
                frame False {
                  n1056 = case shown="True" w1776 {
                    tunnel: w1775 -> [w1777 w1780]
                    tunnel: [w1777 w1779] -> w1774
                    tunnel: w1773 -> [_ w1778]
                    frame False {
                    }
                    frame True {
                      n1057 = Build Array (concatenate)(w1780, w1778) -> (w1779:sgl[])
                    }
                  }
                }
                frame True {
                }
              }
            }
            n1058 = Array Max & Min(array=w1751) -> (max value=w1756:sgl, min value=w1755:sgl)  [unwired: 2 out]
            n1059 = Subtract(x=w1756, y=w1755) -> (x-y=w1754:sgl)
            n1060 = property on="SHOTS" class="Arr (strict)"("Val(Sgnl)"=w1750) -> ()  [unwired: 2 in, 2 out]
            n1061 = To Long Integer(number=w1754) -> (32bit integer=→"rangeOfResults":i32)
          }
        }
      }
      frame 11 {
        n1062 = local read "SafetyInterlock"() -> (w1851:cluster{"ARMED":bool})
        n1063 = Unbundle By Name(w1851) -> ("ARMED"=w1850:bool)
        n1064 = Not(x="InterlockExists") -> (.not. x?=w1846:bool)
        n1065 = Or(x=w1850, y=w1846) -> (x .or. y?=w1847:bool)
        n1066 = case shown="True" w1847 {
          tunnel: [Collector_State."POLL" ("progState") w1864] -> w1849
          tunnel: [-1 ("index of element") w1863] -> w1848
          tunnel: "InterlockExists" -> [_ w1862]
          tunnel: [w1855 w1861] -> w1844
          tunnel: w1843 -> [w1855 w1860]
          tunnel: [w1854 w1859] -> w1840
          tunnel: [w1853 w1858] -> w1839
          frame False {
            n1067 = local read "MeasVelScrnSet1"() -> (w1854:sgl)
            n1068 = local read "MeasVelScrnSet2"() -> (w1853:sgl)
          }
          frame True {
            n1069 = stacked-sequence {
              tunnel: [_ Collector_State."PROCESS SHOTS" ("progState")] -> w1864
              tunnel: [_ -1] -> w1863
              tunnel: w1862 -> [w1869 _]
              tunnel: [w1867 _] -> w1861
              tunnel: w1860 -> [w1868 _]
              tunnel: [w1866 _] -> w1859
              tunnel: [w1865 _] -> w1858
              frame #0 {
                n1070 = local read "MeasSrc"() -> (w1870:T6)
                n1071 = case shown="\"Simulated\", Default" w1870 {
                  tunnel: w1869 -> [_ _ w1902]
                  tunnel: w1868 -> [w1872 w1895 w1900]
                  tunnel: [w1872 w1895 w1901] -> w1867
                  tunnel: [w1871 w1894 w1897] -> w1866
                  tunnel: [w1871 w1893 w1896] -> w1865
                  frame "Simulated", Default {
                    # "Simulated"
                    n1072 = local read "minV50"() -> (w1879:i32)
                    n1073 = local read "Powder Loading"() -> (w1892:sgl)
                    n1074 = To Single Precision Float(number=w1879) -> (single precision float=w1878:sgl)
                    n1075 = call "Get Shell Speed.vi"("loading"=w1892, "v50"=w1878) -> ("impact"=w1871:sgl, "residual"=w1887:sgl)  [unwired: 1 in, 2 out]
                    n1076 = Random Number (0-1)() -> (number: 0 to 1=w1885:dbl)
                    n1077 = To Single Precision Float(number=w1885) -> (single precision float=w1881:sgl)
                    n1078 = Multiply(x=w1881, y=sgl 0.002) -> (x*y=w1884:sgl)
                    n1079 = local read "SafetyInterlock"() -> (w1874:cluster{"ARMED":bool})
                    n1080 = Add(x=w1884, y=sgl 0.999) -> (x+y=w1882:sgl)
                    n1081 = Greater Than 0?(x=w1887) -> (x > 0?=w1889:bool)
                    n1082 = Multiply(x=w1871, y=w1882) -> (x*y=w1880:sgl)
                    n1083 = Bundle By Name(cluster=w1874, "ARMED"=FALSE) -> (w1875:cluster{"ARMED":bool})
                    n1084 = Select(t=u16 1, s=w1889, f=u16 0) -> (s? t:f=w1888:u16)
                    n1085 = local write "Current/residual/speed"(w1887) -> ()
                    n1086 = local write "SHOT STATUS"(w1888) -> ()
                    n1087 = local write "Current/sthotstatus"(w1888) -> ()
                    n1088 = local write "MeasVelScrnSet1"(w1871) -> ()
                    n1089 = local write "MeasVelScrnSet2"(w1880) -> ()
                    n1090 = local write "readyClock"(TRUE ("RANGE RESET")) -> ()
                    n1091 = local write "SafetyInterlock"(w1875) -> ()
                    n1092 = Wait (ms)(milliseconds to wait=u32 500 ("number")) -> ()  [unwired: 1 out]
                  }
                  frame "Radar" {
                    # "Radar -- (future)"
                    n1093 = local read "MeasVelScrnSet1"() -> (w1894:sgl)
                    n1094 = local read "MeasVelScrnSet2"() -> (w1893:sgl)
                  }
                  frame "Screens" {
                    # "This section checks to see if the counters have been fired.  If they have then the counter times are read"
                    n1095 = Concatenate Strings("-1|", "F0|") -> (w1904:string)
                    n1096 = case shown="True" w1902 {
                      tunnel: w1900 -> [w1911 w1912]
                      tunnel: [w1911 w1912] -> w1899
                      frame False {
                      }
                      frame True {
                      }
                    }
                    n1097 = global read "BIMS_Collector Globals.vi" "Screens"() -> (w1903)
                    n1098 = Unbundle By Name(w1903) -> ("ScrnSet1CntrID"=w1907)
                    n1099 = Concatenate Strings(w1904, "2|") -> (w1908:string)
                    n1100 = call "Check DAQ Status.vi"("errIN"=w1899, "TL Calling Location"=w1908, "Task ID"=w1907) -> ("error out"=w1910:errorcluster, "Armed?"=w1898:bool)  [unwired: 1 out]
                    n1101 = case shown="False" w1898 {
                      tunnel: w1910 -> [w1937 w1977]
                      tunnel: w1907 -> [w1920 _]
                      tunnel: w1908 -> [w1933 _]
                      tunnel: w1903 -> [w1923 _]
                      tunnel: [w1915 w1977] -> w1901
                      tunnel: [w1913 w1976] -> w1897
                      tunnel: [w1914 w1975] -> w1896
                      frame False {
                        n1102 = local read "Set#1 Separation"() -> (w1940:sgl)
                        n1103 = Concatenate Strings(w1933, "F|") -> (w1928:string)
                        n1104 = call "Read TIO Count.vi"("TL Calling Location"=w1928, "error In"=w1937, "task IN"=w1920) -> ("error out"=w1922:errorcluster, "time (secs)"=w1942:sgl)  [unwired: 1 in, 4 out]
                        n1105 = Divide(x=w1940, y=w1942) -> (x/y=w1913:sgl)
                        n1106 = call "Arm TIO Channel.vi"("error IN"=w1922, "task ID IN"=w1920) -> ("error out"=w1921:errorcluster)  [unwired: 1 in, 2 out]
                        n1107 = Unbundle By Name(w1923) -> ("ScrnSet2CntrID"=w1925)
                        n1108 = local write "MeasVelScrnSet1"(w1913) -> ()
                        n1109 = Concatenate Strings(w1928, "a|") -> (w1931:string)
                        n1110 = call "Check DAQ Status.vi"("errIN"=w1921, "TL Calling Location"=w1931, "Task ID"=w1925) -> ("error out"=w1936:errorcluster, "Armed?"=w1927:bool)  [unwired: 1 out]
                        n1111 = case shown="False" w1927 {
                          tunnel: [w1953 sgl 0.0] -> w1914
                          tunnel: w1936 -> [w1952 w1957]
                          tunnel: [w1947 w1957] -> w1938
                          tunnel: w1925 -> [w1946 _]
                          tunnel: w1928 -> [w1950 _]
                          frame False {
                            n1112 = local read "Set#2 Separation"() -> (w1954:sgl)
                            n1113 = Concatenate Strings(w1950, "Fa|") -> (w1949:string)
                            n1114 = call "Read TIO Count.vi"("TL Calling Location"=w1949, "error In"=w1952, "task IN"=w1946) -> ("error out"=w1948:errorcluster, "time (secs)"=w1955:sgl)  [unwired: 1 in, 4 out]
                            n1115 = Divide(x=w1954, y=w1955) -> (x/y=w1953:sgl)
                            n1116 = call "Arm TIO Channel.vi"("error IN"=w1948, "task ID IN"=w1946) -> ("error out"=w1947:errorcluster)  [unwired: 1 in, 2 out]
                          }
                          frame True {
                          }
                        }
                        n1117 = Unbundle By Name(w1923) -> ("residualCntrID"=w1924)
                        n1118 = local write "MeasVelScrnSet2"(w1914) -> ()
                        n1119 = Concatenate Strings(w1928, "b|") -> (w1929:string)
                        n1120 = call "Check DAQ Status.vi"("errIN"=w1938, "TL Calling Location"=w1929, "Task ID"=w1924) -> ("error out"=w1935:errorcluster, "Armed?"=w1926:bool)  [unwired: 1 out]
                        n1121 = case shown="True" w1926 {
                          tunnel: w1935 -> [w1964 w1973]
                          tunnel: [w1969 w1974] -> w1941
                          tunnel: w1924 -> [w1959 _]
                          tunnel: [w1958 w1973] -> w1916
                          tunnel: [w1966 sgl 0.0] -> w1939
                          tunnel: w1928 -> [w1961 _]
                          frame False {
                            w1970 = u16 1 items=["Partial", "Complete"] ("SHOT STATUS")
                            w1971 = u16 0 items=["Partial", "Complete"] ("SHOT STATUS")
                            n1122 = local read "Residual/Separation"() -> (w1965:sgl)
                            n1123 = Concatenate Strings(w1961, "Fb|") -> (w1962:string)
                            n1124 = call "Read TIO Count.vi"("TL Calling Location"=w1962, "error In"=w1964, "task IN"=w1959) -> ("error out"=w1960:errorcluster, "timeout"=w1967:bool, "time (secs)"=w1968:sgl)  [unwired: 1 in, 3 out]
                            n1125 = Divide(x=w1965, y=w1968) -> (x/y=w1966:sgl)
                            n1126 = call "Arm TIO Channel.vi"("error IN"=w1960, "task ID IN"=w1959) -> ("error out"=w1958:errorcluster)  [unwired: 1 in, 2 out]
                            n1127 = Select(t=w1971, s=w1967, f=w1970) -> (s? t:f=w1969:u16)
                          }
                          frame True {
                            w1974 = u16 1 items=["Partial", "Complete"] ("SHOT STATUS")
                          }
                        }
                        n1128 = local write "Current/residual/speed"(w1939) -> ()
                        n1129 = local write "SHOT STATUS"(w1941) -> ()
                        n1130 = local write "Current/sthotstatus"(w1941) -> ()
                        n1131 = case shown="No Error" w1916 {
                          selector: w1916 -> [w1945 _]
                          frame No Error {
                            # "=false"
                            n1132 = Unbundle By Name(w1945) -> ("status"=w1944:bool)
                            n1133 = Not(x=w1944) -> (.not. x?=w1943:bool)
                            n1134 = local write "readyClock"(w1943) -> ()
                          }
                          frame Error {
                          }
                        }
                        n1135 = local read "SafetyInterlock"() -> (w1917:cluster{"ARMED":bool})
                        n1136 = Bundle By Name(cluster=w1917, "ARMED"=FALSE) -> (w1918:cluster{"ARMED":bool})
                        n1137 = local write "SafetyInterlock"(w1918) -> ()
                        n1138 = call <vilib>:"Simple Error Handler.vi"("error in (no error)"=w1916) -> ("error out"=w1915:errorcluster)  [unwired: 1 in, 7 out]
                      }
                      frame True {
                        # "Error -10600 occurrs in \"Read Count.vi\"\n\n  Possible reason(s): NI-DAQ LV: No setup operation has been performed for the specified resources. Or, some resources require a specific ordering of calls for proper setup.  \n\n  Solution: To avoid this error, you must call the Dig_Line_Config function to setup the direction for each digital line prior to calling the Dig_Grp_Config function."
                        n1139 = local read "MeasVelScrnSet1"() -> (w1976:sgl)
                        n1140 = local read "MeasVelScrnSet2"() -> (w1975:sgl)
                      }
                    }
                  }
                }
              }
              frame #1 {
              }
            }
          }
        }
        n1141 = control-ref of="2ndScreen"() -> (w1841:refnum<vi>)
        n1142 = call "2nd screen effect (SubVI).vi"("MeasVelScrnSet 2"=w1839, "MeasVelScrnSet 1"=w1840, "2nd Screen ref"=w1841) -> ("MeasVelOut"=→"Current/avg/speed":sgl)
      }
    }
    "SMErr" <- w13
  }
  n1143 = while "U/I Event Handler" {
    shift-right: [w1981] -> _
    shift-left: w7 -> [w1982]
    stop <- FALSE stop-if-true
    n1144 = event shown="[24] \"RefreshMetadata\": Value Change" {
      selector: _ -> [_ _ _ _ _ _ _ _ _ _ _ _ _ _ _ _ _ _ _ _ _ _ _ _ _ _ _]
      dyn-events: _ -> [_ _ _ _ _ _ _ _ _ _ _ _ _ _ _ _ _ _ _ _ _ _ _ _ _ _ _]
      timeout: 100 -> [_ _ _ _ _ _ _ _ _ _ _ _ _ _ _ _ _ _ _ _ _ _ _ _ _ _ _]
      tunnel: w1982 -> [w1986 _ w2003 w2013 w2022 w2032 w2069 w2095 w2102 w2128 w2167 w2210 w2249 w2252 w2289 w2326 w2330 w2340 w2368 w2374 w2380 w2406 w2425 w2428 w2456 w2488 _]
      tunnel: [w1986 w1990 w2003 w2010 w2021 w2031 w2068 w2094 w2100 w2137 w2166 w2207 w2249 w2252 w2289 w2326 w2329 w2336 w2368 w2374 w2377 w2403 w2425 w2428 w2458 w2488 w2496] -> w1981
      tunnel: [FALSE ("UpdateMetadata") "EXIT" "diagPageVisible" "runtimeMenusVisible" "ARM" "QueryLoad" FALSE ("UpdateMetadata") FALSE ("UpdateMetadata") FALSE ("UpdateMetadata") FALSE ("UpdateMetadata") FALSE ("UpdateMetadata") FALSE ("UpdateMetadata") FALSE ("UpdateMetadata") FALSE ("UpdateMetadata") FALSE ("UpdateMetadata") FALSE ("UpdateMetadata") FALSE ("UpdateMetadata") FALSE ("UpdateMetadata") "Drag Corrected" _ FALSE ("UpdateMetadata") "PublishNewRecords" FALSE ("UpdateMetadata") FALSE ("UpdateMetadata") "RefreshMetadata" FALSE ("UpdateMetadata") FALSE ("UpdateMetadata")] -> w1980
      event Timeout {
        n1145 = event-data() -> ()  [unwired: 2 out]
        n1146 = Get Date/Time In Seconds() -> (seconds since 1Jan1904=w1988:timestamp)
        n1147 = Format Date/Time String(seconds (now)=w1988) -> (date/time string=→"TimeNow":string)  [unwired: 2 out]
      }
      event "EXIT": Value Change {
        n1148 = event-data() -> ()  [unwired: 2 out]
        n1149 = property on="Property Node" class="Application"(error in=errorcluster {"status"=FALSE, "code"=0, "source"=""} ("error in (no error)")) -> (error out=w1990:errorcluster, "Application:Kind"=w1995:T38)  [unwired: 1 in, 1 out]
        n1150 = Two Button Dialog(message="Exit BIMS Collector?\nAll Unsaved data will be lost.", 1:"NO" ("F button name (\"Cancel\")"), 2:"YES" ("T button name (\"OK\")")) -> (T button?=w1996:bool)
        n1151 = case shown="\"Development System\"" w1995 {
          tunnel: w1996 -> [w1997 w1998 w1999]
          frame Default {
            n1152 = Stop(stop? (T)=w1997) -> ()
          }
          frame "Development System" {
            n1153 = Stop(stop? (T)=w1998) -> ()
          }
          frame "Run Time System" {
            n1154 = Quit LabVIEW(quit? (T)=w1999) -> ()
          }
        }
      }
      event "diagPageVisible": Value Change {
        # "Toggles display of \"Internal Use\" tab for diagnostics purposes"
        # "Key navigation ONLY: Cntrl-Shift-F11"
        n1155 = event-data() -> ("NewVal"=w2006:bool)  [unwired: 1 out]
        n1156 = property on="aboutTabCntrl" class="TabCtl (strict)"(error in=errorcluster {"status"=FALSE, "code"=0, "source"=""} ("error in (no error)")) -> (error out=w2005:errorcluster, "Pages"=w2009:refnum<vi>[])  [unwired: 1 in, 1 out]
        n1157 = Index Array(array=w2009, index=3) -> (element=w2007:refnum<vi>)
        n1158 = property on="Property Node" class="Page"(reference=w2007, error in=w2005, "PageVis"=w2006) -> (error out=w2004:errorcluster)  [unwired: 1 out]
        n1159 = property on="diagPageVisible" class="Bool (strict)"(error in=w2004, "Value"=w2006) -> (error out=w2001:errorcluster)  [unwired: 1 in, 1 out]
        n1160 = call <vilib>:"General Error Handler.vi"("error in (no error)"=w2001) -> ()  [unwired: 2 in, 13 out]
      }
      event "runtimeMenusVisible": Value Change {
        # "Key navigation ONLY: Cntrl-Shift-F10"
        n1161 = event-data() -> ("NewVal"=w2015:bool)  [unwired: 1 out]
        n1162 = control-ref of="This VI"() -> (w2014:refnum<vi>)
        n1163 = property class="VI"(reference=w2014, error in=w2013, "Front Panel.ShowMenuBar"=w2015) -> (reference out=w2012:refnum<vi>, error out=w2011:errorcluster)
        n1164 = Close Reference(reference=w2012, error in (no error)=w2011) -> (error out=w2010:errorcluster)
      }
      event "ARM": Value Change {
        # "This section will arm the system"
        n1165 = event-data() -> ()  [unwired: 2 out]
        n1166 = disable-structure shown="Disabled" {
          frame Disabled {
            "DIO" <- u32 21 ("DIO")
          }
          frame Enabled {
          }
        }
        n1167 = Bundle By Name(cluster=cluster{"ARMED":bool} {"ARMED"=FALSE} ("Safety_Interlock"), "ARMED"=TRUE) -> (→"SafetyInterlock":cluster{"ARMED":bool})
        n1168 = local write "SUBMIT DATE/TIME"("" ("Empty String Constant")) -> ()
        n1169 = local read "MeasSrc"() -> (w2023:T6)
        n1170 = case shown="\"Screens\"" w2023 {
          tunnel: w2022 -> [w2026 w2027 w2029]
          tunnel: [w2026 w2027 w2029] -> w2021
          frame "Simulated", Default {
          }
          frame "Radar" {
          }
          frame "Screens" {
            n1171 = local write "readyClock"(TRUE ("readyClock")) -> ()
          }
        }
      }
      event "QueryLoad": Value Change {
        w2037 = "%x" ("time format string (%c)")
        w2053 = "" ("replace string (\"\")")
        # "This section plots  Impact velocity vs. loadingdata"
        n1172 = event-data() -> ()  [unwired: 2 out]
        n1173 = Format Date/Time String(time format string (%c)=w2037, seconds (now)="lkupStartDate") -> (date/time string=w2036:string)  [unwired: 1 out]
        n1174 = Format Date/Time String(time format string (%c)=w2037, seconds (now)="lkupEndDate") -> (date/time string=w2035:string)  [unwired: 1 out]
        n1175 = call "Trim String.vi"("inStr"="Powder.freeTxt") -> ("outStr"=w2051:string)
        n1176 = call "Trim String.vi"("inStr"="Threat.freeTxt") -> ("outStr"=w2052:string)
        n1177 = invoke on="v50_table" class="Tbl" method="Reinit To Default"(error in=w2032) -> (error out=w2044:errorcluster)  [unwired: 2 in, 2 out]
        n1178 = invoke on="Vel.vs.Loading" class="WFGraph (strict)" method="Reinit To Default"(error in=w2044) -> (error out=w2039:errorcluster)  [unwired: 2 in, 2 out]
        n1179 = Format Into String(format string="SELECT TOP %d dbsrc.experiment.threat, dbsrc.shots.loading, dbsrc.shots.impact, dbsrc.experiment.powder, dbsrc.shots.date from dbsrc.shots, dbsrc.experiment where dbsrc.shots.expt = dbsrc.experiment.expt and dbsrc.shots.loading > 0 and dbsrc.shots.date between '%s' and '%s' and dbsrc.shots.impact between 10 and 5000 and dbsrc.experiment.powder like '%%%s%%' and dbsrc.experiment.threat like '%%%s%%' and experiment.threat<>'' order by dbsrc.experiment.threat, dbsrc.shots.loading, dbsrc.shots.impact;" ("Format String"), error in=w2039, "maxRecs", w2036, w2035, w2051, w2052) -> (resulting string=w2057:string, error out=w2042:errorcluster)  [unwired: 1 in]
        n1180 = Search and Replace String(input string=w2057, search string=" and experiment.powder like '%%'", replace string=w2053, error in=w2042) -> (result string=w2055:string, error out=w2043:errorcluster)  [unwired: 6 out]
        n1181 = Search and Replace String(input string=w2055, search string="and experiment.threat like '%%'", replace string=w2053, error in=w2043) -> (result string=w2046:string, error out=w2041:errorcluster)  [unwired: 6 out]
        n1182 = call "Fetch Data (SubVI).vi"("error IN"=w2041, "query string"=w2046) -> ("error OUT"=w2031:errorcluster, "recordset data"=w2047:string[][])  [unwired: 4 out]
        "v50_table" <- w2047
        n1183 = Fract/Exp String To Number(string=w2047) -> (number=w2061:dbl[][])  [unwired: 4 out]
        n1184 = Array Size(array=w2047) -> (size(s)=w2049:i32[])
        n1185 = Index Array(array=w2049) -> (element=→"ActualNumRecs":i32)  [unwired: 1 in]
        n1186 = Index Array(array=w2061, index (col)=2 ("Disabled Index (col)")) -> (element=w2060:dbl[])  [unwired: 1 in]
        n1187 = Index Array(array=w2061, index (col)=1 ("Disabled Index (col)")) -> (element=w2059:dbl[])  [unwired: 1 in]
        n1188 = Bundle(w2059, w2060) -> (→"Vel.vs.Loading":cluster{dbl[], dbl[]})  [unwired: 1 out]
      }
      event "ThreatGroups": Value Change {
        n1189 = event-data() -> ()  [unwired: 2 out]
        n1190 = control-ref of="ThreatGroups"() -> (w2070:refnum<vi>)
        n1191 = property on="Property Node" class="Ring (strict)"(reference=w2070, error in=w2069) -> (error out=w2067:errorcluster, "RingText.Text"=w2065:string)  [unwired: 1 out]
        n1192 = Not Equal?(x=w2065, y="") -> (x != y?=w2064:bool)
        n1193 = case shown="True" w2064 {
          tunnel: w2065 -> [_ w2080]
          tunnel: [w2072 w2078] -> w2068
          tunnel: w2067 -> [w2075 w2077]
          frame False {
            n1194 = property on="ThreatDetails" class="Ring (strict)"(error in=w2075, "Strings []"=string[] [], "Value"=u16 0 ("Value (Signaling)")) -> (error out=w2073:errorcluster)  [unwired: 1 in, 1 out]
            n1195 = invoke on="threatDetails" class="Clust (strict)" method="Reinit To Default"(error in=w2073) -> (error out=w2072:errorcluster)  [unwired: 2 in, 2 out]
          }
          frame True {
            n1196 = call "Select Threat Details.vi"("threatGroup"=w2080) -> ("threatDetails"=w2079:string[])  [unwired: 1 out]
            n1197 = property on="ThreatDetails" class="Ring (strict)"(error in=w2077, "Strings []"=w2079, "Val(Sgnl)"=u16 0 ("Value (Signaling)")) -> (error out=w2078:errorcluster)  [unwired: 1 in, 1 out]
          }
        }
      }
      event "panelSearch": Value Change {
        # "This section returns past panels"
        n1198 = event-data() -> ()  [unwired: 2 out]
        n1199 = control-ref of="pastPanels"() -> (w2097:refnum<vi>)
        n1200 = control-ref of="Mfr_0"() -> (w2091:refnum<vi>)
        n1201 = control-ref of="SampleStyle_0"() -> (w2092:refnum<vi>)
        n1202 = control-ref of="Requestors_0"() -> (w2090:refnum<vi>)
        n1203 = control-ref of="ThreatSize_0"() -> (w2089:refnum<vi>)
        n1204 = call "queryPanels (SubVI).vi"("ThreatSize_0"=w2089, "Mfr_0"=w2091, "Requestors_0"=w2090, "Style_0"=w2092, "error in"=w2095, "srchParams"="srchParams", "pastPanels"=w2097) -> ("error out"=w2094:errorcluster, "recordset data"=w2088:string[][], "actualNumPanels"=→"actualNumPanels":i32)  [unwired: 2 in]
        "pastPanels" <- w2088
        n1205 = Index Array(array=w2088) -> (element=w2082:string[])  [unwired: 2 in]
        n1206 = Array Size(array=w2082) -> (size(s)=w2087:i32)
        n1207 = Greater Than 0?(x=w2087) -> (x > 0?=w2086:bool)
        n1208 = Select(t=T15."Enabled" ("Disabled"), s=w2086, f=T15."Disabled and Grayed Out" ("Disabled")) -> (s? t:f=w2085:T15)
        n1209 = property on="reportV50_History" class="Bool"("DisabledEnum"=w2085) -> ()  [unwired: 2 in, 2 out]
      }
      event "pastPanels": Mouse Up {
        n1210 = event-data() -> ("CtlRef"=w2110:refnum<vi>)  [unwired: 1 out]
        n1211 = property on="Property Node" class="Tbl (strict)"(reference=w2110, error in=w2102) -> (error out=w2101:errorcluster, "Value"=w2109:string[][], "EditPos"=w2108:T39)  [unwired: 1 out]
        n1212 = Unbundle By Name(w2108) -> ("Row"=w2107:i32)
        n1213 = Index Array(array=w2109, index (row)=w2107, index (col)=0 ("disabled index (col)")) -> (element=w2106:string)
        n1214 = Scan From String(input string=w2106, error in=w2101, default 1=1 ("Record #")) -> (error out=w2100:errorcluster, output 1=w2104:i32)  [unwired: 2 in, 2 out]
        n1215 = local write "Record #"(w2104) -> ()
      }
      event "ThreatDetails", "SampleID": Value Change {
        # "A Sample ID is entered"
        # "A range is selected"
        # "A measurement requires the selection of a threat,\nso delay enabling the \"Measure\" tab until a grain wt\nis chosen."
        n1216 = event-data() -> ()  [unwired: 2 out]
        n1217 = control-ref of="ThreatGroups"() -> (w2129:refnum<vi>)
        n1218 = control-ref of="ThreatDetails"() -> (w2126:refnum<vi>)
        n1219 = call "Get Projectile Atributes from ThreatGroupDetail.vi"("error IN"=w2128, "ThreatDetail"=w2126, "ThreatGroup"=w2129) -> ("error out"=w2127:errorcluster, "projectileAttribs"=w2125:T40)  [unwired: 1 out]
        "threatDetails" <- w2125
        n1220 = Unbundle By Name(w2125) -> ("grainSize"=w2118:string)
        n1221 = Equal?(x=w2118, y="") -> (x = y?=w2119:bool)
        n1222 = case shown="False" w2119 {
          tunnel: w2118 -> [w2147 _]
          tunnel: [w2146 u16 0 ("GrainSize")] -> w2124
          frame False {
            # "A grain size is selected"
            n1223 = Scan From String(input string=w2147) -> (output 1=w2146:u16)  [unwired: 3 in, 4 out]
            "GrainSize" <- w2146
          }
          frame True {
            # "A grain size not selected"
          }
        }
        n1224 = Equal?(x=w2118, y="") -> (x = y?=w2144:bool)
        n1225 = local read "rangeSetup"() -> (w2141:u16)
        n1226 = case shown="False" w2144 {
          tunnel: [w2151 sgl 0.0] -> w2140
          tunnel: w2118 -> [w2149 _]
          frame False {
            w2153 = sgl 0.0  # sgl
            n1227 = Scan From String(format string="%f " ("Format String"), input string=w2149, default 1=w2153) -> (output 1=w2152:sgl)  [unwired: 2 in, 3 out]
            n1228 = disable-structure shown="Enabled" {
              disable-tunnel: w2152 -> [w2156 w2157]
              disable-tunnel: [w2155 w2157] -> w2151
              frame Disabled {
                n1229 = Multiply(x=sgl 0.06479891, y=w2156) -> (x*y=w2155:sgl)
              }
              frame Enabled {
              }
            }
          }
          frame True {
          }
        }
        "Projectile Mass" <- w2140
        n1230 = local read "SampleID"() -> (w2123:string)
        n1231 = Greater Than 0?(x=w2141) -> (x > 0?=w2142:bool)
        n1232 = Greater Than 0?(x=w2124) -> (x > 0?=w2143:bool)
        n1233 = Not Equal?(x=w2123, y="") -> (x != y?=w2121:bool)
        n1234 = Compound Arithmetic op=AND(w2143, w2142, w2121) -> (w2116:bool)
        n1235 = property on="mainTabCntrl" class="TabCtl (strict)"(error in=w2127) -> (error out=w2133:errorcluster, "Pages"=w2136:refnum<vi>[])  [unwired: 1 in, 1 out]
        n1236 = Not(x=w2116) -> (.not. x?=w2132:bool)
        n1237 = Index Array(array=w2136, index=1) -> (element=w2134:refnum<vi>)
        n1238 = Select(t=T16."Page Enabled" ("Page Enabled State"), s=w2116, f=T16."Page Disabled & Grayed" ("Page Enabled State")) -> (s? t:f=w2115:T16)
        n1239 = property on="Property Node" class="Page"(reference=w2134, error in=w2133, "PageEnb"=w2115) -> (error out=w2131:errorcluster)  [unwired: 1 out]
        n1240 = Select(t=T15."Enabled" ("Disabled"), s=w2116, f=T15."Disabled and Grayed Out" ("Disabled")) -> (s? t:f=w2113:T15)
        n1241 = property on="ARM" class="Bool"(error in=w2131, "Disabled"=w2113) -> (error out=w2139:errorcluster)  [unwired: 1 in, 1 out]
        n1242 = property on="addShot" class="Bool"(error in=w2139, "Disabled"=w2113) -> (error out=w2138:errorcluster)  [unwired: 1 in, 1 out]
        n1243 = property on="instruct_addShot" class="Str"(error in=w2138, "Visible"=w2132) -> (error out=w2137:errorcluster)  [unwired: 1 in, 1 out]
      }
      event "Mfr_1", "Mfr_2", "Mfr_3", "Mfr_4", "Mfr_5", "Mfr_6", "Mfr_0": Value Change {
        n1244 = event-data() -> ("CtlRef"=w2175:refnum<vi>)  [unwired: 1 out]
        n1245 = property on="Property Node" class="Ring (strict)"(reference=w2175, error in=w2167) -> (error out=w2165:errorcluster, "Label.Text"=w2171:string, "RingText.Text"=w2172:string)  [unwired: 1 out]
        n1246 = flat-sequence {
          tunnel: ["Mfr_1"] -> _
          tunnel: ["Mfr_2"] -> _
          tunnel: ["Mfr_3"] -> _
          tunnel: ["Mfr_4"] -> _
          tunnel: ["Mfr_5"] -> _
          tunnel: ["Mfr_6"] -> _
          frame #0 {
          }
        }
        n1247 = call "Select Sample Style.vi"("error IN"=w2165, "Mfr"=w2172) -> ("error Out"=w2164:errorcluster, "SampleStyles"=w2160:string[])  [unwired: 4 out]
        n1248 = Scan From String(format string="Mfr_%d", input string=w2171, error in=w2164, default 1=0 ("Mfr#")) -> (error out=w2161:errorcluster, output 1=w2170:i32)  [unwired: 1 in, 2 out]
        n1249 = case shown="1" w2170 {
          tunnel: [w2187 w2190 w2193 w2196 w2199 w2202 w2205] -> w2169
          tunnel: [w2186 w2189 w2192 w2195 w2198 w2201 w2204] -> w2162
          tunnel: w2161 -> [w2186 w2189 w2192 w2195 w2198 w2201 w2204]
          tunnel: w2160 -> [w2185 w2188 w2191 w2194 w2197 w2200 w2203]
          tunnel: [w2184 w2188 w2191 w2194 w2197 w2200 w2203] -> w2159
          frame 0, Default {
            n1250 = Delete From Array(array=w2185, length=1, index=0) -> (array with subset deleted=w2184:string[])  [unwired: 1 out]
            n1251 = control-ref of="SampleStyle_0"() -> (w2187:refnum<vi>)
          }
          frame 1 {
            n1252 = control-ref of="SampleStyle_1"() -> (w2190:refnum<vi>)
          }
          frame 2 {
            n1253 = control-ref of="SampleStyle_2"() -> (w2193:refnum<vi>)
          }
          frame 3 {
            n1254 = control-ref of="SampleStyle_3"() -> (w2196:refnum<vi>)
          }
          frame 4 {
            n1255 = control-ref of="SampleStyle_4"() -> (w2199:refnum<vi>)
          }
          frame 5 {
            n1256 = control-ref of="SampleStyle_5"() -> (w2202:refnum<vi>)
          }
          frame 6 {
            n1257 = control-ref of="SampleStyle_6"() -> (w2205:refnum<vi>)
          }
        }
        n1258 = property on="Property Node" class="Ring (strict)"(reference=w2169, error in=w2162, "Strings []"=w2159, "Val(Sgnl)"=u16 0 ("Value (Signaling)")) -> (error out=w2166:errorcluster)  [unwired: 1 out]
      }
      event "SampleStyle_1", "SampleStyle_2", "SampleStyle_3", "SampleStyle_4", "SampleStyle_5", "SampleStyle_6", "SampleStyle_0": Value Change {
        n1259 = event-data() -> ("CtlRef"=w2216:refnum<vi>)  [unwired: 1 out]
        n1260 = call "Get Sample Style Atributes.vi"("StyleNumRef"=w2216) -> ("SampleSpecs"=w2211:T41)  [unwired: 1 in]
        n1261 = flat-sequence {
          tunnel: ["SampleStyle_1"] -> _
          tunnel: ["SampleStyle_2"] -> _
          tunnel: ["SampleStyle_3"] -> _
          tunnel: ["SampleStyle_4"] -> _
          tunnel: ["SampleStyle_5"] -> _
          tunnel: ["SampleStyle_6"] -> _
          frame #0 {
          }
        }
        n1262 = property on="Property Node" class="Ring (strict)"(reference=w2216, error in=w2210) -> (error out=w2209:errorcluster, "Label.Text"=w2215:string)  [unwired: 1 out]
        n1263 = Scan From String(format string="SampleStyle_%d", input string=w2215, error in=w2209, default 1=0 ("default value 1")) -> (error out=w2208:errorcluster, output 1=w2213:i32)  [unwired: 1 in, 2 out]
        n1264 = case shown="0, Default" w2213 {
          tunnel: w2211 -> [w2225 w2228 w2231 w2234 w2237 w2240 w2243]
          tunnel: w2208 -> [w2224 w2227 w2230 w2233 w2236 w2239 w2242]
          tunnel: [w2223 w2226 w2229 w2232 w2235 w2238 w2241] -> w2207
          frame 0, Default {
            n1265 = property on="SampleAttribs_0" class="Clust (strict)"(error in=w2224, "Val(Sgnl)"=w2225) -> (error out=w2223:errorcluster)  [unwired: 1 in, 1 out]
            "SampleAttribs_0" <- w2225
          }
          frame 1 {
            n1266 = property on="SampleAttribs_1" class="Clust (strict)"(error in=w2227, "Val(Sgnl)"=w2228) -> (error out=w2226:errorcluster)  [unwired: 1 in, 1 out]
            "SampleAttribs_1" <- w2228
          }
          frame 2 {
            n1267 = property on="SampleAttribs_2" class="Clust (strict)"(error in=w2230, "Val(Sgnl)"=w2231) -> (error out=w2229:errorcluster)  [unwired: 1 in, 1 out]
            "SampleAttribs_2" <- w2231
          }
          frame 3 {
            n1268 = property on="SampleAttribs_3" class="Clust (strict)"(error in=w2233, "Val(Sgnl)"=w2234) -> (error out=w2232:errorcluster)  [unwired: 1 in, 1 out]
            "SampleAttribs_3" <- w2234
          }
          frame 4 {
            n1269 = property on="SampleAttribs_4" class="Clust (strict)"(error in=w2236, "Val(Sgnl)"=w2237) -> (error out=w2235:errorcluster)  [unwired: 1 in, 1 out]
            "SampleAttribs_4" <- w2237
          }
          frame 5 {
            n1270 = property on="SampleAttribs_5" class="Clust (strict)"(error in=w2239, "Val(Sgnl)"=w2240) -> (error out=w2238:errorcluster)  [unwired: 1 in, 1 out]
            "SampleAttribs_5" <- w2240
          }
          frame 6 {
            n1271 = property on="SampleAttribs_6" class="Clust (strict)"(error in=w2242, "Val(Sgnl)"=w2243) -> (error out=w2241:errorcluster)  [unwired: 1 in, 1 out]
            "SampleAttribs_6" <- w2243
          }
        }
      }
      event "SHOTS", "Sort by AVG": Value Change {
        n1272 = event-data() -> ()  [unwired: 2 out]
        n1273 = local read "Site"() -> (w2244:string)
        n1274 = local read "SHOTS"() -> (w2246:T7[])
        n1275 = call "Update Shot Table.vi"("Sort by AVG"="Sort by AVG", "Site"=w2244, "shotsArr"=w2246) -> ("shotTable OUT"=→"Table of Shots":string[][])
      }
      event "Layer_1", "Layer_2", "Layer_3", "Layer_4", "Layer_5", "Layer_6", "SampleAttribs_1.ozPerYd2", "SampleAttribs_2.ozPerYd2", "SampleAttribs_3.ozPerYd2", "SampleAttribs_4.ozPerYd2", "SampleAttribs_5.ozPerYd2", "SampleAttribs_6.ozPerYd2": Value Change {
        n1276 = event-data() -> ()  [unwired: 2 out]
        n1277 = global read "BIMS_Collector Globals.vi" "SampleAttribs"() -> (w2250:T24)
        n1278 = Build Array("Layer_1", "Layer_2", "Layer_3", "Layer_4", "Layer_5", "Layer_6") -> (w2253:T42)
        n1279 = global write "BIMS_Collector Globals.vi" "LayerSpecs"(w2253) -> ()
        n1280 = for {
          tunnel: w2253 -> [w2280] mode=indexing
          shift-right: [w2282] -> w2261
          shift-left: 0 -> [w2281]
          tunnel: [w2279] -> w2271 mode=indexing
          tunnel: w2250 -> [w2277] mode=indexing
          n1281 = Unbundle By Name(w2277) -> ("ozPerYd2"=w2273:string)
          n1282 = Equal?(x=w2273, y="" ("Empty String Constant")) -> (x = y?=w2272:bool)
          n1283 = case shown="False" w2272 {
            tunnel: [w2286 sgl 0.0 ("default value 1")] -> w2276
            tunnel: w2273 -> [w2283 _]
            frame False {
              n1284 = Scan From String(format string="%f", input string=w2283, default 1=sgl 0.0 ("default value 1")) -> (output 1=w2286:sgl)  [unwired: 2 in, 3 out]
            }
            frame True {
            }
          }
          n1285 = Unbundle By Name(w2280) -> ("plyNum"=w2278:i32)
          n1286 = Add(x=w2281, y=w2278) -> (x+y=w2282:i32)
          n1287 = To Single Precision Float(number=w2278) -> (single precision float=w2275:sgl)
          n1288 = Multiply(x=w2275, y=w2276) -> (x*y=w2279:sgl)
        }
        "totalNumLayers" <- w2261
        n1289 = Divide(x=w2271, y=sgl 144.0) -> (x/y=w2269:sgl[])
        n1290 = Index Array(array=w2269) -> (element #1=→"fab1_totalWt":sgl, element #2=→"fab2_totalWt":sgl, element #3=→"fab3_totalWt":sgl, element #4=→"fab4_totalWt":sgl, element #5=→"fab5_totalWt":sgl, element #6=→"fab6_totalWt":sgl)  [unwired: 6 in]
        n1291 = Add Array Elements(numeric array=w2269) -> (sum=→"totalBAW":sgl)
      }
      event "clayCalArray": Value Change {
        n1292 = event-data() -> ()  [unwired: 2 out]
        n1293 = for {
          tunnel: "clayCalArray" -> [w2315] mode=indexing
          shift-right: [w2314] -> w2297
          shift-left: "" ("Empty String Constant") -> [w2312]
          shift-right: [w2309] -> w2293
          shift-left: i16[] [] -> [w2308]
          n1294 = Greater Than 0?(x=w2315) -> (x > 0?=w2316:bool)
          n1295 = case shown="False" w2316 {
            tunnel: w2315 -> [_ w2322]
            tunnel: ["##" ("clayCalib") w2324] -> w2313
            tunnel: w2312 -> [w2319 w2323]
            tunnel: [w2319 w2323] -> w2311
            tunnel: [w2317 w2321] -> w2309
            tunnel: w2308 -> [w2317 w2320]
            frame False {
            }
            frame True {
              n1296 = Format Into String(w2322) -> (resulting string=w2324:string)  [unwired: 3 in, 1 out]
              n1297 = Build Array (concatenate)(w2320, w2322) -> (w2321:i16[])
            }
          }
          n1298 = Concatenate Strings(w2311, w2313, "-" ("string")) -> (w2314:string)
        }
        n1299 = String Length(string=w2297) -> (length=w2298:i32)
        n1300 = Add Array Elements(numeric array=w2293) -> (sum=w2302:i16)
        n1301 = Array Size(array=w2293) -> (size(s)=w2303:i32)
        n1302 = Decrement(x=w2298) -> (x-1=w2295:i32)
        n1303 = To Single Precision Float(number=w2302) -> (single precision float=w2301:sgl)
        n1304 = To Single Precision Float(number=w2303) -> (single precision float=w2291:sgl)
        n1305 = String Subset(string=w2297, length (rest)=w2295) -> (substring=w2296:string)  [unwired: 1 out]
        n1306 = Equal To 0?(x=w2291) -> (x = 0?=w2290:bool)
        n1307 = local write "clayCalib"(w2296) -> ()
        n1308 = case shown="True" w2290 {
          tunnel: w2301 -> [w2306 w2307]
          tunnel: w2291 -> [w2305 _]
          tunnel: [w2304 w2307] -> w2300
          frame False {
            n1309 = Divide(x=w2306, y=w2305) -> (x/y=w2304:sgl)
          }
          frame True {
          }
        }
        "clayAverage" <- w2300
      }
      event "reportV50_History": Value Change {
        n1310 = event-data() -> ()  [unwired: 2 out]
        n1311 = local write "lookupRec"(TRUE ("lookupRec")) -> ()
      }
      event "Methods": Value Change {
        n1312 = event-data() -> ("CtlRef"=w2334:refnum<vi>)  [unwired: 1 out]
        n1313 = call "Dropdown Selection (SubVI).vi"("reference"=w2334) -> ("element"=w2333:string)
        n1314 = Equal?(x=w2333, y="V50") -> (x = y?=w2331:bool)
        n1315 = property on="minV50" class="DigNum (strict)"(error in=w2330, "Visible"=w2331) -> (error out=w2329:errorcluster)  [unwired: 1 in, 1 out]
      }
      event "rangeSetup": Value Change {
        n1316 = event-data() -> ("NewVal"=w2344:u16)  [unwired: 1 out]
        n1317 = case shown="2" w2344 {
          tunnel: ["0" ("section") "5.0" ("section") "7.5" ("section") "45.0" ("section")] -> w2350
          frame 0, Default {
          }
          frame 1 {
          }
          frame 2 {
          }
          frame 3 {
          }
        }
        n1318 = local read "configPath"() -> (w2352:path)
        n1319 = local read "GrainSize"() -> (w2343:u16)
        n1320 = Greater Than 0?(x=w2344) -> (x > 0?=w2347:bool)
        n1321 = Greater Than 0?(x=w2343) -> (x > 0?=w2345:bool)
        n1322 = call <vilib>:"Open Config Data (compatibility).vi"("error in (no error)"=w2340, "configuration file path"=w2352) -> ("error out"=w2360:errorcluster, "refnum"=w2362:T36)  [unwired: 7 in, 1 out]
        n1323 = And(x=w2347, y=w2345) -> (x .and. y?=w2346:bool)
        n1324 = call-poly <vilib>:"Write Key.vi"("write raw string? (F)"=TRUE, "section"="Ballistic Parameters", "error in (no error)"=w2360, "value"=w2350, "key"="MidPoint To Target Distance", "refnum"=w2362) -> ("error out"=w2359:errorcluster, "refnum out"=w2358:T36)  [unwired: 4 out]
        n1325 = call <vilib>:"Close Config Data.vi"("error in (no error)"=w2359, "refnum"=w2358) -> ("error out"=w2351:errorcluster)  [unwired: 1 in, 8 out]
        n1326 = Not(x=w2346) -> (.not. x?=w2356:bool)
        n1327 = Select(t=u8 0 ("y"), s=w2346, f=u8 2 ("y")) -> (s? t:f=w2342:u8)
        n1328 = Scan From String(input string=w2350, error in=w2351, default 1=sgl 0.0 ("default value 1")) -> (error out=w2339:errorcluster, output 1=w2349:sgl)  [unwired: 2 in, 2 out]
        n1329 = local write "mid_to_targ_dist"(w2349) -> ()
        n1330 = property on="ARM" class="Bool"(error in=w2339, "Disabled"=w2342) -> (error out=w2338:errorcluster)  [unwired: 1 in, 1 out]
        n1331 = property on="addShot" class="Bool"(error in=w2338, "Disabled"=w2342) -> (error out=w2337:errorcluster)  [unwired: 1 in, 1 out]
        n1332 = property on="instruct_addShot" class="Str"(error in=w2337, "Visible"=w2356) -> (error out=w2336:errorcluster)  [unwired: 1 in, 1 out]
        "instruct_addShot" <- "RANGE SETUP and THREAT must be selected before shots can be added." ("instruct_addShot")
      }
      event "Drag Corrected", "maxDev": Value Change {
        n1333 = event-data() -> ()  [unwired: 2 out]
        n1334 = local write "processShots"(TRUE ("ProcessShots")) -> ()
      }
      event "2ndScreen": Value Change {
        n1335 = event-data() -> ()  [unwired: 7 out]
        n1336 = Select(t=T15."Enabled" ("Disabled"), s="2ndScreen", f=T15."Disabled and Grayed Out" ("Disabled")) -> (s? t:f=w2370:T15)
        n1337 = property on="MeasVelScrnSet2" class="DigNum (strict)"("DisabledEnum"=w2370) -> ()  [unwired: 2 in, 2 out]
        n1338 = property on="Redundant/speed" class="DigNum (strict)"("DisabledEnum"=w2370) -> ()  [unwired: 2 in, 2 out]
      }
      event "MC Listbox of Shots": Mouse Up {
        n1339 = event-data() -> ()  [unwired: 2 out]
        n1340 = flat-sequence {
          tunnel: w2380 -> [w2384]
          tunnel: [w2382] -> w2379
          tunnel: ["MC Listbox of Shots"] -> w2376
          tunnel: w2379 -> [w2388]
          tunnel: [w2387] -> w2378
          tunnel: w2376 -> [_]
          tunnel: w2378 -> [w2393]
          tunnel: [w2391] -> w2377
          frame #0 {
            n1341 = property on="Table of Shots" class="Tbl (strict)"(error in=w2384) -> (error out=w2383:errorcluster, "Value"=w2385:string[][])  [unwired: 1 in, 1 out]
            n1342 = local write "STOP (Shots MC LB)"(FALSE ("STOP (Shots MC LB)")) -> ()
            n1343 = property on="MC Listbox of Shots" class="MCListbox (strict)"(error in=w2383, "ItemNames"=w2385) -> (error out=w2382:errorcluster)  [unwired: 1 in, 1 out]
          }
          frame #1 {
            n1344 = control-ref of="MC Listbox of Shots"() -> (w2390:refnum<vi>)
            n1345 = control-ref of="STOP (Shots MC LB)"() -> (w2389:refnum<vi>)
            n1346 = call "multicolumn listbox sort.vi"("error IN"=w2388, "Bool Refnum"=w2389, "MCListbox Refnum"=w2390) -> ("error out"=w2387:errorcluster)  [unwired: 4 in]
          }
          frame #2 {
            n1347 = property on="MC Listbox of Shots" class="MCListbox (strict)"(error in=w2393) -> (error out=w2392:errorcluster, "ItemNames"=w2394:string[][])  [unwired: 1 in, 1 out]
            n1348 = property on="Table of Shots" class="Tbl (strict)"(error in=w2392, "Val(Sgnl)"=w2394) -> (error out=w2391:errorcluster)  [unwired: 1 in, 1 out]
          }
        }
      }
      event "PublishNewRecords": Value Change {
        w2400 = "\\" ("string")
        w2411 = TRUE  # overwrite (F)
        # "2. INSERT new records to Experiments and  \n      Shots tables in local Export.mdb file."
        # "1. SELECT new records from local MDB \n     by comparing against last record numbers \n     found in IMPORT table on BIMS server."
        # "Pushes latest ballistics performance data up to BIMS Server\n\n - Attempts connection with server (reports connection success in msgbox)\n - If successful:\n   - Exports all experiment/shot records since last table marker to [site].mdb file\n   - Sends export.mdb file to drop location on BIMS File Server\n   - Executes SSIS package to import records from export.mdb file\n - Otherwise provides option to try again or cancel"
        # "3. Copy Export.mdb file to [sitename].mdb in [sitename] \n      FileDrop folder on BIMS server."
        n1349 = event-data() -> ()  [unwired: 2 out]
        n1350 = property on="Loading" class="Ring (strict)"(error in=w2406, "Visible"=TRUE) -> (error out=w2405:errorcluster)  [unwired: 1 in, 1 out]
        n1351 = local read "Site"() -> (w2395:string)
        n1352 = call "Export New Records.vi"("error IN"=w2405, "Site"=w2395) -> ("error out"=w2413:errorcluster)  [unwired: 3 in, 6 out]
        n1353 = Concatenate Strings("\\\\" ("string"), "Server", w2400, "Folder", w2400, w2395, ".mdb" ("string")) -> (w2396:string)
        n1354 = String To Path(string=w2396) -> (path=w2409:path)
        n1355 = Copy(8:w2413, 9:w2411, 10:w2409, 11:path "C:/Ballistics/Export.mdb" ("source path")) -> (0:w2410:errorcluster)  [unwired: 3 out]
        n1356 = case shown="No Error" w2410 {
          selector: w2410 -> [w2415 w2417]
          tunnel: [w2415 w2416] -> w2404
          frame No Error {
            n1357 = One Button Dialog(message="New sample performance records submitted \nto BIMS Warehouse successfully.\n\nPublishing will occur in under five minutes.") -> ()  [unwired: 2 out]
          }
          frame Error {
            n1358 = call <vilib>:"General Error Handler.vi"("error in (no error)"=w2417) -> ("error out"=w2416:errorcluster)  [unwired: 2 in, 12 out]
          }
        }
        n1359 = property on="Loading" class="Ring (strict)"(error in=w2404, "Visible"=FALSE) -> (error out=w2403:errorcluster)  [unwired: 1 in, 1 out]
      }
      event "arrIDC": Mouse Up {
        n1360 = event-data() -> ()  [unwired: 2 out]
        "velProfile" <- cluster{dbl, dbl}[] [] ("velProfile")
        "arrIDC" <- dbl[] [] ("arrIDC")
        "relativeTime" <- cluster{"ts2":dbl, "ts3":dbl, "ts1":dbl} {"ts2"=0.0, "ts3"=0.0, "ts1"=0.0} ("relativeTime")
        "velMeasProf" <- T8 {"v2"=0.0, "vB"=0.0, "vOuter"=0.0, "v1"=0.0, "vA"=0.0, "vInner"=0.0} ("velMeasProf")
        "velCompProf" <- cluster{"vStrike":dbl, "vA":dbl} {"vStrike"=0.0, "vA"=0.0} ("velCompProf")
        "displacement" <- T9 {"ds_v2"=6.75, "ds2"=5.0833, "ds_vB"=4.9167, "ds3"=4.75, "ds_vAvg"=6.9167, "ds_v1"=7.0833, "ds1"=8.75, "ds_vA"=8.9167, "ds0"=9.0833} ("displacement")
      }
      event "SampleBackings": Value Change {
        # "Clay is the default sample backing material.\n\n  If another selection is made, then grey out and disable all controls relating to clay."
        n1361 = event-data() -> ()  [unwired: 2 out]
        n1362 = case shown="0, Default" "SampleBackings" {
          tunnel: [T15."Disabled and Grayed Out" ("Disabled") T15."Enabled" ("Disabled") T15."Disabled and Grayed Out" ("Disabled")] -> w2426
          frame 0, Default {
          }
          frame 1 {
          }
          frame 2.. {
          }
        }
        n1363 = property on="clayCalArray" class="Arr (strict)"("DisabledEnum"=w2426) -> ()  [unwired: 2 in, 2 out]
        n1364 = property on="clayAverage" class="DigNum (strict)"("DisabledEnum"=w2426) -> ()  [unwired: 2 in, 2 out]
        n1365 = property on="clayTemp" class="DigNum (strict)"("DisabledEnum"=w2426) -> ()  [unwired: 2 in, 2 out]
      }
      event "RefreshMetadata": Value Change {
        # "Pulls latest metadata down from BIMS Database Server\n - Attempts connection with server \n        (reports failure if connection is unsuccessful)\n - If successful:\n   - Updates local database records from server\n   - Updates dropdown listboxes from local database"
        n1366 = event-data() -> ()  [unwired: 2 out]
        n1367 = property on="Loading" class="Ring (strict)"(error in=w2456, "Visible"=TRUE) -> (error out=w2455:errorcluster)  [unwired: 1 in, 1 out]
        n1368 = control-ref of="LayerStitchTypes"() -> (w2440:refnum<vi>)
        n1369 = control-ref of="BackLayer"() -> (w2451:refnum<vi>)
        n1370 = control-ref of="FrontLayer"() -> (w2452:refnum<vi>)
        n1371 = control-ref of="ThreatGroups"() -> (w2453:refnum<vi>)
        n1372 = control-ref of="SampleClamping"() -> (w2461:refnum<vi>)
        n1373 = control-ref of="SampleTypes"() -> (w2478:refnum<vi>)
        n1374 = control-ref of="SampleDimensions"() -> (w2477:refnum<vi>)
        n1375 = control-ref of="ModelMfrs"() -> (w2476:refnum<vi>)
        n1376 = control-ref of="Assemblers"() -> (w2475:refnum<vi>)
        n1377 = control-ref of="Submitters"() -> (w2474:refnum<vi>)
        n1378 = control-ref of="PowderTypes"() -> (w2473:refnum<vi>)
        n1379 = control-ref of="Methods"() -> (w2470:refnum<vi>)
        n1380 = control-ref of="TestConditions"() -> (w2469:refnum<vi>)
        n1381 = control-ref of="SampleBackings"() -> (w2468:refnum<vi>)
        n1382 = control-ref of="Ballisticians"() -> (w2467:refnum<vi>)
        n1383 = control-ref of="Shooters"() -> (w2466:refnum<vi>)
        n1384 = control-ref of="Recorders"() -> (w2465:refnum<vi>)
        n1385 = Build Array(w2440, w2451, w2452, w2453, w2461, w2478, w2477, w2476, w2475, w2474, w2473, w2470, w2469, w2468, w2467, w2466, w2465) -> (w2472:refnum<vi>[])
        n1386 = call "Update Metadata using listbox names.vi"("error in"=w2455, "Site"="Site", "RefNumArrIn"=w2472) -> ("error out"=w2479:errorcluster, "RefNumArrOut"=w2471:refnum<vi>[])  [unwired: 1 in, 6 out]
        n1387 = call "Fill Lists from DB (1st Pass).vi"("error in"=w2479, "RefNumArray"=w2471) -> ("error out"=w2441:errorcluster)  [unwired: 1 in, 4 out]
        n1388 = call "Fill Stitch Lists.vi"("error IN"=w2441) -> ("error OUT"=w2436:errorcluster)  [unwired: 6 in]
        n1389 = control-ref of="ThreatSize_0"() -> (w2434:refnum<vi>)
        n1390 = control-ref of="Requestors_0"() -> (w2439:refnum<vi>)
        n1391 = Build Array(w2434, w2439) -> (w2438:refnum<vi>[])
        n1392 = call "Fill Lists from DB (2nd Pass).vi"("errorIN"=w2436, "colNames"=string[] ["GrainSize", "requestor"] ("lkupTableNames"), "lkupTableNames"=string[] ["ThreatDetails", "Submitters"], "RefNumArray"=w2438) -> ("error OUT"=w2435:errorcluster)  [unwired: 3 in]
        n1393 = flat-sequence {
          frame #0 {
            n1394 = local write "RefreshMetadata"(FALSE ("UpdateMetadata")) -> ()
            n1395 = local write "TimeNow"("Connecting to BIMS Server . . ." ("TimeNow")) -> ()
          }
        }
        n1396 = call "Create local tables from Server DB.vi"("error in"=w2435, "Site"="Site", "tableNames"=string[] ["Threats", "ThreatDetails", "ThreatCalibers", "Mfrs", "SampleStyles", "SampleSpecs", "FiberTypes"]) -> ("error out"=w2463:errorcluster)  [unwired: 1 in, 7 out]
        n1397 = call "Fill Lists From DB (3rd Pass).vi"("error IN"=w2463) -> ("error OUT"=w2443:errorcluster)  [unwired: 3 in, 3 out]
        n1398 = control-ref of="ModelMfrs"() -> (w2450:refnum<vi>)
        n1399 = property class="Ring (strict)"(reference=w2450, error in=w2443) -> (reference out=w2449:refnum<vi>, error out=w2448:errorcluster, "Strings []"=w2447:string[])
        n1400 = Delete From Array(array=w2447, length=1, index=0) -> (array with subset deleted=w2446:string[])  [unwired: 1 out]
        n1401 = property class="Ring (strict)"(reference=w2449, error in=w2448, "Strings []"=w2446) -> (error out=w2442:errorcluster)  [unwired: 1 out]
        n1402 = case shown="No Error" w2442 {
          selector: w2442 -> [w2480 w2483]
          tunnel: [w2480 w2483] -> w2459
          frame No Error {
            n1403 = local write "TimeNow"("Collector Metadata is READY!" ("TimeNow")) -> ()
            n1404 = Wait (ms)(milliseconds to wait=u32 2000) -> ()  [unwired: 1 out]
          }
          frame Error {
            n1405 = call <vilib>:"General Error Handler.vi"("error in (no error)"=w2483) -> ()  [unwired: 2 in, 13 out]
          }
        }
        n1406 = property on="Loading" class="Ring (strict)"(error in=w2459, "Visible"=FALSE) -> (error out=w2458:errorcluster)  [unwired: 1 in, 1 out]
      }
      event "loadingUnits": Value Change {
        n1407 = local read "Powder Loading"() -> (w2487:sgl)
        n1408 = event-data() -> ("NewVal"=w2486:enum32{"grams", "grains"})  [unwired: 6 out]
        n1409 = case shown="\"grams\", Default" w2486 {
          tunnel: w2487 -> [w2492 w2493]
          frame "grams", Default {
            n1410 = Multiply(x=w2492, y=sgl 0.06479891) -> (x*y=w2490:sgl)
            n1411 = local write "Powder Loading"(w2490) -> ()
          }
          frame "grains" {
            n1412 = Multiply(x=w2493, y=sgl 15.432359) -> (x*y=w2494:sgl)
            n1413 = local write "Powder Loading"(w2494) -> ()
          }
        }
      }
      event "clearErrors": Value Change {
        w2496 = errorcluster {"status"=FALSE, "code"=0, "source"=""} ("error in")
        n1414 = event-data() -> ()  [unwired: 7 out]
        n1415 = local write "SMErr"(w2496) -> ()
      }
    }
    "U/I EvErr" <- w1981
    "booleanDump" <- w1980
  }
